vi "Telemetry.vi"() -> ()   [LabVIEW 2017]
uses:
  <vilib>/Platform/TimedLoop/XDataNode/timing_clust.ctl
  <vilib>/Platform/TimedLoop/XDataNode/nitl_modes.ctl
  <vilib>/Platform/TimedLoop/XDataNode/wakeup.ctl
  <vilib>/nican/nican.llb/ncNetAttr.ctl
  <vilib>/Utility/file.llb/Read From Spreadsheet File (string).vi
  <vilib>/xnet/xnet.llb/XNET Create Session (Frame Input Stream).vi
  <vilib>/xnet/xnet.llb/XNET Read (Frame CAN).vi
  <vilib>/Utility/file.llb/Write To Spreadsheet File (string).vi
  <vilib>/Platform/TimedLoop/XDataNode/XDataNode.xnode
  <resource>/objmgr/xnet.rc
  <vilib>/Platform/TimedLoop/XDataNode/XDNodeRunTimeDep.lvlib
panel:
  out "Traction Control ON":bool
  out "Torque Demand [Nm]":dbl
  out "BP_rear":i16
  out "BP_front":i16
  out "Front / Rear Brake Pressure":cluster{u16, u16}
  out "Regbrake Front Sum [Nm]":dbl
  out "Regbrake Rear Sum [Nm]":dbl
  out "BrakeForce":u16
  out "Cones3 2":T1(array[cluster])
  out "Cones2 2":T1(array[cluster])
  out "Cones1 2":T1(array[cluster])
  out "(hi.lo) 3":u64 format="%064b"
  out "Cones3":T1(array[cluster])
  out "(hi.lo) 2":u64 format="%064b"
  out "Cones2":T1(array[cluster])
  in  "ConeType":cluster{"Col":dbl, "X":dbl, "Y":dbl}
  out "(hi.lo)":u64 format="%064b"
  out "Cones1":T1(array[cluster])
  out "IGBT Temperature":T2(graph)
  out "Numeric 2":u8
  out "Slope":u16
  out "Damper Travel FR [mm]":dbl
  out "Damper Travel RR [mm]":dbl
  out "Damper Travel FL [mm]":dbl
  in  "Wheel Travel FR":dbl=1000.0
  in  "Wheel Travel FL Offset":dbl=1000.0
  in  "Wheel Travel RR Offset":dbl=1000.0
  out "Damper Travel RL [mm]":dbl
  in  "Wheel Travel RL Offset":dbl=1000.0
  out "HV Cell Voltage":u16(graph)
  out "accY 2":dbl
  out "accZ 2":dbl
  out "TorqRaw 2":u16
  in  "Brake Min 3":dbl=426.0
  out "BPRV":bool
  out "BPFV":bool
  out "BPFV":bool
  out "BPFSV":bool
  out "STA2":bool
  out "STA1":bool
  out "TPS2V":bool
  out "TPS1V":bool
  out "Apps2":dbl
  out "Apps1":dbl
  out "APPS1":u8(slide) scale=0.0..100.0
  out "APPS2":u8(slide) scale=0.0..100.0
  out "Brake Pedal Fore Supply":dbl
  out "Status LEDs Red":bool[](array[boolean])
  out "Status LEDs Green":bool[](array[boolean])
  out "Numeric":dbl
  out "TCU speed":cluster{dbl, "AccelXRaw":dbl, dbl}(graph)
  out "AccelYRaw":dbl
  out "AccelXRaw":dbl
  in  "Acc Y offset":dbl
  in  "Acc X offset 2":dbl
  in  "OffsetFilter":dbl=0.01
  out "IsStopped":bool
  out "Acc Z 2":dbl
  out "Acc X 2":dbl
  out "Roll 2":dbl
  out "Acc Y 2":dbl
  out "Yaw 2":dbl
  in  "Acc Z offset":dbl
  out "Vel_acc":dbl=-0.0098098
  in  "New Lap":bool
  out "Energy":dbl[](array[numeric])
  out "Wheel Travel FL":u16
  out "Wheel Travel FR":u16
  out "Wheel Travel RL":u16
  out "Wheel Travel RR":u16
  out "Acc X":dbl
  out "Roll":dbl
  out "Yaw":dbl
  out "Acc Y":dbl
  out "Acc Z":dbl
  out "accY":dbl
  out "accZ":dbl
  out "Intensity Graph":dbl[][](graph)
  in  "Rollrate offset":dbl
  out "XY Graph 2":cluster{dbl[], dbl[]}(graph)
  out "Torq_sum":dbl
  in  "Play":bool
  in  "Timestep":u32
  in  "stop":bool
  in  "start":bool
  in  "pause":bool
  in  "Progress":i32(slide) min=0 step=60 scale=-1.0..61354011.0 scale format="%.0p"
  out "Time Stamp":string="2\r\n60"
  out "Charge Voltage":dbl
  out "Charge Curr":dbl
  in  "Tab Control":T3(tab)
  in  "Rows to read":i32=60
  in  "Data Path":path=path "D:/__BME-FRT/2016/2016-05-19/2016_05_19_tokol_endurance_00005_00001.csv"
  in  "CAN1 Enable":bool
  in  "CAN0 Enable":bool
  in  "Data Source":u16(ring) items=["Wi-Fi", "CAN-USB", "Log Analysis", "XCAN-USB"]
  in  "Port":u16=8998
  in  "Exit":bool
  in  "Log Path":path=path "D:/__BME-FRT/2016/test.txt"
  in  "Log Enable":bool
  out "WiFi Error":errorcluster
  in  "Length":u16=10
  out "CAN0 Error":errorcluster
  out "CAN1 Error":errorcluster
  out "Log Error":errorcluster
  out "CAN Message":u8[][](array[numeric])=[[2, 1, 128, 63, 0, 0, 129, 162, 129, 155], [2, 17, 23, 61, 0, 1, 0, 0, 0, 0], [3, 64, 252, 0, 0, 0, 27, 55, 27, 0], [2, 16, 115, 16, 37, 0, 203, 0, 0, 0], [4, 17, 23, 61, 0, 1, 0, 0, 0, 0], [2, 0, 128, 44, 0, 0, 136, 1, 7, 207], [2, 1, 128, 63, 0, 0, 129, 162, 129, 155], [2, 17, 23, 61, 0, 1, 0, 0, 0, 0], [4, 34, 0, 33, 0, 30, 0, 0, 0, 0], [4, 80, 148, 60, 128, 0, 0, 0, 0, 0], [1, 116, 84, 128, 0, 0, 190, 127, 8, 37], [2, 16, 116, 15, 111, 0, 203, 0, 0, 0], [1, 120, 211, 127, 0, 0, 193, 158, 8, 215], [1, 180, 84, 128, 0, 0, 223, 126, 2, 100], [1, 124, 0, 0, 0, 0, 189, 126, 8, 75], [1, 184, 62, 128, 2, 15, 59, 127, 2, 219], [4, 17, 23, 61, 0, 1, 0, 0, 0, 0], [1, 188, 0, 0, 0, 0, 136, 158, 2, 110], [2, 0, 128, 44, 0, 0, 136, 1, 7, 207], [2, 1, 128, 63, 0, 0, 129, 162, 129, 155], [2, 17, 23, 61, 0, 1, 0, 0, 0, 0], [3, 64, 252, 0, 0, 0, 27, 55, 27, 0], [4, 48, 10, 15, 219, 0, 96, 0, 0, 0], [3, 49, 128, 255, 0, 0, 0, 0, 0, 0], [2, 16, 117, 0, 0, 0, 203, 0, 0, 0], [4, 17, 23, 61, 0, 1, 0, 0, 0, 0], [2, 0, 128, 44, 0, 0, 136, 1, 7, 207], [2, 1, 128, 63, 0, 0, 129, 162, 129, 155], [2, 17, 23, 61, 0, 1, 0, 0, 0, 0], [3, 32, 112, 255, 0, 0, 0, 0, 0, 0], [4, 34, 0, 30, 0, 31, 0, 0, 0, 0], [1, 116, 87, 128, 0, 0, 184, 127, 9, 218], [1, 120, 203, 127, 1, 37, 194, 158, 9, 222], [2, 16, 118, 0, 0, 0, 205, 0, 0, 0], [1, 124, 0, 0, 0, 0, 176, 126, 9, 211], [1, 180, 90, 128, 0, 0, 215, 126, 3, 116], [1, 184, 50, 128, 3, 19, 44, 127, 3, 114], [4, 17, 23, 61, 0, 1, 0, 0, 0, 0], [1, 188, 0, 0, 0, 0, 147, 158, 3, 235], [2, 0, 128, 43, 0, 0, 136, 1, 7, 207], [2, 1, 128, 63, 0, 0, 129, 162, 129, 155], [2, 17, 23, 61, 0, 1, 0, 0, 0, 0], [3, 64, 252, 0, 0, 0, 38, 55, 38, 0], [2, 16, 119, 0, 0, 0, 202, 0, 0, 0], [4, 17, 23, 61, 0, 1, 0, 0, 0, 0], [2, 0, 128, 43, 0, 0, 136, 2, 7, 207], [2, 1, 128, 63, 0, 0, 129, 162, 129, 155], [2, 17, 23, 61, 0, 1, 0, 0, 0, 0], [4, 34, 0, 20, 0, 26, 0, 0, 0, 0], [1, 116, 78, 128, 0, 0, 179, 127, 10, 75], [1, 120, 206, 127, 2, 57, 194, 158, 10, 132], [2, 16, 120, 16, 37, 0, 200, 0, 210, 0], [1, 180, 90, 128, 0, 0, 206, 126, 4, 188], [1, 124, 0, 0, 0, 0, 157, 126, 10, 65], [1, 184, 39, 128, 4, 3, 33, 127, 4, 7], [4, 17, 23, 61, 0, 1, 0, 0, 0, 0], [1, 188, 0, 0, 0, 0, 153, 158, 4, 183], [2, 0, 128, 43, 0, 0, 136, 2, 7, 207], [2, 1, 128, 63, 0, 0, 129, 162, 129, 155], [2, 17, 23, 61, 0, 1, 0, 0, 0, 0]] format="%02x"
  out "CAN ID":u16[](array[numeric])=[513, 529, 832, 528, 1041, 512, 513, 529, 1058, 1104, 372, 528, 376, 436, 380, 440, 1041, 444, 512, 513, 529, 832, 1072, 817, 528, 1041, 512, 513, 529, 800, 1058, 372, 376, 528, 380, 436, 440, 1041, 444, 512, 513, 529, 832, 528, 1041, 512, 513, 529, 1058, 372, 376, 528, 436, 380, 440, 1041, 444, 512, 513, 529] format="%x"
  out "CAN Message 2":u8[][](array[numeric])=[[2, 1, 128, 63, 0, 0, 129, 162, 129, 155], [2, 17, 23, 61, 0, 1, 0, 0, 0, 0], [3, 64, 252, 0, 0, 0, 27, 55, 27, 0], [2, 16, 115, 16, 37, 0, 203, 0, 0, 0], [4, 17, 23, 61, 0, 1, 0, 0, 0, 0], [2, 0, 128, 44, 0, 0, 136, 1, 7, 207], [2, 1, 128, 63, 0, 0, 129, 162, 129, 155], [2, 17, 23, 61, 0, 1, 0, 0, 0, 0], [4, 34, 0, 33, 0, 30, 0, 0, 0, 0], [4, 80, 148, 60, 128, 0, 0, 0, 0, 0], [1, 116, 84, 128, 0, 0, 190, 127, 8, 37], [2, 16, 116, 15, 111, 0, 203, 0, 0, 0], [1, 120, 211, 127, 0, 0, 193, 158, 8, 215], [1, 180, 84, 128, 0, 0, 223, 126, 2, 100], [1, 124, 0, 0, 0, 0, 189, 126, 8, 75], [1, 184, 62, 128, 2, 15, 59, 127, 2, 219], [4, 17, 23, 61, 0, 1, 0, 0, 0, 0], [1, 188, 0, 0, 0, 0, 136, 158, 2, 110], [2, 0, 128, 44, 0, 0, 136, 1, 7, 207], [2, 1, 128, 63, 0, 0, 129, 162, 129, 155], [2, 17, 23, 61, 0, 1, 0, 0, 0, 0], [3, 64, 252, 0, 0, 0, 27, 55, 27, 0], [4, 48, 10, 15, 219, 0, 96, 0, 0, 0], [3, 49, 128, 255, 0, 0, 0, 0, 0, 0], [2, 16, 117, 0, 0, 0, 203, 0, 0, 0], [4, 17, 23, 61, 0, 1, 0, 0, 0, 0], [2, 0, 128, 44, 0, 0, 136, 1, 7, 207], [2, 1, 128, 63, 0, 0, 129, 162, 129, 155], [2, 17, 23, 61, 0, 1, 0, 0, 0, 0], [3, 32, 112, 255, 0, 0, 0, 0, 0, 0], [4, 34, 0, 30, 0, 31, 0, 0, 0, 0], [1, 116, 87, 128, 0, 0, 184, 127, 9, 218], [1, 120, 203, 127, 1, 37, 194, 158, 9, 222], [2, 16, 118, 0, 0, 0, 205, 0, 0, 0], [1, 124, 0, 0, 0, 0, 176, 126, 9, 211], [1, 180, 90, 128, 0, 0, 215, 126, 3, 116], [1, 184, 50, 128, 3, 19, 44, 127, 3, 114], [4, 17, 23, 61, 0, 1, 0, 0, 0, 0], [1, 188, 0, 0, 0, 0, 147, 158, 3, 235], [2, 0, 128, 43, 0, 0, 136, 1, 7, 207], [2, 1, 128, 63, 0, 0, 129, 162, 129, 155], [2, 17, 23, 61, 0, 1, 0, 0, 0, 0], [3, 64, 252, 0, 0, 0, 38, 55, 38, 0], [2, 16, 119, 0, 0, 0, 202, 0, 0, 0], [4, 17, 23, 61, 0, 1, 0, 0, 0, 0], [2, 0, 128, 43, 0, 0, 136, 2, 7, 207], [2, 1, 128, 63, 0, 0, 129, 162, 129, 155], [2, 17, 23, 61, 0, 1, 0, 0, 0, 0], [4, 34, 0, 20, 0, 26, 0, 0, 0, 0], [1, 116, 78, 128, 0, 0, 179, 127, 10, 75], [1, 120, 206, 127, 2, 57, 194, 158, 10, 132], [2, 16, 120, 16, 37, 0, 200, 0, 210, 0], [1, 180, 90, 128, 0, 0, 206, 126, 4, 188], [1, 124, 0, 0, 0, 0, 157, 126, 10, 65], [1, 184, 39, 128, 4, 3, 33, 127, 4, 7], [4, 17, 23, 61, 0, 1, 0, 0, 0, 0], [1, 188, 0, 0, 0, 0, 153, 158, 4, 183], [2, 0, 128, 43, 0, 0, 136, 2, 7, 207], [2, 1, 128, 63, 0, 0, 129, 162, 129, 155], [2, 17, 23, 61, 0, 1, 0, 0, 0, 0]] format="%02x"
  out "CAN ID 2":u16[](array[numeric])=[513, 529, 832, 528, 1041, 512, 513, 529, 1058, 1104, 372, 528, 376, 436, 380, 440, 1041, 444, 512, 513, 529, 832, 1072, 817, 528, 1041, 512, 513, 529, 800, 1058, 372, 376, 528, 380, 436, 440, 1041, 444, 512, 513, 529, 832, 528, 1041, 512, 513, 529, 1058, 372, 376, 528, 436, 380, 440, 1041, 444, 512, 513, 529] format="%x"
  out "CAN Message 3":u8[][](array[numeric])=[[2, 1, 128, 63, 0, 0, 129, 162, 129, 155], [2, 17, 23, 61, 0, 1, 0, 0, 0, 0], [3, 64, 252, 0, 0, 0, 27, 55, 27, 0], [2, 16, 115, 16, 37, 0, 203, 0, 0, 0], [4, 17, 23, 61, 0, 1, 0, 0, 0, 0], [2, 0, 128, 44, 0, 0, 136, 1, 7, 207], [2, 1, 128, 63, 0, 0, 129, 162, 129, 155], [2, 17, 23, 61, 0, 1, 0, 0, 0, 0], [4, 34, 0, 33, 0, 30, 0, 0, 0, 0], [4, 80, 148, 60, 128, 0, 0, 0, 0, 0], [1, 116, 84, 128, 0, 0, 190, 127, 8, 37], [2, 16, 116, 15, 111, 0, 203, 0, 0, 0], [1, 120, 211, 127, 0, 0, 193, 158, 8, 215], [1, 180, 84, 128, 0, 0, 223, 126, 2, 100], [1, 124, 0, 0, 0, 0, 189, 126, 8, 75], [1, 184, 62, 128, 2, 15, 59, 127, 2, 219], [4, 17, 23, 61, 0, 1, 0, 0, 0, 0], [1, 188, 0, 0, 0, 0, 136, 158, 2, 110], [2, 0, 128, 44, 0, 0, 136, 1, 7, 207], [2, 1, 128, 63, 0, 0, 129, 162, 129, 155], [2, 17, 23, 61, 0, 1, 0, 0, 0, 0], [3, 64, 252, 0, 0, 0, 27, 55, 27, 0], [4, 48, 10, 15, 219, 0, 96, 0, 0, 0], [3, 49, 128, 255, 0, 0, 0, 0, 0, 0], [2, 16, 117, 0, 0, 0, 203, 0, 0, 0], [4, 17, 23, 61, 0, 1, 0, 0, 0, 0], [2, 0, 128, 44, 0, 0, 136, 1, 7, 207], [2, 1, 128, 63, 0, 0, 129, 162, 129, 155], [2, 17, 23, 61, 0, 1, 0, 0, 0, 0], [3, 32, 112, 255, 0, 0, 0, 0, 0, 0], [4, 34, 0, 30, 0, 31, 0, 0, 0, 0], [1, 116, 87, 128, 0, 0, 184, 127, 9, 218], [1, 120, 203, 127, 1, 37, 194, 158, 9, 222], [2, 16, 118, 0, 0, 0, 205, 0, 0, 0], [1, 124, 0, 0, 0, 0, 176, 126, 9, 211], [1, 180, 90, 128, 0, 0, 215, 126, 3, 116], [1, 184, 50, 128, 3, 19, 44, 127, 3, 114], [4, 17, 23, 61, 0, 1, 0, 0, 0, 0], [1, 188, 0, 0, 0, 0, 147, 158, 3, 235], [2, 0, 128, 43, 0, 0, 136, 1, 7, 207], [2, 1, 128, 63, 0, 0, 129, 162, 129, 155], [2, 17, 23, 61, 0, 1, 0, 0, 0, 0], [3, 64, 252, 0, 0, 0, 38, 55, 38, 0], [2, 16, 119, 0, 0, 0, 202, 0, 0, 0], [4, 17, 23, 61, 0, 1, 0, 0, 0, 0], [2, 0, 128, 43, 0, 0, 136, 2, 7, 207], [2, 1, 128, 63, 0, 0, 129, 162, 129, 155], [2, 17, 23, 61, 0, 1, 0, 0, 0, 0], [4, 34, 0, 20, 0, 26, 0, 0, 0, 0], [1, 116, 78, 128, 0, 0, 179, 127, 10, 75], [1, 120, 206, 127, 2, 57, 194, 158, 10, 132], [2, 16, 120, 16, 37, 0, 200, 0, 210, 0], [1, 180, 90, 128, 0, 0, 206, 126, 4, 188], [1, 124, 0, 0, 0, 0, 157, 126, 10, 65], [1, 184, 39, 128, 4, 3, 33, 127, 4, 7], [4, 17, 23, 61, 0, 1, 0, 0, 0, 0], [1, 188, 0, 0, 0, 0, 153, 158, 4, 183], [2, 0, 128, 43, 0, 0, 136, 2, 7, 207], [2, 1, 128, 63, 0, 0, 129, 162, 129, 155], [2, 17, 23, 61, 0, 1, 0, 0, 0, 0]] format="%02x"
  out "CAN ID 3":u16[](array[numeric])=[513, 529, 832, 528, 1041, 512, 513, 529, 1058, 1104, 372, 528, 376, 436, 380, 440, 1041, 444, 512, 513, 529, 832, 1072, 817, 528, 1041, 512, 513, 529, 800, 1058, 372, 376, 528, 380, 436, 440, 1041, 444, 512, 513, 529, 832, 528, 1041, 512, 513, 529, 1058, 372, 376, 528, 436, 380, 440, 1041, 444, 512, 513, 529] format="%x"
  out "Max RPM":u16
  out "Throttle Bias Front":dbl
  out "STA2":i16
  out "STA1":i16
  out "Max Power":u8
  out "TPS1_Raw":u16
  out "BPS1_Raw":u16
  out "Velocity [km/h]":dbl(knob) scale=0.0..120.0
  out "CAN Missing Message":u8[](array[numeric])
  out "TCU FR":dbl(graph)
  out "TCU RR":dbl(graph)
  out "TCU FL":dbl(graph)
  out "Throttle Bias Rear":dbl
  out "Torque":dbl(slide) scale=0.0..100.0
  out "FL":dbl(slide) scale=0.0..2330.0
  in  "Torque Min":dbl
  in  "Torque Max":dbl=1000.0
  in  "Brake Min":dbl
  in  "Brake Max":dbl=1000.0
  out "FL 2":dbl(slide)
  out "FR":dbl(slide) scale=0.0..2330.0
  out "FR 2":dbl(slide)
  out "RL":dbl(slide) scale=0.0..2330.0
  out "RL 2":dbl(slide)
  out "RR":dbl(slide) scale=0.0..2330.0
  out "RR 2":dbl(slide)
  out "Sensor Check":bool[](array[boolean])
  out "Brake Front":dbl(slide)=-0.5082592121982211 scale=0.0..100.0
  out "Brake Rear":dbl(slide)=-0.9529860228716646 scale=0.0..100.0
  in  "Brake Min 2":dbl=460.0
  in  "Brake Max 2":dbl=2000.0
  out "TorqRaw":u16
  out "BrakeRaw 2":u16
  out "Boolean":bool
  out "Boolean 2":bool
  out "Boolean 3":bool
  out "Boolean 4":bool
  out "Dial":dbl(knob)=3.0 scale=1.0..12.0
  out "Dial 2":dbl(knob)=11.0 scale=1.0..12.0
  out "Dial 3":dbl(knob)=9.0 scale=1.0..12.0
  out "Dial 4":dbl(knob)=1.0 scale=1.0..12.0
  out "Dial 5":dbl(knob)=1.0 scale=1.0..12.0
  out "Torque %":u8
  out "Speed [kmph]":dbl
  out "Regen %":u8
  out "BTC":bool
  out "TCU RR Status":bool[](array[boolean])
  out "TCU RL Status":bool[](array[boolean])
  out "TCU FR Status":bool[](array[boolean])
  out "TCU FL Status":bool[](array[boolean])
  out "Torque [Nm]":dbl(knob) scale=-500.0..1250.0
  out "XY Graph":cluster{dbl[], dbl[]}[](graph)
  out "TCU RL":dbl(graph)
  out "BPS2_Raw":u16
  out "BPF_Raw":u16
  out "BPR_Raw":u16
  out "TPS2_Raw":u16
  out "STA2_Raw":u16
  out "STA1_Raw":u16
  out "OFF":bool=TRUE
  out "START":bool
  out "ON":bool
  in  "Steering Null":dbl=1919.0
  in  "Steering Min":dbl=174.0
  in  "Steering Max":dbl=3565.0
  out "Steering Angle":dbl(slide)=-0.10285714285714287 scale=90.0..-90.0
  out "SteeringRaw":u16
  out "Safety Mode Enabled":bool
  out "PPS1":i16
  out "PPS2":i16
  out "Logging":bool
  out "Pressure based":bool
  out "Force based":bool
  out "Brake Force 2":u16
  out "Brake Force":u16(slide) scale=0.0..1500.0
  out "Slip_TCU":cluster{dbl, dbl, dbl, dbl}(graph)
  out "TCU_acc":cluster{dbl[], dbl[]}[](graph)
  out "Slip":cluster{dbl, dbl, dbl, dbl}(graph)
  out "TCU_ay":dbl
  out "TCU_v":dbl
  out "TCU_ax":dbl
  out "TCU_yaw":dbl
  out "TCU_slipFL":dbl
  out "TCU_slipFR":dbl
  out "TCU_slipRL":dbl
  out "TCU_slipRR":dbl
  out "FL Velocity":dbl
  out "FL Torque Pos":dbl
  out "FL Torque Neg":dbl
  out "FR Velocity":dbl
  out "FR Torque Pos":dbl
  out "FR Torque Neg":dbl
  out "RL Velocity":dbl
  out "RL Torque Pos":dbl
  out "RL Torque Neg":dbl
  out "RR Velocity":dbl
  out "RR Torque Pos":dbl
  out "RR Torque Neg":dbl
  out "MCU RR":cluster{dbl, dbl}(graph)={-0.487060546875, 0.57037353515625}
  out "MCU RL":cluster{dbl, dbl}(graph)={0.743408203125, -0.384521484375}
  out "MCU FR":cluster{dbl, dbl}(graph)={-0.25634765625, -0.205078125}
  out "MCU FL":cluster{dbl, dbl}(graph)={-0.16021728515625, 0.50628662109375}
  out "Actual Velocity\nFL [RPM]":i16
  out "Id FL [A]":dbl
  out "Iq FL [A]":dbl
  out "T Motor FL [°C]":dbl
  out "Error Info FL":u16
  out "Actual Velocity\nFR [RPM]":i16
  out "Id FR [A]":dbl
  out "Iq FR [A]":dbl
  out "Actual Velocity\nRL [RPM]":i16
  out "Id RL [A]":dbl
  out "Iq RL [A]":dbl
  out "Actual Velocity \nRR [RPM]":i16
  out "Id RR [A]":dbl
  out "Iq RR [A]":dbl
  out "Error Info FR":u16
  out "T Motor FR [°C]":dbl
  out "Error Info RL":u16
  out "T Motor RL [°C]":dbl
  out "Error Info RR":u16
  out "T Motor RR [°C]":dbl
  out "Status FL":bool[](array[boolean])
  out "Status FR":bool[](array[boolean])
  out "Status RL":bool[](array[boolean])
  out "Status RR":bool[](array[boolean])
  out "T Inv. FL [°C]":dbl
  out "T Inv. FR [°C]":dbl
  out "T Inv. RR [°C]":dbl
  out "T Inv. RL [°C]":dbl
  out "IGBT FL TEMP":i16
  out "IGBT FR TEMP":dbl
  out "IGBT RL TEMP":dbl
  out "IGBT RR TEMP":dbl
  out "MCU SC Endline":bool
  out "HVD Interlock":bool
  out "Motor4 Interlock":bool
  out "Motor3 Interlock":bool
  out "Motor2 Interlock":bool
  out "Motor1 Interlock":bool
  out "SC LKS":bool
  out "SC RKS":bool
  out "SC MCU":bool
  out "SC 12V":bool
  out "SC IMD":bool
  out "SC AMS":bool
  out "SC AIR-":bool
  out "SC AIR+":bool
  out "SC BOTS &\nINS & CKS":bool
  out "SC Motor 3":bool
  out "SC Motor 1":bool
  out "SC Motor 4":bool
  out "SC Motor 2":bool
  out "HVDet":bool
  out "AIR-":bool
  out "AIR+":bool
  out "MCU Interlocks":bool
  out "LKS & RKS":bool
  out "HV_ACC in menu":bool
  out "AMS Relay":bool
  out "IMD Relay":bool
  out "SC Endline":bool
  out "Radiator Cooling":bool
  out "Battery Low":bool
  out "BMS IC Wake":bool
  out "BMS IC Fault":bool
  out "48V Out 5":bool
  out "Battery Full":bool
  out "48V Out 3":bool
  out "48V Out 4":bool
  out "Undervoltage 3":bool
  out "Overtemp. 3":bool
  out "Logging Status":bool
  out "Radio CS":bool
  out "12V Out 2":bool
  out "12V Out 3":bool
  out "SC State":bool
  out "12V Out 1":bool
  out "Main Switch":bool
  out "MP Switch":bool
  out "12V Out 5":bool
  out "12V Out 4":bool
  out "48V Out 2":bool
  out "48V Out 1":bool
  out "Discharge":bool[](array[boolean])
  out "LV Temp":dbl[](array[numeric])
  out "LV Battery":cluster{"CellSlide":u16, "CellVoltage":u16}[](array[cluster])=[{"CellSlide"=0, "CellVoltage"=0}, {"CellSlide"=0, "CellVoltage"=0}, {"CellSlide"=0, "CellVoltage"=0}, {"CellSlide"=0, "CellVoltage"=0}, {"CellSlide"=0, "CellVoltage"=0}, {"CellSlide"=0, "CellVoltage"=0}, {"CellSlide"=0, "CellVoltage"=0}, {"CellSlide"=0, "CellVoltage"=0}, {"CellSlide"=0, "CellVoltage"=0}, {"CellSlide"=2800, "CellVoltage"=0}, {"CellSlide"=0, "CellVoltage"=0}, {"CellSlide"=0, "CellVoltage"=0}, {"CellSlide"=0, "CellVoltage"=0}, {"CellSlide"=0, "CellVoltage"=0}] {"CellSlide" scale=2800.0..4200.0}
  out "LV Temp":dbl
  out "LV Max":u16
  out "LV Min":u16
  out "LV Cell Voltages":T4(graph)
  out "Overtemp Errors":u16
  out "Undervoltage Errrors":u16
  out "LV Current":cluster{dbl, dbl}(graph)
  out "LV Voltage [V]":dbl format="%#.2g"
  out "12V Current [A]":dbl format="%#.1g"
  out "48V Current [A]":dbl format="%#.1g"
  out "Temp Max 2":dbl
  out "Cell Min 2":u16
  out "HVDet":bool
  out "Stack 1":cluster{"CellSlide":u16, "CellVoltage":u16}[](array[cluster]) {"CellSlide" scale=2800.0..4200.0}
  out "Temp 1":dbl[](array[numeric])
  out "Cell Min":u16
  out "Cell Max":u16
  out "Temp Max":dbl
  out "HV Before":dbl
  out "HV After":dbl
  out "HV Current":dbl
  out "SoC [mAh]":dbl
  out "Stack 2":cluster{"CellSlide":u16, "CellVoltage":u16}[](array[cluster]) {"CellSlide" scale=2800.0..4200.0}
  out "Stack 3":cluster{"CellSlide":u16, "CellVoltage":u16}[](array[cluster]) {"CellSlide" scale=2800.0..4200.0}
  out "Stack 4":cluster{"CellSlide":u16, "CellVoltage":u16}[](array[cluster])=[{"CellSlide"=0, "CellVoltage"=0}, {"CellSlide"=0, "CellVoltage"=0}, {"CellSlide"=0, "CellVoltage"=0}, {"CellSlide"=0, "CellVoltage"=0}, {"CellSlide"=0, "CellVoltage"=0}, {"CellSlide"=0, "CellVoltage"=0}, {"CellSlide"=0, "CellVoltage"=0}, {"CellSlide"=0, "CellVoltage"=0}, {"CellSlide"=0, "CellVoltage"=0}, {"CellSlide"=0, "CellVoltage"=0}, {"CellSlide"=0, "CellVoltage"=0}, {"CellSlide"=0, "CellVoltage"=0}, {"CellSlide"=0, "CellVoltage"=0}, {"CellSlide"=0, "CellVoltage"=0}, {"CellSlide"=0, "CellVoltage"=0}, {"CellSlide"=0, "CellVoltage"=0}, {"CellSlide"=0, "CellVoltage"=0}, {"CellSlide"=0, "CellVoltage"=0}, {"CellSlide"=0, "CellVoltage"=0}, {"CellSlide"=0, "CellVoltage"=0}, {"CellSlide"=0, "CellVoltage"=0}, {"CellSlide"=0, "CellVoltage"=0}, {"CellSlide"=2800, "CellVoltage"=0}, {"CellSlide"=2800, "CellVoltage"=0}] {"CellSlide" scale=2800.0..4200.0}
  out "Stack 5":cluster{"CellSlide":u16, "CellVoltage":u16}[](array[cluster])=[{"CellSlide"=2800, "CellVoltage"=0}, {"CellSlide"=0, "CellVoltage"=0}, {"CellSlide"=0, "CellVoltage"=0}, {"CellSlide"=0, "CellVoltage"=0}, {"CellSlide"=0, "CellVoltage"=0}, {"CellSlide"=0, "CellVoltage"=0}, {"CellSlide"=0, "CellVoltage"=0}, {"CellSlide"=0, "CellVoltage"=0}, {"CellSlide"=0, "CellVoltage"=0}, {"CellSlide"=0, "CellVoltage"=0}, {"CellSlide"=0, "CellVoltage"=0}, {"CellSlide"=0, "CellVoltage"=0}, {"CellSlide"=0, "CellVoltage"=0}, {"CellSlide"=0, "CellVoltage"=0}, {"CellSlide"=0, "CellVoltage"=0}, {"CellSlide"=0, "CellVoltage"=0}, {"CellSlide"=0, "CellVoltage"=0}, {"CellSlide"=0, "CellVoltage"=0}, {"CellSlide"=0, "CellVoltage"=0}, {"CellSlide"=0, "CellVoltage"=0}, {"CellSlide"=0, "CellVoltage"=0}, {"CellSlide"=0, "CellVoltage"=0}, {"CellSlide"=0, "CellVoltage"=0}, {"CellSlide"=0, "CellVoltage"=0}] {"CellSlide" scale=2800.0..4200.0}
  out "Stack 6":cluster{"CellSlide":u16, "CellVoltage":u16}[](array[cluster]) {"CellSlide" scale=2800.0..4200.0}
  out "Temp 2":dbl[](array[numeric])
  out "Temp 3":dbl[](array[numeric])
  out "Temp 4":dbl[](array[numeric])
  out "Temp 5":dbl[](array[numeric])
  out "Temp 6":dbl[](array[numeric])
  out "TSAL State":bool
  out "PC State":bool
  out "12V State":bool
  out "AMS error":bool
  out "IMD error":bool
  out "AMS Relay 2":bool
  out "IMD Relay":bool
  out "AIR+":bool
  out "AIR-":bool
  out "UV":bool
  out "OV":bool
  out "OT":bool
  out "TS-OV":bool
  out "Place of Error":u16
  out "Value":u16
  out "TSAL Green":bool
  out "TSAL Red":bool
  out "MCU HVDET":bool
  out "TSAL Error":bool
  out "TS-OC":bool
  out "PC":bool
  out "?":T5(graph)
  out "Angular Speed":T6(graph)
  out "Pedal Signals":cluster{u16, "BrakeRaw":u16}(graph)
  out "Brake Pressure":T7(graph)
  out "XY Graph 3":cluster{dbl[], dbl[]}[](graph)
  out "HV Cell":cluster{"Cell Max":u16, "Cell Min":u16}(graph)
  out "Current":dbl(graph)
  out "Electric Power":cluster{dbl, dbl}(graph)
  out "HV Voltage":cluster{"HV Before":dbl, "HV After":dbl}(graph)={"HV Before"=594.9, "HV After"=0.1}
  out "HV Cell Temperature":cluster{dbl, dbl}(graph)
  out "Motor Temperature":cluster{dbl, dbl, dbl, dbl}(graph)={1.3, 1.3, 1.6, 1.5}
  out "Inverter Temperature":cluster{dbl, dbl, dbl, dbl}(graph)={1.3, 1.3, 1.6, 1.5}
  out "Radiator Temperature":cluster{dbl, dbl, dbl, dbl}(graph)={1.3, 1.3, 1.6, 1.5}
  out "Dash Heartbeat":dbl
  out "Overvoltage":bool
  out "MODE":bool
  out "XLAT":bool
  out "BLANK":bool
  out "MCU S SC Endl":u16
  out "SD CS":bool
  out "Radio CS":bool
  out "XBee CS":bool
  out "TSAL":bool
  out "Logging":bool
  out "OFF":bool
  out "START":bool
  out "24V rear DC/DC":bool
  out "OFF Button":bool
  out "START Button":bool
  out "ON Button":bool
  out "Power B Current":u32
  out "Power A Current":u32
  out "CAN2 Term.":bool
  out "CAN1 Term.":bool
  out "MCU TSAL":bool
  out "MCU SC Endline 2":bool
  out "MCU FL 4":bool
  out "MCU FL 3":bool
  out "MCU FL 2":bool
  out "Brake Heartbeat":bool
  out "MCU RF 4":bool
  out "MCU RF 3":bool
  out "MCU RF 2":bool
  out "MCU RF 1":bool
  out "MCU EF2 B":bool
  out "MCU EF2 A":bool
  out "MCU EF B":bool
  out "MCU EF A":bool
  out "24V Power B":bool
  out "Braking":bool
  out "STA2 ADC Null":u16
  out "STA1 ADC Null":u16
  out "Battery Low 2":bool
  out "BMS IC Awake":bool
  out "BMS IC Error":bool
  out "48V Out 5 2":bool
  out "Battery Full 2":bool
  out "48V Out 3 2":bool
  out "48V Out 4 2":bool
  out "Undervoltage 4":bool
  out "Overtemp. 4":bool
  out "Logging Status":bool
  out "Radio CS":bool
  out "12V Out 2 2":bool
  out "12V Out 3 2":bool
  out "SC State 2":bool
  out "12V Out 1 2":bool
  out "Main Switch 2":bool
  out "MP Switch 2":bool
  out "12V Out 5 2":bool
  out "12V Out 4 2":bool
  out "48V Out 2 2":bool
  out "48V Out 1 2":bool
  out "ON":bool
  out "24V front DC/DC":bool
  out "MCU Interlock":bool
  out "TCU Power":bool
  out "RTDS":bool
  out "LKS & RKS":bool
  out "Brake Light":bool
  out "STA2 ADC 90":u16
  out "STA1 ADC 90":u16
  out "BSE2 ADC Max":u16
  out "BSE2 ADC Min":u16
  out "BSE1 ADC Max":u16
  out "BSE1 ADC Min":u16
  out "APPS2 ADC Max":u16
  out "APPS2 ADC Min":u16
  out "APPS1 ADC Max":u16
  out "APPS1 ADC Min":u16
  out "MCU EF":bool
  out "MCU RF":bool
  out "Radiator Left IN":dbl
  out "Radiator Right OUT":dbl
  out "Radiator Right IN":dbl
  out "Radiator Left OUT":dbl
  out "TSAL State 2":bool
  out "PC State 2":bool
  out "Driver Protection":bool
  out "12V Current [mA]":dbl
  out "48V Current [mA]":dbl
  out "Pedal Heartbeat":dbl
  out "Sensorbox Front Timeout Error":bool
  out "AccY Rear Validity Error":bool
  out "Yaw Rate Rear Validity Error":bool
  out "AccX Rear Validity Error":bool
  out "Sensorbox Front Timeout Error  2":bool
  out "Yaw Rate Front Validity Error":bool
  out "AccY Front Validity Error":bool
  out "AccX Front Validity Error":bool
  out "Steering Angle 1 Validity Error":bool
  out "Steering Angle Plausibility Error":bool
  out "APPS2 Validity Error":bool
  out "APPS1 Validity Error":bool
  out "APPS Plausibility Error":bool
  out "Yaw Rate Plausibility Error":bool
  out "AccY Plausibility Error":bool
  out "AccX Plausibility Error":bool
  out "SC Endline Validity Error":bool
  out "Brake Pressure Timeout Error":bool
  out "Brake Pressure Rear Validity Error":bool
  out "Brake Pressure Front Validity Error":bool
  out "Brake Force Timeout Error":bool
  out "Brake Force Validity Error":bool
  out "Steering APPS Timeout Error":bool
  out "Steering Angle 2 Validity Error":bool
  out "Button 2 Validity Error":bool
  out "Button 1 Validity Error":bool
  out "Rot Switch 5 Validity Error":bool
  out "Rot Switch 4 Validity Error":bool
  out "Rot Switch 3 Validity Error":bool
  out "Rot Switch 2 Validity Error":bool
  out "Rot Switch 1 Validity Error":bool
  out "SC Endline Timeout Error":bool
  out "HV Voltage Validity Error":bool
  out "HV Current Validity Error":bool
  out "HV Cell Values Timeout Error":bool
  out "HV Cell Voltage Validity Error":bool
  out "HV Cell Temperature Validity Error":bool
  out "Steering Control Timeout Error":bool
  out "Button 4 Validity Error":bool
  out "Button 3 Validity Error":bool
  out "LV Cell Values Timeout Error":bool
  out "LV Cell Voltage Validity Error":bool
  out "LV Cell Temperature Validity Error":bool
  out "HV Battery Status Timeout Error":bool
  out "Yaw Control":dbl
  out "New Drop":dbl
  out "PowerLimiter Approx":u16
  out "Hardcore Powlim":bool
  out "New Drop":bool
  out "Drop":dbl
  out "Torque Based Powlim":bool
  out "Throttle Based Powlim":bool
  out "Yaw Rear":dbl(graph)
  out "Yaw Front":dbl(graph)
  out "Slip":dbl(graph)
  out "Characteristics Approx":u8
  out "Tune":dbl
  out "Wheel Travel":cluster{"y_":dbl, "y_":dbl, "y_":dbl, "y_":dbl}(graph)
  out "Fz_FR":u16
  out "Fz_RL":u16
  out "Fz_FL":u16
  out "Fz_RR":u16
  out "YawControlSelector":u16
  out "P tag":u16
  out "Yaw_Control_ON":bool
  out "M_COG_Limit":u16
  out "M Yaw [Nm]":i16
  out "LaunchControl_Mu":dbl
  out "Brake Force Threshold":u16
  out "TC Threshold":u8
  out "Rear_Reduction":dbl format="%.2f"
  out "LaunchControl_Active":bool
  out "TC Normalizer":u16
  out "SlipControl_Enabled":bool
  out "Target pos [°]":ext
  out "ASSI":T8(ring)
  out "EBS":T9(ring)
  out "AMI":T10(ring)
  out "ASMS":u8
  out "RES EBS":bool
  out "RES GO":bool
  out "RES BUTTON":bool
  out "Steering Angle":T11(graph)
  out "Actual pos [°]":ext
  out "Voltage enabled":bool
  out "Fault present":bool
  out "Operation enable":bool
  out "Switched on":bool
  out "Ready to switch on":bool
  out "Warning present":bool
  out "Switch on disabled":bool
  out "In operational NMT state":bool
  out "Target reached":bool
  out "Following error":bool
  out "Setpoint ack":bool
  out "Position referenced to home position":bool
  out "Actual pos [°] Maxon":ext
  out "Voltage Limit":dbl
  out "Current Limit":dbl
  # "SlipControl"
  # "HV    LV BPSD IMD AMS  FL    FR    RL   RR"
  # "SystemReady : 1 ha van 24V és felállt a belsõ rendszer\nError : 1 ha valamilyen error van\nWarn : 1 ha warning van\nQuitDcOn : DcOn visszajelzõje, hogy ténylegesen engedélyezte-e a HV-t, és hogy van is HV\nDcOn : TCU küldi CAN-en, hogy engedélyezze a HV bemenetet, CAN-en beolvasott értéket írja itt ki\nQuitInverterOn : az inverterek tényleges állapota, 1 ha aktívak, azaz a fizikai engedélyezõ jelek is aktívak\nInverterOn : TCU küldi, inverter engedélyezõ jel, azt küldi amit CAN-rõl beolvasott\nDerating : valamilyen derating állapotban van"
  # "Wi-Fi"
  # "CAN-USB"
  # "Log Analysis"
  # "TPS1"
  # "STA1"
  # "TPS2"
  # "STA1"
  # "STA2"
  # "STA2"
  # "BPS1"
  # "STA1 raw"
  # "Throttle Bias"
  # "BPS2"
  # "BPF"
  # "STA2 raw"
  # "BPR"
  # "InverterOn"
  # "InverterOn"
  # "InverterOn"
  # "InverterOn"
  # "DcOn"
  # "DcOn"
  # "DcOn"
  # "DcOn"
  # "Enable"
  # "Enable"
  # "Enable"
  # "Enable"
  # "ErrorReset"
  # "ErrorReset"
  # "ErrorReset"
  # "ErrorReset"
  # "SysReady"
  # "SysReady"
  # "SysReady"
  # "SysReady"
  # "Error"
  # "Error"
  # "Error"
  # "Error"
  # "Warn"
  # "Warn"
  # "Warn"
  # "Warn"
  # "QuitDcOn"
  # "QuitDcOn"
  # "QuitDcOn"
  # "QuitDcOn"
  # "DcOn"
  # "DcOn"
  # "DcOn"
  # "DcOn"
  # "QuitInvOn"
  # "QuitInvOn"
  # "QuitInvOn"
  # "QuitInvOn"
  # "InverterOn"
  # "InverterOn"
  # "InverterOn"
  # "InverterOn"
  # "Derating"
  # "Derating"
  # "Derating"
  # "Derating"
  # "HV Accumulator ECU"
  # "Pedalbox"
  # "LV Sys ECU"
  # "MCU Power ECU"
  # "MCU Support ECU"
  # "Dashboard"
  # "Yaw Control"
  # "Powerlimiter"
  # "Characteristics Approx"
  # "Smooth Transition"
  # "ASSI State"
  # "EBS State"
  # "AMI State"
types:
  T1 = cluster{"Cluster":cluster{"Col":dbl, "X":dbl, "Y":dbl}}[]
  T2 = cluster{"IGBT FL TEMP":i16, "IGBT FR TEMP":dbl, "IGBT RL TEMP":dbl, "IGBT RR TEMP":dbl}
  T3 = enum32{"Config", "Raw Data", "Driver", "TCU", "MCUs", "SC", "LV Accu", "HV Accu", "Dynamics", "Tractive System", "Temperatures", "LV System", "Errors", "Test Settings", "AS"}
  T4 = cluster{"[0]":u16, "[1]":u16, "[2]":u16, "[3]":u16, "[4]":u16, "[5]":u16, "[6]":u16, "[7]":u16, "[8]":u16}
  T5 = cluster{"Velocity [km/h]":dbl, "Torque":dbl, dbl, dbl}
  T6 = cluster{"Actual Velocity (RPM)":i16, "Actual Velocity (RPM) 2":i16, "Actual Velocity (RPM) 3":i16, "Actual Velocity (RPM) 4":i16}
  T7 = cluster{"BP_front":i16, "BP_rear":i16, "Brake Force Threshold":u16, "TC Threshold":u8}
  T8 = enum16{"Invalid", "Off", "Ready", "Driving", "Emergency brake", "Finish", ""}
  T9 = enum16{"Invalid", "Unavailable", "Armed", "Triggered", ""}
  T10 = enum16{"Invalid", "Acceleration", "Skidpad", "Trackdrive", "Braketest", "Inspection", ""}
  T11 = cluster{ext, "Steering Angle":dbl, "Actual pos [°] Maxon":ext}
  T12 = typedef "ncNetAttr.ctl" = cluster{"Start On Open":enum32{"FALSE", "TRUE"}, "Baud Rate":u32, "Read Queue Length":u32, "Write Queue Length":u32, "Standard Comparator":u32, "Standard Mask":u32, "Extended Comparator":u32, "Extended Mask":u32}
  T13 = typedef "xobjhandle.ctl" = u32
  T14 = typedef "XNET Frame CAN.ctl" = cluster{"timestamp":timestamp, "payload":u8[], "identifier":u32, "type":T15, "extended?":bool, "echo?":bool}
  T15 = typedef "XNET Frame Type CAN.ctl" = u8
  T16 = cluster{"ConeType":cluster{"Col":dbl, "X":dbl, "Y":dbl}}[]
  T17 = cluster{"Actual Velocity\nFL [RPM]":i16, "Actual Velocity\nFR [RPM]":i16, "Actual Velocity\nRL [RPM]":i16, "Actual Velocity \nRR [RPM]":i16}
  T18 = cluster{"Regen %":u8, "Characteristics":u8, "Drop Parameter":dbl, "Yaw Control P":u16, "Max Power":u8, "Torque %":u8, "Max RPM":u16, "Regen press":bool, "Regen force":bool, "BTC":bool, "Safety Mode":bool, "Keylock Enable":bool, "Hardcore Powerlimiter On":bool, "Throttle Powerlimiter On":bool, "Torque Powerlimiter On":bool, "New Drop Enabled":bool, "Yaw Control On":bool, "Traction Control On":bool, "Slip Control On":bool, "Launch Control On":bool}
  T19 = cluster{"T Motor FL [°C]":dbl, "T Motor FR [°C]":dbl, "T Motor RL [°C]":dbl, "T Motor RR [°C]":dbl}
  T20 = cluster{"T Inv. FL [°C]":dbl, "T Inv. FR [°C]":dbl, "T Inv. RL [°C]":dbl, "T Inv. RR [°C]":dbl}
  T21 = cluster{"Brake_Force_Max":u16, "Yaw Control Balance":dbl, "M_Yaw_Limit [Nm]":u16, "M_Yaw [Nm]":i16, "Yaw Control Weight":u16, "Brake Force Threshold":u16, "Powlim Approx":u16, "Rear Reduction":dbl, "TC Normalizer":u16, "Drop New":dbl, "Throttle Bias":dbl}
  T22 = cluster{"Sensorbox Front Timeout Error ":bool, "Yaw Rate Rear Validity Error ":bool, "AccY Rear Validity Error":bool, "AccX Rear Validity Error ":bool, "Sensorbox Front Timeout Error  2":bool, "Yaw Rate Front Validity Error":bool, "AccY Front Validity Error":bool, "AccX Front Validity Error":bool, "Steering Angle 1 Validity Error":bool, "Steering Angle Plausibility Error":bool, "APPS2 Validity Error":bool, "APPS1 Validity Error":bool, "APPS Plausibility Error ":bool, "Yaw Rate Plausibility Error ":bool, "AccY Plausibility Error ":bool, "AccX Plausibility Error ":bool, "SC Endline Validity Error":bool, "Brake Pressure Timeout Error ":bool, "Brake Pressure Rear Validity Error":bool, "Brake Pressure Front Validity Error":bool, "Brake Force Timeout Error ":bool, "Brake Force Validity Error ":bool, "Steering APPS Timeout Error":bool, "Steering Angle 2 Validity Error":bool, "Button 2 Validity Error":bool, "Button 1 Validity Error":bool, "Rot Switch 5 Validity Error":bool, "Rot Switch 4 Validity Error":bool, "Rot Switch 3 Validity Error":bool, "Rot Switch 2 Validity Error":bool, "Rot Switch 1 Validity Error":bool, "SC Endline Timeout Error":bool, "HV Voltage Validity Error":bool, "HV Current Validity Error":bool, "HV Cell Values Timeout Error":bool, "HV Cell Voltage Validity Error":bool, "HV Cell Temperature Validity Error":bool, "Steering Control Timeout Error":bool, "Button 4 Validity Error":bool, "Button 3 Validity Error":bool, "LV Cell Values Timeout Error":bool, "LV Cell Voltage Validity Error":bool, "LV Cell Temperature Validity Error":bool, "HV Battery Status Timeout Error":bool}
  T23 = cluster{"Fz RR [N]":u16, "Speed [kmph]":dbl, "Fz FR [N]":u16, "Fz RL [N]":u16, "Torque Demand [Nm]":dbl, "Fz FL [N]":u16, "Regbrake Front Sum [Nm]":dbl, "Regbrake Rear Sum [Nm]":dbl}
  T24 = cluster{"Efficiency Tune":dbl, "TC Threshold":u8, "Launch Control Mu":dbl, "Brake Force Filtered":u16}
  T25 = typedef "XDNodeRunTimeDep.lvlib/timing_clust.ctl" = cluster{"Expected End [f-1]":u64, "Actual End [f-1]":u64, "Finished Late? [f-1]":bool, "Expected End [i-1]":u64, "Actual End [i-1]":u64, "Finished Late? [i-1]":bool, "Expected Start [i]":u64, "Actual Start [i]":u64, "Expected Start [f]":u64, "Actual Start [f]":u64, "Source Name":string, "Structure Name":string, "Period":i64, "Deadline":i64, "Offset":i64, "Start":i64, "Priority":i32, "Timeout":i32, "Mode":T26, "Wakeup Reason":T27, "Error":errorcluster, "Source Type":string, "Secondary Source Type":string, "Global End Time":u64, "Global Start Time":u64, "Frame Duration":u64, "Iteration Duration":u64, "Assigned CPU":i32, "I/O Scan Engine Mode":u32}
  T26 = typedef "XDNodeRunTimeDep.lvlib/nitl_modes.ctl" = enum32{"No Change", "Process missed periods, maintain original phase", "Discard missed periods, maintain original phase", "Process missed periods, ignore original phase", "Discard missed periods, ignore original phase"}
  T27 = typedef "XDNodeRunTimeDep.lvlib/wakeup.ctl" = enum32{"Normal", "Aborted", "Asynchronous wakeup", "Timing source error", "Timed loop error", "Timeout"}
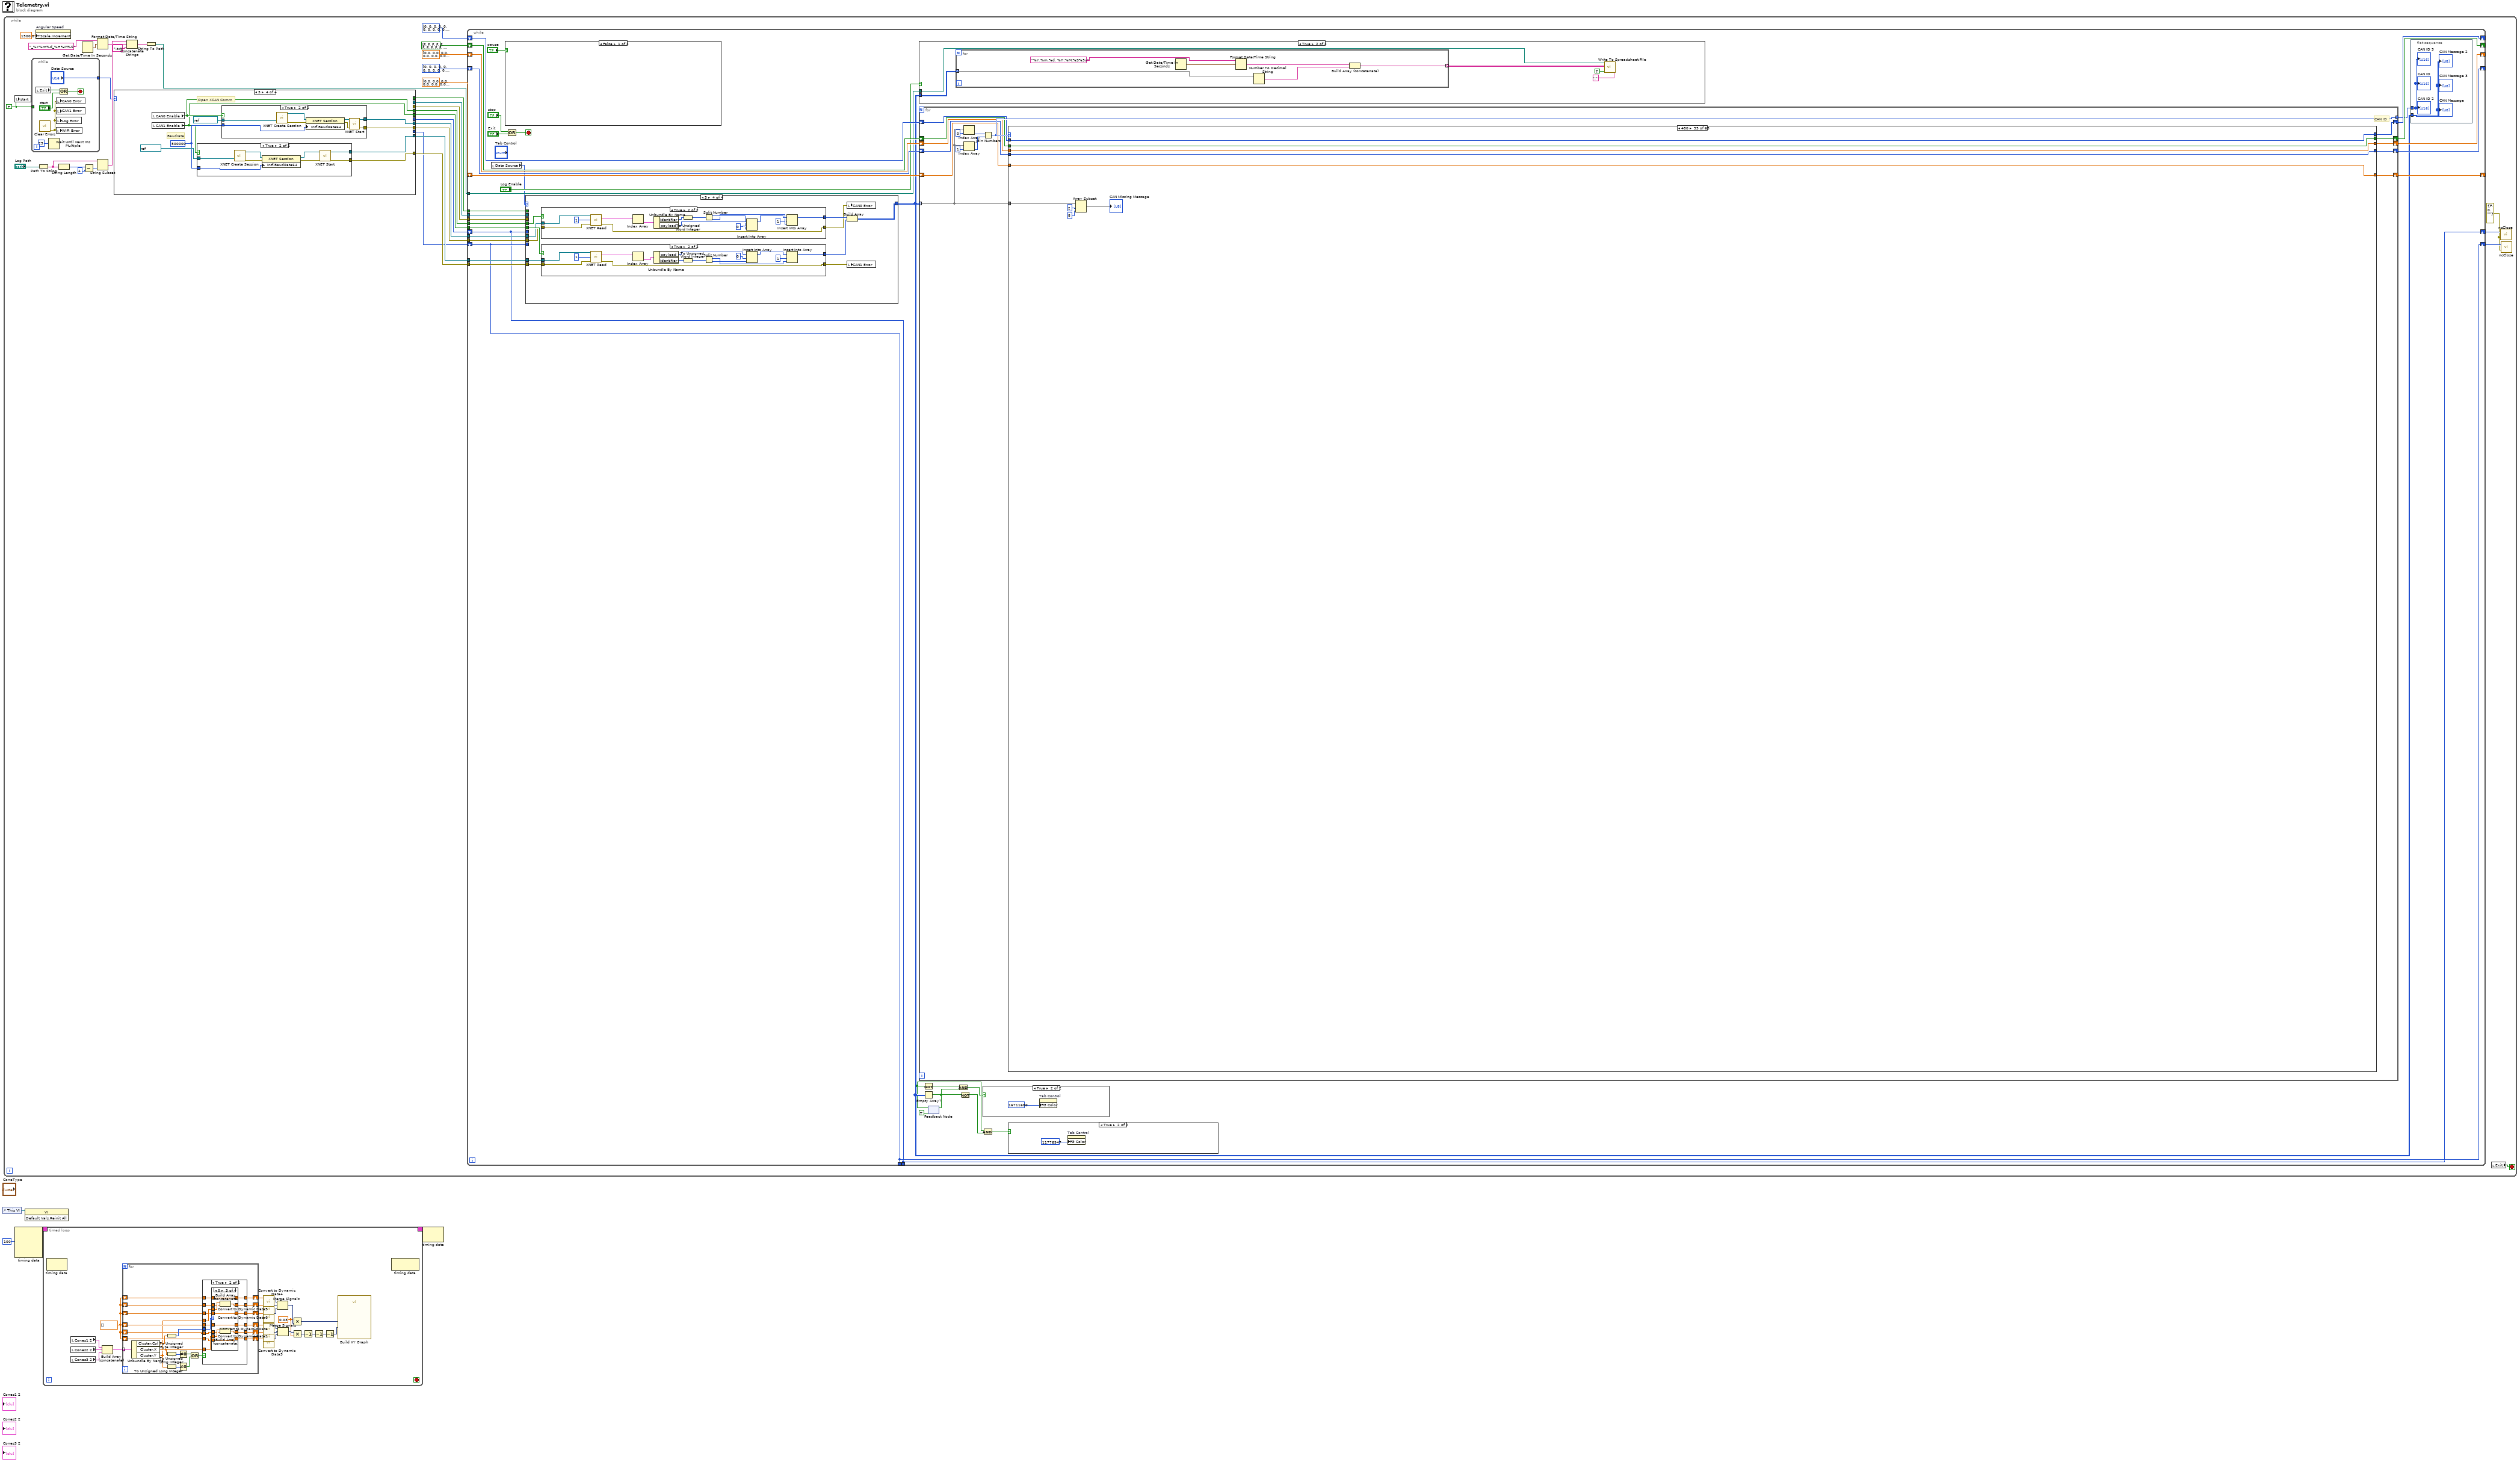
[diagram p0: block diagram]
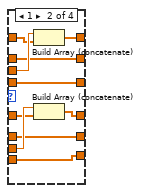
[diagram p4: hidden frame]
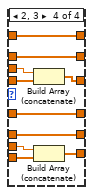
[diagram p5: hidden frame]
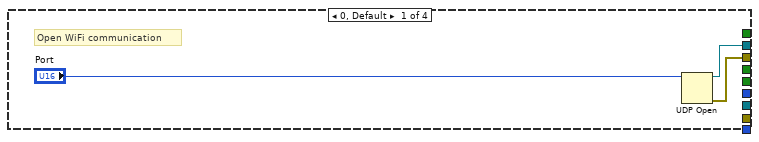
[diagram p6: hidden frame]
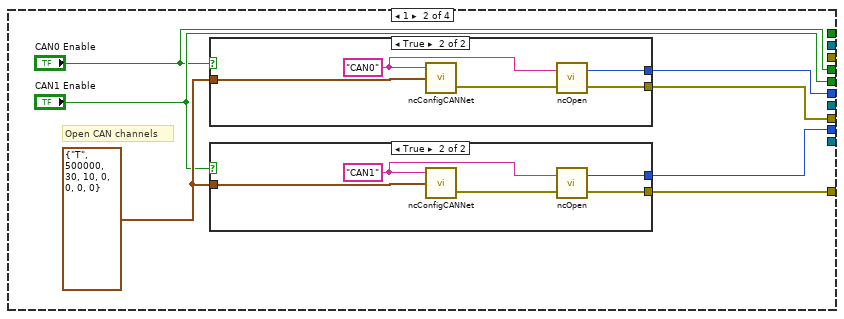
[diagram p7: hidden frame]
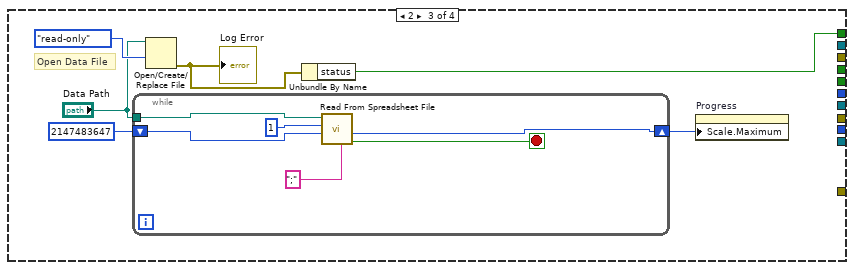
[diagram p10: hidden frame]
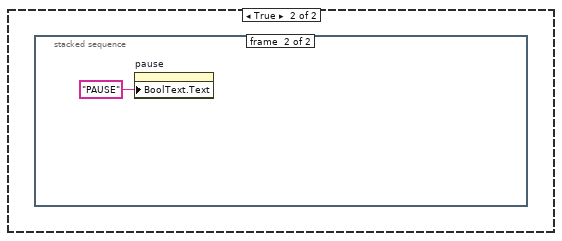
[diagram p13: hidden frame]
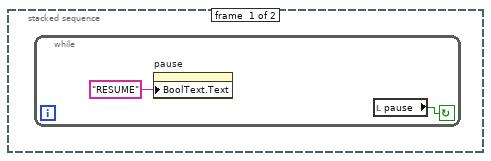
[diagram p14: hidden frame]
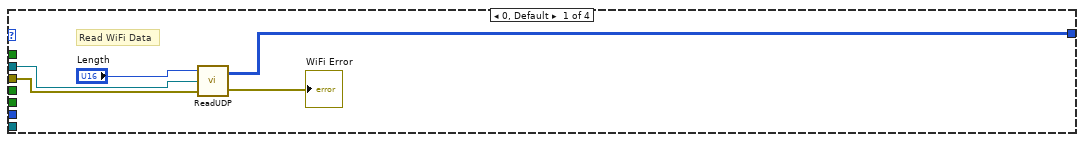
[diagram p17: hidden frame]
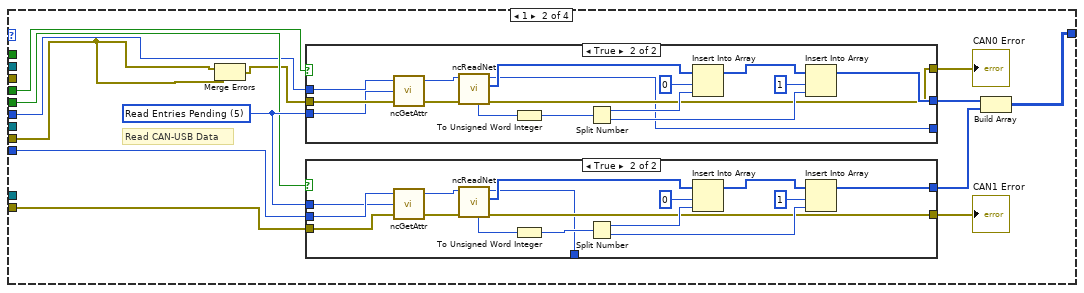
[diagram p18: hidden frame]
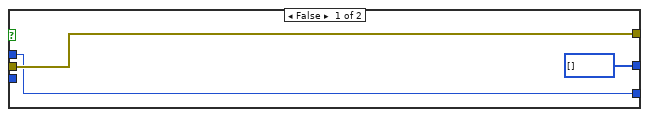
[diagram p19: hidden frame]
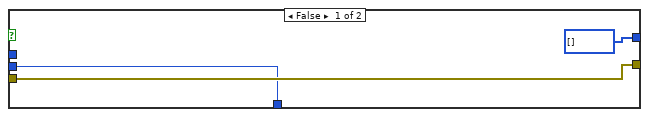
[diagram p20: hidden frame]
diagram:
  n1 = control-ref of="This VI"() -> (w4:refnum<vi>)
  n2 = while {
    stop <- w14 stop-if-true
    w7 = errorcluster {"status"=FALSE, "code"=0, "source"=""} ("Error in")
    w8 = FALSE ("start")
    n3 = local write "start"(w8) -> ()
    n4 = while {
      tunnel: ["Data Source"] -> w15
      tunnel: w8 -> [_]
      stop <- w41 stop-if-true
      n5 = local read "Exit"() -> (w42:bool)
      n6 = call <vilib>:"Clear Errors.vi"() -> ("error out"=w40:errorcluster)  [unwired: 6 in, 1 out]
      n7 = Wait Until Next ms Multiple(millisecond multiple=u32 25) -> ()  [unwired: 1 out]
      n8 = local write "CAN0 Error"(w40) -> ()
      n9 = local write "CAN1 Error"(w40) -> ()
      n10 = local write "Log Error"(w40) -> ()
      n11 = local write "WiFi Error"(w40) -> ()
      n12 = Compound Arithmetic op=OR(w42, "start") -> (w41:bool)
    }
    n13 = property on="Angular Speed" class="WFChart (strict)"("YScale.Increment"=1500.0 ("Y Scale.Range:Increment")) -> ()  [unwired: 2 in, 2 out]
    n14 = Path To String(path="Log Path") -> (string=w31:string)
    n15 = String Length(string=w31) -> (length=w30:i32)
    n16 = Get Date/Time In Seconds() -> (seconds since 1Jan1904=w33:timestamp)
    n17 = Subtract(x=w30, y=4) -> (x-y=w28:i32)
    n18 = Format Date/Time String(time format string (%c)="_%Y%m%d_%H%M%S", seconds (now)=w33) -> (date/time string=w24:string)  [unwired: 1 in]
    n19 = String Subset(string=w31, length (rest)=w28) -> (substring=w25:string)  [unwired: 1 in]
    n20 = case shown="3" w15 {
      tunnel: [_ w55 _ _] -> w6
      tunnel: [_ w54 _ w79] -> w19
      tunnel: [_ w53 _ _] -> w5
      tunnel: [_ w52 _ w78] -> w20
      tunnel: [w47 _ _ _] -> w22
      tunnel: [w46 _ _ _] -> w21
      tunnel: [_ "CAN0 Enable" _ w83] -> w18
      tunnel: [_ "CAN1 Enable" _ w82] -> w17
      tunnel: [_ _ w69 _] -> w16
      tunnel: [_ _ _ w81] -> w12
      tunnel: [_ _ _ w80] -> w11
      frame 0, Default {
        # "Open WiFi communication"
        n21 = UDP Open(11:"Port") -> (port=w47:refnum<k16>, 0:w46:errorcluster)  [unwired: 4 in, 1 out]
      }
      frame 1 {
        w51 = T12 {"Start On Open"=enum."TRUE", "Baud Rate"=500000, "Read Queue Length"=30, "Write Queue Length"=10, "Standard Comparator"=0, "Standard Mask"=0, "Extended Comparator"=0, "Extended Mask"=0} ("CAN Network Interface Config")
        # "Open CAN channels"
        n22 = case shown="True" "CAN0 Enable" {
          tunnel: w51 -> [_ w63]
          tunnel: [_ w62] -> w55
          tunnel: [_ w61] -> w54
          frame False {
          }
          frame True {
            w64 = "CAN0" ("ObjName")
            n23 = call <vilib>:"ncConfigCANNet.vi"("CAN Network Interface Config"=w63, "ObjName"=w64) -> ("Error out"=w65:errorcluster)  [unwired: 3 in]
            n24 = call <vilib>:"ncOpen.vi"("Error in"=w65, "ObjName"=w64) -> ("Error out"=w61:errorcluster, "ObjHandle out"=w62:T13)
          }
        }
        n25 = case shown="True" "CAN1 Enable" {
          tunnel: [_ w58] -> w53
          tunnel: [_ w57] -> w52
          tunnel: w51 -> [_ w56]
          frame False {
          }
          frame True {
            w60 = "CAN1" ("ObjName")
            n26 = call <vilib>:"ncConfigCANNet.vi"("CAN Network Interface Config"=w56, "ObjName"=w60) -> ("Error out"=w59:errorcluster)  [unwired: 3 in]
            n27 = call <vilib>:"ncOpen.vi"("Error in"=w59, "ObjName"=w60) -> ("Error out"=w57:errorcluster, "ObjHandle out"=w58:T13)
          }
        }
      }
      frame 2 {
        # "Open Data File"
        n28 = while {
          tunnel: "Data Path" -> [w77]
          shift-right: [w73] -> w67
          shift-left: 2147483647 ("mark after read (chars.)") -> [w74]
          stop <- w75 stop-if-true
          n29 = call-poly <vilib>:"Read From Spreadsheet File.vi"("delimiter (\\t)"=";" ("delimiter (\\t)"), "start of read offset (chars.:0)"=w74, "number of rows (all:-1)"=1, "file path (dialog if empty)"=w77) -> ("EOF?"=w75:bool, "mark after read (chars.)"=w73:i32)  [unwired: 3 in, 3 out]
        }
        n30 = Open/Create/Replace File(file path (use dialog)="Data Path", access (0:read/write)=enum16{"read/write", "read-only", "write-only"}."read-only") -> (error out=w70:errorcluster)  [unwired: 4 in, 2 out]
        "Log Error" <- w70
        n31 = Unbundle By Name(w70) -> ("status"=w69:bool)
        n32 = property on="Progress" class="Slide (strict)"("Scale.Maximum"=w67) -> ()  [unwired: 2 in, 2 out]
      }
      frame 3 {
        w84 = u64 500000
        # "Open XCAN Comm"
        # "Baudrate"
        n33 = local read "CAN0 Enable"() -> (w83:bool)
        n34 = local read "CAN1 Enable"() -> (w82:bool)
        n35 = case shown="True" w82 {
          tunnel: refnum<k21> "CAN3" ("XNET Interface") -> [_ w94]
          tunnel: w84 -> [_ w93]
          tunnel: [_ w88] -> w78
          tunnel: [_ w87] -> w80
          frame False {
          }
          frame True {
            n36 = call-poly <vilib>:"XNET Create Session.vi"("interface"=w94) -> ("session out"=w92:refnum<k21>, "error out"=w91:errorcluster)  [unwired: 13 in]
            n37 = property class="XNET Session"(reference=w92, error in=w91, "Intf.BaudRate64"=w93) -> (reference out=w90:refnum<k21>, error out=w89:errorcluster)
            n38 = call <vilib>:"XNET Start.vi"("session in"=w90, "error in (no error)"=w89) -> ("session out"=w87:refnum<k21>, "error out"=w88:errorcluster)  [unwired: 12 in]
          }
        }
        n39 = case shown="True" w83 {
          tunnel: w84 -> [_ w102]
          tunnel: refnum<k21> "CAN2" ("XNET Interface") -> [_ w101]
          tunnel: [_ w96] -> w79
          tunnel: [_ w95] -> w81
          frame False {
          }
          frame True {
            n40 = call-poly <vilib>:"XNET Create Session.vi"("interface"=w101) -> ("session out"=w99:refnum<k21>, "error out"=w100:errorcluster)  [unwired: 13 in]
            n41 = property class="XNET Session"(reference=w99, error in=w100, "Intf.BaudRate64"=w102) -> (reference out=w98:refnum<k21>, error out=w97:errorcluster)
            n42 = call <vilib>:"XNET Start.vi"("session in"=w98, "error in (no error)"=w97) -> ("session out"=w95:refnum<k21>, "error out"=w96:errorcluster)  [unwired: 12 in]
          }
        }
      }
    }
    n43 = Concatenate Strings(w25, w24, ".txt" ("string")) -> (w26:string)
    n44 = String To Path(string=w26) -> (path=w34:path)
    n45 = while {
      tunnel: w22 -> [w138]
      tunnel: w21 -> [w139]
      shift-right: [w136] -> _
      shift-left: u16[] [0, 0, 0, 0, 0, 0, 0, 0, 0, 0, 0, 0, 0, 0, 0, 0, 0, 0, 0, 0, 0, 0, 0, 0, 0, 0, 0, 0, 0, 0, 0, 0, 0, 0, 0, 0, 0, 0, 0, 0, 0, 0, 0, 0, 0, 0, 0, 0, 0, 0, 0, 0, 0, 0, 0, 0, 0, 0, 0, 0, 0, 0, 0, 0, 0, 0, 0, 0, 0, 0, 0, 0, 0, 0, 0, 0, 0, 0, 0, 0, 0, 0, 0, 0, 0, 0, 0, 0, 0, 0, 0, 0, 0, 0, 0, 0, 0, 0, 0, 0, 0, 0, 0, 0, 0, 0, 0, 0, 0, 0, 0, 0, 0, 0, 0, 0, 0, 0, 0, 0, 0, 0, 0, 0, 0, 0, 0, 0, 0, 0, 0, 0, 0, 0, 0, 0, 0, 0, 0, 0, 0, 0, 0, 0, 0, 0, 0, 0, 0, 0, 0, 0, 0, 0, 0, 0, 0, 0, 0, 0, 0, 0, 0, 0, 0, 0, 0, 0, 0, 0, 0, 0, 0, 0, 0, 0, 0, 0, 0, 0, 0] -> [w137]
      shift-right: [w135] -> _
      shift-left: dbl[] [0.0, 0.0, 0.0, 0.0, 0.0, 0.0, 0.0, 0.0, 0.0, 0.0, 0.0, 0.0, 0.0, 0.0, 0.0, 0.0, 0.0, 0.0, 0.0, 0.0, 0.0, 0.0, 0.0, 0.0, 0.0, 0.0, 0.0, 0.0, 0.0, 0.0, 0.0, 0.0, 0.0, 0.0, 0.0, 0.0, 0.0, 0.0, 0.0, 0.0, 0.0, 0.0, 0.0, 0.0, 0.0, 0.0, 0.0, 0.0, 0.0, 0.0, 0.0, 0.0, 0.0, 0.0, 0.0, 0.0, 0.0, 0.0, 0.0, 0.0, 0.0, 0.0, 0.0, 0.0, 0.0, 0.0, 0.0, 0.0, 0.0, 0.0, 0.0, 0.0, 0.0, 0.0, 0.0, 0.0, 0.0, 0.0, 0.0, 0.0, 0.0, 0.0, 0.0, 0.0, 0.0, 0.0, 0.0, 0.0, 0.0, 0.0, 0.0, 0.0, 0.0, 0.0, 0.0, 0.0, 0.0, 0.0, 0.0, 0.0, 0.0, 0.0, 0.0, 0.0, 0.0, 0.0, 0.0, 0.0, 0.0, 0.0, 0.0, 0.0, 0.0, 0.0, 0.0, 0.0, 0.0, 0.0, 0.0, 0.0, 0.0, 0.0, 0.0, 0.0, 0.0, 0.0, 0.0, 0.0, 0.0, 0.0, 0.0, 0.0, 0.0, 0.0, 0.0, 0.0, 0.0, 0.0, 0.0, 0.0, 0.0, 0.0, 0.0, 0.0, 0.0, 0.0, 0.0, 0.0, 0.0, 0.0, 0.0, 0.0, 0.0, 0.0, 0.0, 0.0, 0.0, 0.0, 0.0, 0.0, 0.0, 0.0, 0.0, 0.0, 0.0, 0.0, 0.0, 0.0, 0.0, 0.0, 0.0, 0.0, 0.0, 0.0, 0.0, 0.0, 0.0, 0.0, 0.0, 0.0, 0.0] -> [w134]
      shift-right: [w130] -> _
      shift-left: u16[] [0, 0, 0, 0, 0, 0, 0, 0, 0, 0, 0, 0, 0, 0] -> [w131]
      shift-right: [w129] -> _
      shift-left: bool[] [FALSE, FALSE, FALSE, FALSE, FALSE, FALSE, FALSE, FALSE, FALSE, FALSE, FALSE, FALSE, FALSE, FALSE] -> [w132]
      shift-right: [w128] -> _
      shift-left: dbl[] [0.0, 0.0, 0.0, 0.0, 0.0, 0.0, 0.0, 0.0, 0.0, 0.0, 0.0, 0.0, 0.0, 0.0] -> [w133]
      tunnel: w34 -> [w125]
      tunnel: w20 -> [w123]
      tunnel: w19 -> [w122]
      tunnel: w18 -> [w107]
      tunnel: w17 -> [w121]
      tunnel: w16 -> [w113]
      tunnel: w12 -> [w106]
      tunnel: w11 -> [w105]
      shift-right: [w104] -> w9
      shift-left: w5 -> [w104]
      tunnel: [w103] -> _
      tunnel: [w104] -> _
      shift-right: [w103] -> w10
      shift-left: w6 -> [w103]
      stop <- w109 stop-if-true
      n46 = local read "Data Source"() -> (w124:u16)
      n47 = case shown="False" "pause" {
        frame False {
        }
        frame True {
          n48 = stacked-sequence {
            frame #0 {
              n49 = while {
                stop <- w141 continue-if-true
                n50 = property on="pause" class="Bool (strict)"("BoolText.Text"="RESUME" ("Boolean Text.Text")) -> ()  [unwired: 2 in, 2 out]
                n51 = local read "pause"() -> (w141:bool)
              }
            }
            frame #1 {
              n52 = property on="pause" class="Bool (strict)"("BoolText.Text"="PAUSE" ("Boolean Text.Text")) -> ()  [unwired: 2 in, 2 out]
            }
          }
        }
      }
      n53 = Compound Arithmetic op=OR("stop", "Exit") -> (w109:bool)
      n54 = case shown="3" w124 {
        tunnel: w139 -> [w147 _ _ _]
        tunnel: w138 -> [w148 _ _ _]
        tunnel: [w146 w159 w202 w227] -> w120
        tunnel: w104 -> [_ w162 _ _]
        tunnel: w123 -> [_ w157 _ w231]
        tunnel: w122 -> [_ w150 _ w230]
        tunnel: w103 -> [_ w151 _ _]
        tunnel: w107 -> [_ w154 _ w233]
        tunnel: w121 -> [_ w153 _ w232]
        tunnel: w113 -> [_ _ w201 _]
        tunnel: w106 -> [_ _ _ w229]
        tunnel: w105 -> [_ _ _ w228]
        frame 0, Default {
          # "Read WiFi Data"
          n55 = call "ReadUDP.vi"("error in (no error)"=w147, "connection ID"=w148, "Message length"="Length") -> ("error out"=→"WiFi Error":errorcluster, "Array"=w146:u8[][])
        }
        frame 1 {
          w156 = u32 5 items=["(reserved)", "Protocol Version", "Software Version", "Object State", "(reserved)", "Read Entries Pending", "Write Entries Pending", "ReadMult Size for Notification", "Listen Only?", "Self Reception?", "Transmit Error Counter", "Receive Error Counter", "Single Shot Transmit?", "Series 2 Filter Mode", "Series 2 Mask", "Series 2 Comparator", "Serial Number", "Form Factor", "Series", "Transceiver Type", "Interface Number", "Series 2 Error/Arb Capture", "Transceiver Mode", "Transceiver External Outputs", "Transceiver External Inputs", "Start Trigger Behavior", "Log Comm Warnings", "User RTSI Frame", "Transmit Mode", "Log Start Trigger?", "Timestamp Format", "Master Timebase Rate", "Virtual Bus Timing", "Write Entries Free", "Timeline Recovery", "Log Bus Errors", "Log Transceiver Faults", "Termination", "LIN Sleep", "LIN Checksum Type", "LIN Response Timeout", "LIN Enable DLC Check", "LIN Log Wakeup", "Baud Rate"] ("AttrId")
          # "Read CAN-USB Data"
          n56 = Merge Errors(w150, w150) -> (w152:errorcluster)
          n57 = case shown="True" w154 {
            tunnel: w156 -> [_ w167]
            tunnel: w152 -> [w165 w180]
            tunnel: w151 -> [w163 w168]
            tunnel: [u8[] [] ("Data") w170] -> w161
            tunnel: [w165 w169] -> w155
            tunnel: [w163 w166] -> _
            frame False {
            }
            frame True {
              n58 = call <vilib>:"ncGetAttr.vi"("Error in"=w180, "AttrId"=w167, "ObjHandle in"=w168) -> ("Error out"=w179:errorcluster, "ObjHandle out"=w181:T13)  [unwired: 1 out]
              n59 = call <vilib>:"ncReadNet.vi"("ObjHandle in"=w181, "Error in"=w179) -> ("ArbitrationId"=w172:u32, "ObjHandle out"=w166:T13, "Data"=w178:u8[], "Error out"=w169:errorcluster)  [unwired: 2 in, 3 out]
              n60 = To Unsigned Word Integer(number=w172) -> (unsigned 16bit integer=w171:u16)
              n61 = Split Number(x=w171) -> (hi(x)=w174:u8, lo(x)=w173:u8)
              n62 = Insert Into Array(array=w178, index=0, new element=w174) -> (w176:u8[])
              n63 = Insert Into Array(array=w176, index=1, new element=w173) -> (w170:u8[])
            }
          }
          "CAN0 Error" <- w155
          n64 = case shown="True" w153 {
            tunnel: w162 -> [w182 w199]
            tunnel: w156 -> [_ w198]
            tunnel: [u8[] [] ("Data") w188] -> w160
            tunnel: [w184 w187] -> w158
            tunnel: w157 -> [w184 w186]
            tunnel: [w182 w185] -> _
            frame False {
            }
            frame True {
              n65 = call <vilib>:"ncGetAttr.vi"("Error in"=w186, "AttrId"=w198, "ObjHandle in"=w199) -> ("Error out"=w197:errorcluster, "ObjHandle out"=w200:T13)  [unwired: 1 out]
              n66 = call <vilib>:"ncReadNet.vi"("ObjHandle in"=w200, "Error in"=w197) -> ("ArbitrationId"=w196:u32, "ObjHandle out"=w185:T13, "Data"=w192:u8[], "Error out"=w187:errorcluster)  [unwired: 2 in, 3 out]
              n67 = To Unsigned Word Integer(number=w196) -> (unsigned 16bit integer=w195:u16)
              n68 = Split Number(x=w195) -> (hi(x)=w191:u8, lo(x)=w189:u8)
              n69 = Insert Into Array(array=w192, index=0, new element=w191) -> (w190:u8[])
              n70 = Insert Into Array(array=w190, index=1, new element=w189) -> (w188:u8[])
            }
          }
          "CAN1 Error" <- w158
          n71 = Build Array(w161, w160) -> (w159:u8[][])
        }
        frame 2 {
          n72 = case shown="False" w201 {
            tunnel: [w216 u8[][] []] -> w202
            frame False {
              n73 = Wait Until Next ms Multiple(millisecond multiple="Timestep") -> ()  [unwired: 1 out]
              n74 = local read "Data Path"() -> (w222:path)
              n75 = call-poly <vilib>:"Read From Spreadsheet File.vi"("delimiter (\\t)"=";" ("delimiter (\\t)"), "start of read offset (chars.:0)"="Progress", "number of rows (all:-1)"="Rows to read", "file path (dialog if empty)"=w222) -> ("mark after read (chars.)"=w213:i32, "all rows"=w220:string[][])  [unwired: 3 in, 3 out]
              n76 = Delete From Array(array=w220, index (col)=0 ("disabled index (col)")) -> (deleted portion=w207:string[], array with subset deleted=w218:string[][])  [unwired: 2 in]
              n77 = case shown="True" "Play" {
                tunnel: w213 -> [_ w223]
                frame False {
                }
                frame True {
                  n78 = local write "Progress"(w223) -> ()
                }
              }
              n79 = Array Size(array=w207) -> (size(s)=w209:i32)
              n80 = Decimal String To Number(string=w218, default (0L)=u8 0 ("default (0 I32)")) -> (number=w216:u8[][])  [unwired: 1 in, 1 out]
              n81 = Decrement(x=w209) -> (x-1=w208:i32)
              n82 = Index Array(array=w207, index=w208) -> (element=w204:string)
              n83 = Index Array(array=w207, index=1) -> (element=w206:string)
              n84 = Concatenate Strings(w206, "\r\n", w204) -> (→"Time Stamp":string)
            }
            frame True {
            }
          }
        }
        frame 3 {
          n85 = case shown="True" w233 {
            tunnel: w229 -> [_ w269]
            tunnel: w230 -> [w254 w268]
            tunnel: [u8[] [] ("Data") w256] -> w235
            tunnel: [w254 w255] -> w226
            frame False {
            }
            frame True {
              n86 = call-poly <vilib>:"XNET Read.vi"("session in"=w269, "number to read (-1)"=1, "error in (no error)"=w268) -> ("data"=w266:T14[], "error out"=w255:errorcluster)  [unwired: 9 in, 2 out]
              n87 = Index Array(array=w266) -> (element=w265:T14)  [unwired: 1 in]
              n88 = Unbundle By Name(w265) -> ("identifier"=w264:u32, "payload"=w262:u8[])
              n89 = To Unsigned Word Integer(number=w264) -> (unsigned 16bit integer=w263:u16)
              n90 = Split Number(x=w263) -> (hi(x)=w260:u8, lo(x)=w258:u8)
              n91 = Insert Into Array(array=w262, index=0, new element=w260) -> (w259:u8[])
              n92 = Insert Into Array(array=w259, index=1, new element=w258) -> (w256:u8[])
            }
          }
          n93 = case shown="True" w232 {
            tunnel: w231 -> [w237 w251]
            tunnel: w228 -> [_ w252]
            tunnel: [w237 w249] -> w225
            tunnel: [u8[] [] ("Data") w238] -> w234
            frame False {
            }
            frame True {
              n94 = call-poly <vilib>:"XNET Read.vi"("session in"=w252, "number to read (-1)"=1, "error in (no error)"=w251) -> ("data"=w248:T14[], "error out"=w249:errorcluster)  [unwired: 9 in, 2 out]
              n95 = Index Array(array=w248) -> (element=w247:T14)  [unwired: 1 in]
              n96 = Unbundle By Name(w247) -> ("payload"=w246:u8[], "identifier"=w244:u32)
              n97 = To Unsigned Word Integer(number=w244) -> (unsigned 16bit integer=w243:u16)
              n98 = Split Number(x=w243) -> (hi(x)=w242:u8, lo(x)=w241:u8)
              n99 = Insert Into Array(array=w246, index=0, new element=w242) -> (w245:u8[])
              n100 = Insert Into Array(array=w245, index=1, new element=w241) -> (w238:u8[])
            }
          }
          n101 = local write "CAN0 Error"(w226) -> ()
          n102 = Build Array(w235, w234) -> (w227:u8[][])
          n103 = local write "CAN1 Error"(w225) -> ()
        }
      }
      n104 = case shown="True" "Log Enable" {
        tunnel: w125 -> [_ w273]
        tunnel: w120 -> [_ w272]
        frame False {
        }
        frame True {
          n105 = for {
            tunnel: w272 -> [w280] mode=indexing
            tunnel: [w278] -> w271 mode=indexing
            n106 = Get Date/Time In Seconds() -> (seconds since 1Jan1904=w276:timestamp)
            n107 = Format Date/Time String(time format string (%c)="%Y.%m.%d. %H:%M:%S%3u", seconds (now)=w276) -> (date/time string=w279:string)  [unwired: 1 in]
            n108 = Number To Decimal String(number=w280) -> (decimal integer string=w277:string[])  [unwired: 1 in]
            n109 = Build Array (concatenate)(w279, w277) -> (w278:string[])
          }
          n110 = call-poly <vilib>:"Write To Spreadsheet File.vi"("delimiter (\\t)"=";" ("delimiter (\\t)"), "append to file? (new file:F)"=TRUE, "2D data"=w271, "file path (dialog if empty)"=w273) -> ()  [unwired: 4 in, 1 out]
        }
      }
      n111 = for {
        tunnel: w120 -> [w293] mode=indexing
        tunnel: [w294] -> w127 mode=indexing
        shift-right: [w284] -> w136
        shift-left: w137 -> [w292]
        shift-right: [w290] -> w135
        shift-left: w134 -> [w291]
        shift-right: [w288] -> w130
        shift-left: w131 -> [w289]
        shift-right: [w283] -> w129
        shift-left: w132 -> [w287]
        shift-right: [w285] -> w128
        shift-left: w133 -> [w286]
        # "CAN ID"
        n112 = Index Array(array=w293, index=0) -> (element=w296:u8)
        n113 = Index Array(array=w293, index=1) -> (element=w295:u8)
        n114 = Join Numbers(hi=w296, lo=w295) -> ((hi.lo)=w294:u16)
        n115 = case shown="480" w294 {
          tunnel: w293 -> [_ w309 w410 w510 w637 w691 w739 w760 w787 w818 w849 w894 w923 w1044 w1066 w1074 w1182 w1251 w1281 w1351 w1431 w1484 w1569 w1599 w1645 w1679 w1722 w1751 w1785 w1866 w1932 w1967 w2038 w2047 w2058 w2119 w2136 w2155 w2223 w2329 w2364 w2442 w2506 w2569 w2593 w2611 w2635 w2690 w2746 w2760 w2803 w2810 w2814 w2840 w2857 w2876 w2927 w2942 w2953 w2967 w2991 w3018 w3039]
          tunnel: w292 -> [w303 w304 w405 w505 w644 w698 w746 w775 w806 w837 w868 w901 w930 w1051 w1068 w1098 w1213 w1268 w1295 w1355 w1446 w1528 w1588 w1634 w1674 w1710 w1745 w1780 w1816 w1897 w1961 w1996 w2037 w2049 w2054 w2115 w2145 w2201 w2310 w2353 w2418 w2447 w2552 w2586 w2594 w2612 w2636 w2703 w2755 w2779 w2798 w2806 w2837 w2849 w2858 w2877 w2928 w2943 w2954 w2973 w3008 w3013 w3032]
          tunnel: [w303 w304 w405 w505 w644 w698 w746 w775 w806 w837 w868 w901 w930 w1051 w1068 w1098 w1213 w1268 w1295 w1325 w1446 w1528 w1588 w1634 w1674 w1710 w1745 w1780 w1816 w1897 w1961 w1996 w2037 w2049 w2054 w2115 w2145 w2201 w2310 w2353 w2418 w2447 w2552 w2586 w2594 w2612 w2636 w2703 w2755 w2779 w2798 w2806 w2837 w2849 w2858 w2877 w2928 w2943 w2954 w2973 w3008 w3013 w3032] -> w284
          tunnel: w291 -> [w302 w308 w404 w504 w643 w697 w745 w774 w805 w836 w867 w900 w929 w1050 w1067 w1097 w1212 w1267 w1294 w1348 w1445 w1527 w1592 w1638 w1673 w1709 w1744 w1779 w1815 w1896 w1960 w1995 w2036 w2048 w2053 w2114 w2149 w2200 w2314 w2357 w2421 w2446 w2551 w2590 w2606 w2616 w2640 w2707 w2759 w2772 w2797 w2805 w2836 w2853 w2862 w2881 w2932 w2947 w2958 w2972 w3007 w3017 w3031]
          tunnel: [w302 w308 w404 w504 w643 w697 w745 w774 w805 w836 w867 w900 w929 w1050 w1067 w1097 w1212 w1267 w1294 w1301 w1445 w1527 w1592 w1638 w1673 w1709 w1744 w1779 w1815 w1896 w1960 w1995 w2036 w2048 w2053 w2114 w2149 w2200 w2314 w2357 w2421 w2446 w2551 w2590 w2606 w2616 w2640 w2707 w2759 w2772 w2797 w2805 w2836 w2853 w2862 w2881 w2932 w2947 w2958 w2972 w3007 w3017 w3031] -> w290
          tunnel: w289 -> [w301 w307 w408 w508 w642 w696 w744 w773 w804 w835 w864 w899 w928 w1049 w1071 w1094 w1211 w1266 w1293 w1335 w1442 w1522 w1591 w1637 w1670 w1706 w1741 w1776 w1812 w1893 w1957 w1992 w2006 w2052 w2057 w2118 w2148 w2193 w2313 w2356 w2420 w2445 w2550 w2589 w2605 w2615 w2639 w2706 w2758 w2780 w2801 w2809 w2834 w2852 w2861 w2880 w2931 w2946 w2957 w2970 w3004 w3016 w3035]
          tunnel: [w301 w307 w408 w508 w642 w696 w744 w773 w804 w835 w864 w899 w928 w1049 w1071 w1094 w1211 w1266 w1293 w1335 w1442 w1522 w1591 w1637 w1670 w1706 w1741 w1776 w1812 w1893 w1957 w1992 w2006 w2052 w2057 w2118 w2148 w2193 w2313 w2356 w2420 w2445 w2550 w2589 w2605 w2615 w2639 w2706 w2758 w2762 w2801 w2809 w2834 w2852 w2861 w2880 w2931 w2946 w2957 w2970 w3004 w3016 w3035] -> w288
          tunnel: w287 -> [w300 w306 w407 w507 w641 w695 w743 w772 w803 w834 w863 w898 w927 w1048 w1070 w1095 w1210 w1265 w1292 w1333 w1443 w1521 w1590 w1636 w1671 w1707 w1742 w1777 w1813 w1894 w1958 w1993 w2005 w2051 w2056 w2117 w2147 w2192 w2312 w2355 w2419 w2444 w2549 w2588 w2604 w2614 w2638 w2705 w2757 w2776 w2800 w2808 w2833 w2851 w2860 w2879 w2930 w2945 w2956 w2969 w3005 w3015 w3034]
          tunnel: w286 -> [w299 w305 w406 w506 w640 w694 w742 w771 w802 w833 w862 w897 w926 w1047 w1069 w1096 w1209 w1264 w1291 w1334 w1444 w1526 w1589 w1635 w1672 w1708 w1743 w1778 w1814 w1895 w1959 w1994 w2035 w2050 w2055 w2116 w2146 w2199 w2311 w2354 w2417 w2443 w2548 w2587 w2603 w2613 w2637 w2704 w2756 w2773 w2799 w2807 w2835 w2850 w2859 w2878 w2929 w2944 w2955 w2971 w3006 w3014 w3033]
          tunnel: [w299 w305 w406 w506 w640 w694 w742 w771 w802 w833 w862 w897 w926 w1047 w1069 w1096 w1209 w1264 w1291 w1334 w1444 w1526 w1589 w1635 w1672 w1708 w1743 w1778 w1814 w1895 w1959 w1994 w2035 w2050 w2055 w2116 w2146 w2199 w2311 w2354 w2417 w2443 w2548 w2587 w2603 w2613 w2637 w2704 w2756 w2768 w2799 w2807 w2835 w2850 w2859 w2878 w2929 w2944 w2955 w2971 w3006 w3014 w3033] -> w285
          tunnel: [w300 w306 w407 w507 w641 w695 w743 w772 w803 w834 w863 w898 w927 w1048 w1070 w1095 w1210 w1265 w1292 w1333 w1443 w1521 w1590 w1636 w1671 w1707 w1742 w1777 w1813 w1894 w1958 w1993 w2005 w2051 w2056 w2117 w2147 w2192 w2312 w2355 w2419 w2444 w2549 w2588 w2604 w2614 w2638 w2705 w2757 w2774 w2800 w2808 w2833 w2851 w2860 w2879 w2930 w2945 w2956 w2969 w3005 w3015 w3034] -> w283
          frame 0, Default {
          }
          frame 272 {
            w397 = u64 511 ("y")
            w375 = -1.0 ("y")
            w362 = i16 -8 ("y")
            w361 = u64 511 ("y")
            w360 = u64 1023 ("y")
            w359 = u64 3 ("y")
            n116 = local read "ConeType"() -> (w336:cluster{"Col":dbl, "X":dbl, "Y":dbl})
            n117 = Array Subset(array=w309, index=2, length=8) -> (w339:u8[])
            n118 = Index Array(array=w339, index #1=7 ("index"), index #2=6 ("index"), index #3=5 ("index"), index #4=4 ("index"), index #5=3 ("index"), index #6=2 ("index"), index #7=1 ("index"), index #8=0 ("index")) -> (element #1=w318:u8, element #2=w319:u8, element #3=w320:u8, element #4=w321:u8, element #5=w322:u8, element #6=w323:u8, element #7=w324:u8, element #8=w325:u8)
            n119 = Join Numbers(hi=w318, lo=w319) -> ((hi.lo)=w326:u16)
            n120 = Join Numbers(hi=w320, lo=w321) -> ((hi.lo)=w327:u16)
            n121 = Join Numbers(hi=w322, lo=w323) -> ((hi.lo)=w328:u16)
            n122 = Join Numbers(hi=w324, lo=w325) -> ((hi.lo)=w329:u16)
            n123 = Join Numbers(hi=w326, lo=w327) -> ((hi.lo)=w330:u32)
            n124 = Join Numbers(hi=w328, lo=w329) -> ((hi.lo)=w331:u32)
            n125 = Join Numbers(hi=w330, lo=w331) -> ((hi.lo)=w340:u64)
            "(hi.lo)" <- w340
            n126 = Logical Shift(y=i16 0, x=w340) -> (x << y=w350:u64)
            n127 = Logical Shift(y=i16 -2, x=w340) -> (x << y=w351:u64)
            n128 = Logical Shift(y=i16 -12, x=w340) -> (x << y=w352:u64)
            n129 = Logical Shift(y=i16 -21, x=w340) -> (x << y=w353:u64)
            n130 = Logical Shift(y=i16 -23, x=w340) -> (x << y=w354:u64)
            n131 = Logical Shift(y=i16 -33, x=w340) -> (x << y=w355:u64)
            n132 = Logical Shift(y=i16 -42, x=w340) -> (x << y=w356:u64)
            n133 = Logical Shift(y=i16 -44, x=w340) -> (x << y=w357:u64)
            n134 = Logical Shift(y=i16 -54, x=w340) -> (x << y=w358:u64)
            n135 = And(x=w350, y=w359) -> (x .and. y?=w378:u64)
            n136 = And(x=w351, y=w360) -> (x .and. y?=w380:u64)
            n137 = And(x=w353, y=w359) -> (x .and. y?=w377:u64)
            n138 = And(x=w354, y=w360) -> (x .and. y?=w381:u64)
            n139 = And(x=w356, y=w359) -> (x .and. y?=w376:u64)
            n140 = And(x=w357, y=w360) -> (x .and. y?=w379:u64)
            n141 = And(x=w352, y=w361) -> (x .and. y?=w389:u64)
            n142 = And(x=w355, y=w361) -> (x .and. y?=w385:u64)
            n143 = And(x=w358, y=w361) -> (x .and. y?=w387:u64)
            n144 = Logical Shift(y=w362, x=w389) -> (x << y=w363:u64)
            n145 = Logical Shift(y=w362, x=w385) -> (x << y=w364:u64)
            n146 = Logical Shift(y=w362, x=w387) -> (x << y=w365:u64)
            n147 = To Unsigned Byte Integer(number=w378) -> (unsigned 8bit integer=w403:u8)
            n148 = To Unsigned Word Integer(number=w380) -> (unsigned 16bit integer=w402:u16)
            n149 = Decrement(x=w389) -> (x-1=w369:u64)
            n150 = To Unsigned Byte Integer(number=w377) -> (unsigned 8bit integer=w401:u8)
            n151 = To Unsigned Word Integer(number=w381) -> (unsigned 16bit integer=w400:u16)
            n152 = Decrement(x=w385) -> (x-1=w370:u64)
            n153 = To Unsigned Byte Integer(number=w376) -> (unsigned 8bit integer=w398:u8)
            n154 = To Unsigned Word Integer(number=w379) -> (unsigned 16bit integer=w399:u16)
            n155 = Decrement(x=w387) -> (x-1=w371:u64)
            n156 = Not(x=w369) -> (.not. x?=w392:u64)
            n157 = Not Equal To 0?(x=w363) -> (x != 0?=w367:bool)
            n158 = Not(x=w370) -> (.not. x?=w393:u64)
            n159 = Not Equal To 0?(x=w364) -> (x != 0?=w368:bool)
            n160 = Not(x=w371) -> (.not. x?=w395:u64)
            n161 = Not Equal To 0?(x=w365) -> (x != 0?=w366:bool)
            n162 = And(x=w397, y=w392) -> (x .and. y?=w391:u64)
            n163 = And(x=w397, y=w393) -> (x .and. y?=w394:u64)
            n164 = And(x=w397, y=w395) -> (x .and. y?=w396:u64)
            n165 = To Double Precision Float(number=w385) -> (double precision float=w386:dbl)
            n166 = Multiply(x=w375, y=w391) -> (x*y=w372:dbl)
            n167 = Multiply(x=w375, y=w394) -> (x*y=w374:dbl)
            n168 = Multiply(x=w375, y=w396) -> (x*y=w373:dbl)
            n169 = To Double Precision Float(number=w389) -> (double precision float=w390:dbl)
            n170 = To Double Precision Float(number=w387) -> (double precision float=w388:dbl)
            n171 = Select(t=w372, s=w367, f=w390) -> (s? t:f=w382:dbl)
            n172 = Select(t=w374, s=w368, f=w386) -> (s? t:f=w384:dbl)
            n173 = Select(t=w373, s=w366, f=w388) -> (s? t:f=w383:dbl)
            n174 = Bundle By Name(cluster=w336, "Col"=w403, "X"=w402, "Y"=w382) -> (w332:cluster{"Col":dbl, "X":dbl, "Y":dbl})
            n175 = Bundle By Name(cluster=w336, "Col"=w401, "X"=w400, "Y"=w384) -> (w333:cluster{"Col":dbl, "X":dbl, "Y":dbl})
            n176 = Bundle By Name(cluster=w336, "Col"=w398, "X"=w399, "Y"=w383) -> (w334:cluster{"Col":dbl, "X":dbl, "Y":dbl})
            n177 = Build Cluster Array(w332, w333, w334) -> (→"Cones1":T16)
          }
          frame 273 {
            w497 = u64 511 ("y")
            w475 = -1.0 ("y")
            w462 = i16 -8 ("y")
            w461 = u64 511 ("y")
            w460 = u64 1023 ("y")
            w459 = u64 3 ("y")
            n178 = local read "ConeType"() -> (w409:cluster{"Col":dbl, "X":dbl, "Y":dbl})
            n179 = Array Subset(array=w410, index=2, length=8) -> (w439:u8[])
            n180 = Index Array(array=w439, index #1=7 ("index"), index #2=6 ("index"), index #3=5 ("index"), index #4=4 ("index"), index #5=3 ("index"), index #6=2 ("index"), index #7=1 ("index"), index #8=0 ("index")) -> (element #1=w419:u8, element #2=w420:u8, element #3=w421:u8, element #4=w422:u8, element #5=w423:u8, element #6=w424:u8, element #7=w425:u8, element #8=w426:u8)
            n181 = Join Numbers(hi=w419, lo=w420) -> ((hi.lo)=w427:u16)
            n182 = Join Numbers(hi=w421, lo=w422) -> ((hi.lo)=w428:u16)
            n183 = Join Numbers(hi=w423, lo=w424) -> ((hi.lo)=w429:u16)
            n184 = Join Numbers(hi=w425, lo=w426) -> ((hi.lo)=w430:u16)
            n185 = Join Numbers(hi=w427, lo=w428) -> ((hi.lo)=w431:u32)
            n186 = Join Numbers(hi=w429, lo=w430) -> ((hi.lo)=w432:u32)
            n187 = Join Numbers(hi=w431, lo=w432) -> ((hi.lo)=w440:u64)
            "(hi.lo) 2" <- w440
            n188 = Logical Shift(y=i16 0, x=w440) -> (x << y=w450:u64)
            n189 = Logical Shift(y=i16 -2, x=w440) -> (x << y=w451:u64)
            n190 = Logical Shift(y=i16 -12, x=w440) -> (x << y=w452:u64)
            n191 = Logical Shift(y=i16 -21, x=w440) -> (x << y=w453:u64)
            n192 = Logical Shift(y=i16 -23, x=w440) -> (x << y=w454:u64)
            n193 = Logical Shift(y=i16 -33, x=w440) -> (x << y=w455:u64)
            n194 = Logical Shift(y=i16 -42, x=w440) -> (x << y=w456:u64)
            n195 = Logical Shift(y=i16 -44, x=w440) -> (x << y=w457:u64)
            n196 = Logical Shift(y=i16 -54, x=w440) -> (x << y=w458:u64)
            n197 = And(x=w450, y=w459) -> (x .and. y?=w478:u64)
            n198 = And(x=w451, y=w460) -> (x .and. y?=w480:u64)
            n199 = And(x=w453, y=w459) -> (x .and. y?=w477:u64)
            n200 = And(x=w454, y=w460) -> (x .and. y?=w481:u64)
            n201 = And(x=w456, y=w459) -> (x .and. y?=w476:u64)
            n202 = And(x=w457, y=w460) -> (x .and. y?=w479:u64)
            n203 = And(x=w452, y=w461) -> (x .and. y?=w489:u64)
            n204 = And(x=w455, y=w461) -> (x .and. y?=w485:u64)
            n205 = And(x=w458, y=w461) -> (x .and. y?=w487:u64)
            n206 = Logical Shift(y=w462, x=w489) -> (x << y=w463:u64)
            n207 = Logical Shift(y=w462, x=w485) -> (x << y=w464:u64)
            n208 = Logical Shift(y=w462, x=w487) -> (x << y=w465:u64)
            n209 = To Unsigned Byte Integer(number=w478) -> (unsigned 8bit integer=w503:u8)
            n210 = To Unsigned Word Integer(number=w480) -> (unsigned 16bit integer=w502:u16)
            n211 = Decrement(x=w489) -> (x-1=w469:u64)
            n212 = To Unsigned Byte Integer(number=w477) -> (unsigned 8bit integer=w501:u8)
            n213 = To Unsigned Word Integer(number=w481) -> (unsigned 16bit integer=w500:u16)
            n214 = Decrement(x=w485) -> (x-1=w470:u64)
            n215 = To Unsigned Byte Integer(number=w476) -> (unsigned 8bit integer=w498:u8)
            n216 = To Unsigned Word Integer(number=w479) -> (unsigned 16bit integer=w499:u16)
            n217 = Decrement(x=w487) -> (x-1=w471:u64)
            n218 = Not(x=w469) -> (.not. x?=w492:u64)
            n219 = Not Equal To 0?(x=w463) -> (x != 0?=w467:bool)
            n220 = Not(x=w470) -> (.not. x?=w493:u64)
            n221 = Not Equal To 0?(x=w464) -> (x != 0?=w468:bool)
            n222 = Not(x=w471) -> (.not. x?=w495:u64)
            n223 = Not Equal To 0?(x=w465) -> (x != 0?=w466:bool)
            n224 = And(x=w497, y=w492) -> (x .and. y?=w491:u64)
            n225 = And(x=w497, y=w493) -> (x .and. y?=w494:u64)
            n226 = And(x=w497, y=w495) -> (x .and. y?=w496:u64)
            n227 = To Double Precision Float(number=w485) -> (double precision float=w486:dbl)
            n228 = Multiply(x=w475, y=w491) -> (x*y=w472:dbl)
            n229 = Multiply(x=w475, y=w494) -> (x*y=w474:dbl)
            n230 = Multiply(x=w475, y=w496) -> (x*y=w473:dbl)
            n231 = To Double Precision Float(number=w489) -> (double precision float=w490:dbl)
            n232 = To Double Precision Float(number=w487) -> (double precision float=w488:dbl)
            n233 = Select(t=w472, s=w467, f=w490) -> (s? t:f=w482:dbl)
            n234 = Select(t=w474, s=w468, f=w486) -> (s? t:f=w484:dbl)
            n235 = Select(t=w473, s=w466, f=w488) -> (s? t:f=w483:dbl)
            n236 = Bundle By Name(cluster=w409, "Col"=w503, "X"=w502, "Y"=w482) -> (w433:cluster{"Col":dbl, "X":dbl, "Y":dbl})
            n237 = Bundle By Name(cluster=w409, "Col"=w501, "X"=w500, "Y"=w484) -> (w434:cluster{"Col":dbl, "X":dbl, "Y":dbl})
            n238 = Bundle By Name(cluster=w409, "Col"=w498, "X"=w499, "Y"=w483) -> (w435:cluster{"Col":dbl, "X":dbl, "Y":dbl})
            n239 = Build Cluster Array(w433, w434, w435) -> (→"Cones2":T16)
          }
          frame 274 {
            w597 = u64 511 ("y")
            w575 = -1.0 ("y")
            w562 = i16 -8 ("y")
            w561 = u64 511 ("y")
            w560 = u64 1023 ("y")
            w559 = u64 3 ("y")
            n240 = local read "ConeType"() -> (w509:cluster{"Col":dbl, "X":dbl, "Y":dbl})
            n241 = Array Subset(array=w510, index=2, length=8) -> (w539:u8[])
            n242 = Index Array(array=w539, index #1=7 ("index"), index #2=6 ("index"), index #3=5 ("index"), index #4=4 ("index"), index #5=3 ("index"), index #6=2 ("index"), index #7=1 ("index"), index #8=0 ("index")) -> (element #1=w519:u8, element #2=w520:u8, element #3=w521:u8, element #4=w522:u8, element #5=w523:u8, element #6=w524:u8, element #7=w525:u8, element #8=w526:u8)
            n243 = Join Numbers(hi=w519, lo=w520) -> ((hi.lo)=w527:u16)
            n244 = Join Numbers(hi=w521, lo=w522) -> ((hi.lo)=w528:u16)
            n245 = Join Numbers(hi=w523, lo=w524) -> ((hi.lo)=w529:u16)
            n246 = Join Numbers(hi=w525, lo=w526) -> ((hi.lo)=w530:u16)
            n247 = Join Numbers(hi=w527, lo=w528) -> ((hi.lo)=w531:u32)
            n248 = Join Numbers(hi=w529, lo=w530) -> ((hi.lo)=w532:u32)
            n249 = Join Numbers(hi=w531, lo=w532) -> ((hi.lo)=w540:u64)
            "(hi.lo) 3" <- w540
            n250 = Logical Shift(y=i16 0, x=w540) -> (x << y=w550:u64)
            n251 = Logical Shift(y=i16 -2, x=w540) -> (x << y=w551:u64)
            n252 = Logical Shift(y=i16 -12, x=w540) -> (x << y=w552:u64)
            n253 = Logical Shift(y=i16 -21, x=w540) -> (x << y=w553:u64)
            n254 = Logical Shift(y=i16 -23, x=w540) -> (x << y=w554:u64)
            n255 = Logical Shift(y=i16 -33, x=w540) -> (x << y=w555:u64)
            n256 = Logical Shift(y=i16 -42, x=w540) -> (x << y=w556:u64)
            n257 = Logical Shift(y=i16 -44, x=w540) -> (x << y=w557:u64)
            n258 = Logical Shift(y=i16 -54, x=w540) -> (x << y=w558:u64)
            n259 = And(x=w550, y=w559) -> (x .and. y?=w578:u64)
            n260 = And(x=w551, y=w560) -> (x .and. y?=w580:u64)
            n261 = And(x=w553, y=w559) -> (x .and. y?=w577:u64)
            n262 = And(x=w554, y=w560) -> (x .and. y?=w581:u64)
            n263 = And(x=w556, y=w559) -> (x .and. y?=w576:u64)
            n264 = And(x=w557, y=w560) -> (x .and. y?=w579:u64)
            n265 = And(x=w552, y=w561) -> (x .and. y?=w589:u64)
            n266 = And(x=w555, y=w561) -> (x .and. y?=w585:u64)
            n267 = And(x=w558, y=w561) -> (x .and. y?=w587:u64)
            n268 = Logical Shift(y=w562, x=w589) -> (x << y=w563:u64)
            n269 = Logical Shift(y=w562, x=w585) -> (x << y=w564:u64)
            n270 = Logical Shift(y=w562, x=w587) -> (x << y=w565:u64)
            n271 = To Unsigned Byte Integer(number=w578) -> (unsigned 8bit integer=w603:u8)
            n272 = To Unsigned Word Integer(number=w580) -> (unsigned 16bit integer=w602:u16)
            n273 = Decrement(x=w589) -> (x-1=w569:u64)
            n274 = To Unsigned Byte Integer(number=w577) -> (unsigned 8bit integer=w601:u8)
            n275 = To Unsigned Word Integer(number=w581) -> (unsigned 16bit integer=w600:u16)
            n276 = Decrement(x=w585) -> (x-1=w570:u64)
            n277 = To Unsigned Byte Integer(number=w576) -> (unsigned 8bit integer=w598:u8)
            n278 = To Unsigned Word Integer(number=w579) -> (unsigned 16bit integer=w599:u16)
            n279 = Decrement(x=w587) -> (x-1=w571:u64)
            n280 = Not(x=w569) -> (.not. x?=w592:u64)
            n281 = Not Equal To 0?(x=w563) -> (x != 0?=w567:bool)
            n282 = Not(x=w570) -> (.not. x?=w593:u64)
            n283 = Not Equal To 0?(x=w564) -> (x != 0?=w568:bool)
            n284 = Not(x=w571) -> (.not. x?=w595:u64)
            n285 = Not Equal To 0?(x=w565) -> (x != 0?=w566:bool)
            n286 = And(x=w597, y=w592) -> (x .and. y?=w591:u64)
            n287 = And(x=w597, y=w593) -> (x .and. y?=w594:u64)
            n288 = And(x=w597, y=w595) -> (x .and. y?=w596:u64)
            n289 = To Double Precision Float(number=w585) -> (double precision float=w586:dbl)
            n290 = Multiply(x=w575, y=w591) -> (x*y=w572:dbl)
            n291 = Multiply(x=w575, y=w594) -> (x*y=w574:dbl)
            n292 = Multiply(x=w575, y=w596) -> (x*y=w573:dbl)
            n293 = To Double Precision Float(number=w589) -> (double precision float=w590:dbl)
            n294 = To Double Precision Float(number=w587) -> (double precision float=w588:dbl)
            n295 = Select(t=w572, s=w567, f=w590) -> (s? t:f=w582:dbl)
            n296 = Select(t=w574, s=w568, f=w586) -> (s? t:f=w584:dbl)
            n297 = Select(t=w573, s=w566, f=w588) -> (s? t:f=w583:dbl)
            n298 = Bundle By Name(cluster=w509, "Col"=w603, "X"=w602, "Y"=w582) -> (w533:cluster{"Col":dbl, "X":dbl, "Y":dbl})
            n299 = Bundle By Name(cluster=w509, "Col"=w601, "X"=w600, "Y"=w584) -> (w534:cluster{"Col":dbl, "X":dbl, "Y":dbl})
            n300 = Bundle By Name(cluster=w509, "Col"=w598, "X"=w599, "Y"=w583) -> (w535:cluster{"Col":dbl, "X":dbl, "Y":dbl})
            n301 = Build Cluster Array(w533, w534, w535) -> (→"Cones3":T16)
          }
          frame 372 {
            w632 = i16 -32768
            # "Acceleration Y & Yaw"
            n302 = local read "IsStopped"() -> (w620:bool)
            n303 = Index Array(array=w637, index=7) -> (element=w636:u8)
            n304 = Index Array(array=w637, index=6) -> (element=w633:u8)
            n305 = Index Array(array=w637, index=3) -> (element=w635:u8)
            n306 = Index Array(array=w637, index=2) -> (element=w634:u8)
            n307 = case shown="True" w620 {
              frame False {
              }
              frame True {
                n308 = feedback #1() -> (w649:dbl)  [unwired: 1 in]
                n309 = local read "OffsetFilter"() -> (w647:dbl)
                n310 = local read "Acc Y"() -> (w650:dbl)
                n311 = formula code="y_=a*x+(1-a)*y;"("x"=w650, "y"=w649, "a"=w647) -> ("y_"=w648:dbl)
                n312 = feedback-in #1(w648) -> ()
                n313 = local write "Acc Y offset"(w648) -> ()
              }
            }
            n314 = Join Numbers(hi=w636, lo=w633) -> ((hi.lo)=w630:u16)
            n315 = Join Numbers(hi=w635, lo=w634) -> ((hi.lo)=w628:u16)
            n316 = local read "Actual Velocity \nRR [RPM]"() -> (w613:i16)
            n317 = local read "Actual Velocity\nFR [RPM]"() -> (w612:i16)
            n318 = local read "Actual Velocity\nRL [RPM]"() -> (w614:i16)
            n319 = local read "Actual Velocity\nFL [RPM]"() -> (w609:i16)
            n320 = To Word Integer(number=w630) -> (16bit integer=w631:i16)
            n321 = To Word Integer(number=w628) -> (16bit integer=w629:i16)
            n322 = Subtract(x=w631, y=w632) -> (x-y=w627:i16)
            n323 = Subtract(x=w629, y=w632) -> (x-y=w626:i16)
            n324 = Build Array(w609, w612, w613, w614) -> (w615:i16[])
            n325 = To Double Precision Float(number=w609) -> (double precision float=w610:dbl)
            n326 = Array Max & Min(array=w615) -> (min value=w611:i16)  [unwired: 3 out]
            n327 = To Double Precision Float(number=w627) -> (double precision float=w625:dbl)
            n328 = To Double Precision Float(number=w626) -> (double precision float=w624:dbl)
            n329 = Divide(x=w610, y=148.96908) -> (x/y=w605:dbl)
            n330 = To Double Precision Float(number=w611) -> (double precision float=w607:dbl)
            n331 = Multiply(x=w624, y=0.005) -> (x*y=→"Yaw" →"Yaw Rear":dbl)
            n332 = Multiply(x=w625, y=0.0001274) -> (x*y=→"Acc Y":dbl)
            n333 = Multiply(x=w605, y=0.227) -> (x*y=w604:dbl)
            n334 = Divide(x=w607, y=677.4732) -> ()  [unwired: 1 out]
            n335 = Subtract(x=w604, y=w607) -> (x-y=w606:dbl)
            n336 = Divide(x=w606, y=w604) -> (x/y=→"Slip":dbl)
          }
          frame 376 {
            w686 = i16 -32768
            # "Acceleration X & Roll"
            n337 = local read "IsStopped"() -> (w652:bool)
            n338 = Index Array(array=w691, index=7) -> (element=w690:u8)
            n339 = Index Array(array=w691, index=6) -> (element=w687:u8)
            n340 = Index Array(array=w691, index=3) -> (element=w689:u8)
            n341 = Index Array(array=w691, index=2) -> (element=w688:u8)
            n342 = case shown="True" w652 {
              frame False {
              }
              frame True {
                n343 = feedback #2() -> (w703:dbl)  [unwired: 1 in]
                n344 = local read "OffsetFilter"() -> (w701:dbl)
                n345 = local read "Roll"() -> (w704:dbl)
                n346 = formula code="y_=a*x+(1-a)*y;"("x"=w704, "y"=w703, "a"=w701) -> ("y_"=w702:dbl)
                n347 = feedback-in #2(w702) -> ()
                n348 = local write "Rollrate offset"(w702) -> ()
              }
            }
            n349 = Join Numbers(hi=w690, lo=w687) -> ((hi.lo)=w684:u16)
            n350 = Join Numbers(hi=w689, lo=w688) -> ((hi.lo)=w682:u16)
            n351 = feedback #3() -> (w657:dbl)  [unwired: 1 in]
            n352 = feedback #4() -> (w674:dbl[])  [unwired: 1 in]
            n353 = feedback #5() -> (w660:dbl)  [unwired: 1 in]
            n354 = feedback #6() -> (w667:dbl[])  [unwired: 1 in]
            n355 = local read "Acc Y"() -> (w655:dbl)
            n356 = local read "Acc Z"() -> (w659:dbl)
            n357 = formula code="y_=a*x+(1-a)*y;"("x"=w655, "y"=w657, "a"=0.02 ("input variable")) -> ("y_"=w654:dbl)
            "accY" <- w654
            n358 = feedback-in #3(w654) -> ()
            n359 = formula code="y_=a*x+(1-a)*y;"("x"=w659, "y"=w660, "a"=0.02 ("input variable")) -> ("y_"=w653:dbl)
            "accZ" <- w653
            n360 = feedback-in #5(w653) -> ()
            n361 = To Word Integer(number=w684) -> (16bit integer=w685:i16)
            n362 = To Word Integer(number=w682) -> (16bit integer=w683:i16)
            n363 = Subtract(x=w685, y=w686) -> (x-y=w681:i16)
            n364 = Subtract(x=w683, y=w686) -> (x-y=w680:i16)
            n365 = To Double Precision Float(number=w681) -> (double precision float=w679:dbl)
            n366 = To Double Precision Float(number=w680) -> (double precision float=w678:dbl)
            n367 = Build Array (concatenate)(w667, w653) -> (w668:dbl[])
            n368 = Build Array (concatenate)(w674, w654) -> (w672:dbl[])
            n369 = Build Array(w654) -> (w665:dbl[])
            n370 = Build Array(w653) -> (w664:dbl[])
            n371 = Multiply(x=w678, y=0.005) -> (x*y=→"Roll":dbl)
            n372 = Multiply(x=w679, y=0.0001274) -> (x*y=→"Acc X":dbl)
            n373 = Array Size(array=w672) -> (size(s)=w671:i32)
            n374 = Bundle(w665, w664) -> (w661:cluster{dbl[], dbl[]})  [unwired: 1 in]
            n375 = Less?(x=w671, y=1000) -> (x < y?=w669:bool)
            n376 = case shown="False" w669 {
              tunnel: [w705 w714] -> w666
              tunnel: w668 -> [w706 w714]
              tunnel: [w709 w713] -> w673
              tunnel: w672 -> [w712 w713]
              frame False {
                n377 = Delete From Array(array=w712, length=1, index=0) -> (array with subset deleted=w709:dbl[])  [unwired: 1 out]
                n378 = Delete From Array(array=w706, length=1, index=0) -> (array with subset deleted=w705:dbl[])  [unwired: 1 out]
              }
              frame True {
              }
            }
            n379 = feedback-in #4(w673) -> ()
            n380 = feedback-in #6(w666) -> ()
            n381 = Bundle(w673, w666) -> (w662:cluster{dbl[], dbl[]})  [unwired: 1 in]
            n382 = Build Array(w661, w662) -> (→"XY Graph":cluster{dbl[], dbl[]}[])
          }
          frame 380 {
            # "Acceleration Z"
            n383 = local read "AccelXRaw"() -> (w723:dbl)
            n384 = local read "IsStopped"() -> (w724:bool)
            n385 = local read "TorqRaw"() -> (w720:u16)
            n386 = Index Array(array=w739, index=7) -> (element=w738:u8)
            n387 = Index Array(array=w739, index=6) -> (element=w737:u8)
            n388 = case shown="True" w724 {
              frame False {
              }
              frame True {
                n389 = feedback #7() -> (w751:dbl)  [unwired: 1 in]
                n390 = local read "OffsetFilter"() -> (w749:dbl)
                n391 = local read "Acc Z"() -> (w752:dbl)
                n392 = formula code="y_=a*x+(1-a)*y;"("x"=w752, "y"=w751, "a"=w749) -> ("y_"=w750:dbl)
                n393 = feedback-in #7(w750) -> ()
                n394 = local write "Acc Z offset"(w750) -> ()
              }
            }
            n395 = Less?(x=w720, y=u16 200) -> (x < y?=w718:bool)
            n396 = Join Numbers(hi=w738, lo=w737) -> ((hi.lo)=w734:u16)
            n397 = Multiply(x=0.01, y=w723) -> (x*y=w729:dbl)
            n398 = local read "Velocity [km/h]"() -> (w726:dbl)
            n399 = And(x=w718, y=TRUE) -> (x .and. y?=w717:bool)
            n400 = To Word Integer(number=w734) -> (16bit integer=w735:i16)
            n401 = Divide(x=w726, y=3.6) -> (x/y=w716:dbl)
            n402 = Subtract(x=w735, y=i16 -32768) -> (x-y=w733:i16)
            n403 = feedback #8(w716) -> (w730:dbl)
            n404 = Add(x=w730, y=w729) -> (x+y=w722:dbl)
            n405 = case shown="True" w717 {
              tunnel: w722 -> [w747 _]
              tunnel: [w747 w748] -> w721
              tunnel: w716 -> [_ w748]
              frame False {
              }
              frame True {
              }
            }
            "Vel_acc" <- w721
            n406 = feedback-in #8(w721) -> ()
            n407 = To Double Precision Float(number=w733) -> (double precision float=w732:dbl)
            n408 = Multiply(x=w732, y=0.0001274) -> (x*y=→"Acc Z":dbl)
          }
          frame 389 {
            # "TCU FL"
            n409 = Index Array(array=w760, index=7) -> (element=w781:u8)
            n410 = Index Array(array=w760, index=6) -> (element=w780:u8)
            n411 = Index Array(array=w760, index=9) -> (element=w777:u8)
            n412 = Index Array(array=w760, index=8) -> (element=w776:u8)
            n413 = Index Array(array=w760, index=5) -> (element=w759:u8)
            n414 = Index Array(array=w760, index=4) -> (element=w758:u8)
            n415 = Index Array(array=w760, index=3) -> (element=w765:u8)
            n416 = Join Numbers(hi=w781, lo=w780) -> ((hi.lo)=w767:u16)
            n417 = Join Numbers(hi=w777, lo=w776) -> ((hi.lo)=w769:u16)
            n418 = Join Numbers(hi=w759, lo=w758) -> ((hi.lo)=w757:u16)
            n419 = Number To Boolean Array(number=w765) -> (Boolean array=→"TCU FL Status":bool[])
            n420 = To Word Integer(number=w767) -> (16bit integer=w770:i16)
            n421 = To Word Integer(number=w769) -> (16bit integer=w768:i16)
            n422 = To Word Integer(number=w757) -> (16bit integer=w756:i16)
            n423 = To Double Precision Float(number=w756) -> (double precision float=→"FL Velocity":dbl)
            n424 = To Double Precision Float(number=w770) -> (double precision float=w754:dbl)
            "FL" <- w754
            "FL Torque Pos" <- w754
            n425 = To Double Precision Float(number=w768) -> (double precision float=w753:dbl)
            "FL 2" <- w753
            "FL Torque Neg" <- w753
            n426 = Add(x=w754, y=w753) -> (x+y=→"TCU FL":dbl)
          }
          frame 390 {
            # "TCU FR"
            n427 = Index Array(array=w787, index=7) -> (element=w812:u8)
            n428 = Index Array(array=w787, index=6) -> (element=w811:u8)
            n429 = Index Array(array=w787, index=9) -> (element=w808:u8)
            n430 = Index Array(array=w787, index=8) -> (element=w807:u8)
            n431 = Index Array(array=w787, index=5) -> (element=w791:u8)
            n432 = Index Array(array=w787, index=4) -> (element=w790:u8)
            n433 = Index Array(array=w787, index=3) -> (element=w796:u8)
            n434 = Join Numbers(hi=w812, lo=w811) -> ((hi.lo)=w800:u16)
            n435 = Join Numbers(hi=w808, lo=w807) -> ((hi.lo)=w798:u16)
            n436 = Join Numbers(hi=w791, lo=w790) -> ((hi.lo)=w789:u16)
            n437 = Number To Boolean Array(number=w796) -> (Boolean array=→"TCU FR Status":bool[])
            n438 = To Word Integer(number=w800) -> (16bit integer=w801:i16)
            n439 = To Word Integer(number=w798) -> (16bit integer=w799:i16)
            n440 = To Word Integer(number=w789) -> (16bit integer=w788:i16)
            n441 = To Double Precision Float(number=w788) -> (double precision float=→"FR Velocity":dbl)
            n442 = To Double Precision Float(number=w801) -> (double precision float=w785:dbl)
            "FR" <- w785
            "FR Torque Pos" <- w785
            n443 = To Double Precision Float(number=w799) -> (double precision float=w784:dbl)
            "FR 2" <- w784
            "FR Torque Neg" <- w784
            n444 = Add(x=w785, y=w784) -> (x+y=→"TCU FR":dbl)
          }
          frame 393 {
            # "TCU RL"
            n445 = Index Array(array=w818, index=7) -> (element=w843:u8)
            n446 = Index Array(array=w818, index=6) -> (element=w842:u8)
            n447 = Index Array(array=w818, index=9) -> (element=w839:u8)
            n448 = Index Array(array=w818, index=8) -> (element=w838:u8)
            n449 = Index Array(array=w818, index=5) -> (element=w822:u8)
            n450 = Index Array(array=w818, index=4) -> (element=w821:u8)
            n451 = Index Array(array=w818, index=3) -> (element=w827:u8)
            n452 = Join Numbers(hi=w843, lo=w842) -> ((hi.lo)=w830:u16)
            n453 = Join Numbers(hi=w839, lo=w838) -> ((hi.lo)=w829:u16)
            n454 = Join Numbers(hi=w822, lo=w821) -> ((hi.lo)=w820:u16)
            n455 = Number To Boolean Array(number=w827) -> (Boolean array=→"TCU RL Status":bool[])
            n456 = To Word Integer(number=w830) -> (16bit integer=w832:i16)
            n457 = To Word Integer(number=w829) -> (16bit integer=w831:i16)
            n458 = To Word Integer(number=w820) -> (16bit integer=w819:i16)
            n459 = To Double Precision Float(number=w819) -> (double precision float=→"RL Velocity":dbl)
            n460 = To Double Precision Float(number=w832) -> (double precision float=w816:dbl)
            "RL" <- w816
            "RL Torque Pos" <- w816
            n461 = To Double Precision Float(number=w831) -> (double precision float=w815:dbl)
            "RL 2" <- w815
            "RL Torque Neg" <- w815
            n462 = Add(x=w816, y=w815) -> (x+y=→"TCU RL":dbl)
          }
          frame 394 {
            # "TCU RR"
            n463 = Index Array(array=w849, index=7) -> (element=w874:u8)
            n464 = Index Array(array=w849, index=6) -> (element=w873:u8)
            n465 = Index Array(array=w849, index=9) -> (element=w870:u8)
            n466 = Index Array(array=w849, index=8) -> (element=w869:u8)
            n467 = Index Array(array=w849, index=5) -> (element=w853:u8)
            n468 = Index Array(array=w849, index=4) -> (element=w852:u8)
            n469 = Index Array(array=w849, index=3) -> (element=w858:u8)
            n470 = Join Numbers(hi=w874, lo=w873) -> ((hi.lo)=w860:u16)
            n471 = Join Numbers(hi=w870, lo=w869) -> ((hi.lo)=w866:u16)
            n472 = Join Numbers(hi=w853, lo=w852) -> ((hi.lo)=w851:u16)
            n473 = Number To Boolean Array(number=w858) -> (Boolean array=→"TCU RR Status":bool[])
            n474 = To Word Integer(number=w860) -> (16bit integer=w861:i16)
            n475 = To Word Integer(number=w866) -> (16bit integer=w865:i16)
            n476 = To Word Integer(number=w851) -> (16bit integer=w850:i16)
            n477 = To Double Precision Float(number=w850) -> (double precision float=→"RR Velocity":dbl)
            n478 = To Double Precision Float(number=w861) -> (double precision float=w847:dbl)
            "RR" <- w847
            "RR Torque Pos" <- w847
            n479 = To Double Precision Float(number=w865) -> (double precision float=w846:dbl)
            "RR 2" <- w846
            "RR Torque Neg" <- w846
            n480 = Add(x=w847, y=w846) -> (x+y=→"TCU RR":dbl)
          }
          frame 436 {
            w889 = i16 -32768
            # "Acceleration Y & Yaw"
            n481 = Index Array(array=w894, index=7) -> (element=w893:u8)
            n482 = Index Array(array=w894, index=6) -> (element=w890:u8)
            n483 = Index Array(array=w894, index=3) -> (element=w892:u8)
            n484 = Index Array(array=w894, index=2) -> (element=w891:u8)
            n485 = Join Numbers(hi=w893, lo=w890) -> ((hi.lo)=w887:u16)
            n486 = Join Numbers(hi=w892, lo=w891) -> ((hi.lo)=w885:u16)
            n487 = To Word Integer(number=w887) -> (16bit integer=w888:i16)
            n488 = To Word Integer(number=w885) -> (16bit integer=w886:i16)
            n489 = Subtract(x=w888, y=w889) -> (x-y=w884:i16)
            n490 = Subtract(x=w886, y=w889) -> (x-y=w883:i16)
            n491 = To Double Precision Float(number=w884) -> (double precision float=w882:dbl)
            n492 = To Double Precision Float(number=w883) -> (double precision float=w881:dbl)
            n493 = Multiply(x=w881, y=0.005) -> (x*y=→"Yaw 2" →"Yaw Front":dbl)
            n494 = Multiply(x=w882, y=0.0001274) -> (x*y=→"Acc Y 2":dbl)
          }
          frame 440 {
            w918 = i16 -32768
            # "Acceleration X & Roll"
            n495 = local read "Data Source"() -> (w905:u16)
            n496 = local read "IsStopped"() -> (w906:bool)
            n497 = Index Array(array=w923, index=7) -> (element=w922:u8)
            n498 = Index Array(array=w923, index=6) -> (element=w919:u8)
            n499 = Index Array(array=w923, index=3) -> (element=w921:u8)
            n500 = Index Array(array=w923, index=2) -> (element=w920:u8)
            n501 = case shown="True" w906 {
              frame False {
              }
              frame True {
                n502 = feedback #9() -> (w1033:dbl)  [unwired: 1 in]
                n503 = local read "OffsetFilter"() -> (w1031:dbl)
                n504 = local read "Acc X 2"() -> (w1034:dbl)
                n505 = formula code="y_=a*x+(1-a)*y;"("x"=w1034, "y"=w1033, "a"=w1031) -> ("y_"=w1032:dbl)
                n506 = feedback-in #9(w1032) -> ()
                n507 = local write "Acc X offset 2"(w1032) -> ()
              }
            }
            n508 = case shown="2" w905 {
              frame 0, Default {
              }
              frame 2 {
                (unwired) cluster{dbl, u32}[] [{-1.5, 255}, {0.0, 61192}, {1.5, 16711680}] ("Z Scale.Marker Values[]")
                w936 = 500 ("dimension size")
                n509 = feedback #10() -> (w966:dbl)  [unwired: 1 in]
                n510 = feedback #11(0.0) -> (w958:dbl)
                n511 = Greater?(x=w958, y=200.0) -> (0:w962:bool)
                n512 = local read "Acc Z 2"() -> (w940:dbl)
                n513 = local read "Roll 2"() -> (w964:dbl)
                n514 = Initialize Array(-100.0 ("element"), w936, w936) -> (w935:dbl[][])
                n515 = formula code="y_=a*x+(1-a)*y;"("x"=w964, "y"=w966, "a"=0.5 ("input variable")) -> ("y_"=w963:dbl)
                n516 = feedback-in #10(w963) -> ()
                n517 = feedback #12(dbl[] []) -> (w980:dbl[])
                n518 = feedback #13(dbl[] []) -> (w979:dbl[])
                n519 = feedback #14(dbl[] []) -> (w941:dbl[])
                n520 = local read "Velocity [km/h]"() -> (w972:dbl)
                n521 = Build Array (concatenate)(w941, w940) -> (w933:dbl[])
                n522 = feedback-in #14(w933) -> ()
                n523 = Divide(x=w972, y=3.6) -> (x/y=w974:dbl)
                n524 = Subtract(x=w963, y="Rollrate offset") -> (x-y=w965:dbl)
                n525 = feedback #15() -> (w985:dbl)  [unwired: 1 in]
                n526 = feedback #16() -> (w983:dbl)  [unwired: 1 in]
                n527 = Divide(x=w965, y=180.0 ("Yaw")) -> (x/y=w971:dbl)
                n528 = feedback #17() -> (w986:dbl)  [unwired: 1 in]
                n529 = Multiply(x=3.141592653589793, y=w971) -> (x*y=w969:dbl)
                n530 = formula code="ve=v*cos(phi);\nvn=v*sin(phi);\nse=sx+ve*ts;\nsn=sy+vn*ts;\nphi_=phi+yaw*ts;"("phi"=w983, "yaw"=w969, "ts"=0.01 ("input variable"), "sx"=w986, "sy"=w985, "v"=w974) -> ("se"=w981:dbl, "sn"=w978:dbl, "phi_"=w984:dbl)  [unwired: 4 out]
                n531 = feedback-in #15(w978) -> ()
                n532 = feedback-in #16(w984) -> ()
                n533 = feedback-in #17(w981) -> ()
                n534 = Build Array (concatenate)(w980, w981) -> (w956:dbl[])
                n535 = feedback-in #12(w956) -> ()
                n536 = Build Array (concatenate)(w979, w978) -> (w955:dbl[])
                n537 = feedback-in #13(w955) -> ()
                n538 = Bundle(w956, w955) -> (→"XY Graph 2":cluster{dbl[], dbl[]})  [unwired: 1 in]
                n539 = feedback #18() -> (w949:dbl)  [unwired: 1 in]
                n540 = feedback #19() -> (w945:dbl)  [unwired: 1 in]
                n541 = feedback #20() -> (w947:dbl)  [unwired: 1 in]
                n542 = case shown="True" w962 {
                  tunnel: w956 -> [_ w1030]
                  tunnel: w955 -> [_ w1029]
                  tunnel: [w995 0.0] -> w960
                  tunnel: w958 -> [w996 _]
                  tunnel: [w994 w1010] -> w950
                  tunnel: [w992 w1009] -> w946
                  tunnel: [w993 w1008] -> w948
                  tunnel: w949 -> [w994 _]
                  tunnel: w947 -> [w993 _]
                  tunnel: w945 -> [w992 _]
                  tunnel: w933 -> [_ w997]
                  frame False {
                    n543 = Increment(x=w996) -> (x+1=w995:dbl)
                  }
                  frame True {
                    n544 = Array Max & Min(array=w997) -> (max value=w1007:dbl, min value=w1006:dbl)  [unwired: 2 out]
                    n545 = Array Max & Min(array=w1030) -> (max value=w1024:dbl, min value=w1025:dbl)  [unwired: 2 out]
                    n546 = Array Max & Min(array=w1029) -> (max value=w1016:dbl, min value=w1015:dbl)  [unwired: 2 out]
                    n547 = Add(x=w1024, y=w1025) -> (x+y=w1023:dbl)
                    n548 = Subtract(x=w1024, y=w1025) -> (x-y=w1028:dbl)
                    n549 = Subtract(x=w1016, y=w1015) -> (x-y=w1027:dbl)
                    n550 = Add(x=w1016, y=w1015) -> (x+y=w1017:dbl)
                    n551 = Bundle(w1007, u32 16711680) -> (w1005:cluster{dbl, u32})  [unwired: 1 in]
                    n552 = Bundle(w1006, u32 255) -> (w1003:cluster{dbl, u32})  [unwired: 1 in]
                    n553 = Build Array(w1028, w1027) -> (w1026:dbl[])
                    n554 = Divide(x=w1023, y=2.0) -> (x/y=w1020:dbl)
                    n555 = Divide(x=w1017, y=2.0) -> (x/y=w1013:dbl)
                    n556 = Bundle("y"=0.0, u32 6618880) -> (w1004:cluster{"y":dbl, u32})  [unwired: 1 in]
                    n557 = Build Array(w1003, w1004, w1005) -> (w998:cluster{"y":dbl, u32}[])
                    n558 = Array Max & Min(array=w1026) -> (max value=w1008:dbl)  [unwired: 3 out]
                    n559 = property on="Intensity Graph" class="IntGraph (strict)"("ZScale.MarkerVals[]"=w998) -> ()  [unwired: 2 in, 2 out]
                    n560 = Divide(x=w1008, y=2.0) -> (x/y=w1012:dbl)
                    n561 = Add(x=w1020, y=w1012) -> (x+y=w1019:dbl)
                    n562 = Add(x=w1013, y=w1012) -> (x+y=w1014:dbl)
                    n563 = Subtract(x=w1020, y=w1012) -> (x-y=w1010:dbl)
                    n564 = Subtract(x=w1013, y=w1012) -> (x-y=w1009:dbl)
                    n565 = property on="XY Graph 2" class="XYGraph (strict)"("XScale.Maximum"=w1019) -> ()  [unwired: 2 in, 2 out]
                    n566 = property on="XY Graph 2" class="XYGraph (strict)"("XScale.Minimum"=w1010) -> ()  [unwired: 2 in, 2 out]
                    n567 = property on="XY Graph 2" class="XYGraph (strict)"("YScale.Maximum"=w1014) -> ()  [unwired: 2 in, 2 out]
                    n568 = property on="XY Graph 2" class="XYGraph (strict)"("YScale.Minimum"=w1009) -> ()  [unwired: 2 in, 2 out]
                  }
                }
                n569 = feedback-in #11(w960) -> ()
                n570 = feedback-in #18(w950) -> ()
                n571 = feedback-in #19(w946) -> ()
                n572 = feedback-in #20(w948) -> ()
                n573 = Subtract(x=w956, y=w950) -> (x-y=w954:dbl[])
                n574 = Subtract(x=w955, y=w946) -> (x-y=w953:dbl[])
                n575 = Divide(x=w948, y=500.0) -> (x/y=w951:dbl)
                n576 = Divide(x=w954, y=w951) -> (x/y=w944:dbl[])
                n577 = Divide(x=w953, y=w951) -> (x/y=w943:dbl[])
                n578 = Round To Nearest(number=w944) -> (nearest integer value=w939:dbl[])
                n579 = Round To Nearest(number=w943) -> (nearest integer value=w938:dbl[])
                n580 = for {
                  tunnel: w939 -> [w991] mode=indexing
                  tunnel: w938 -> [w990] mode=indexing
                  tunnel: w933 -> [w989] mode=indexing
                  shift-right: [w987] -> w934
                  shift-left: w935 -> [w988]
                  n581 = Replace Array Subset(array=w988, new element=w989, index (row)=w991, index (col)=w990) -> (w987:dbl[][])
                }
                "Intensity Graph" <- w934
              }
            }
            n582 = Join Numbers(hi=w922, lo=w919) -> ((hi.lo)=w916:u16)
            n583 = Join Numbers(hi=w921, lo=w920) -> ((hi.lo)=w914:u16)
            n584 = To Word Integer(number=w916) -> (16bit integer=w917:i16)
            n585 = To Word Integer(number=w914) -> (16bit integer=w915:i16)
            n586 = Subtract(x=w917, y=w918) -> (x-y=w913:i16)
            n587 = Subtract(x=w915, y=w918) -> (x-y=w912:i16)
            n588 = To Double Precision Float(number=w913) -> (double precision float=w911:dbl)
            n589 = To Double Precision Float(number=w912) -> (double precision float=w910:dbl)
            n590 = Multiply(x=w910, y=0.005) -> (x*y=→"Roll 2":dbl)
            n591 = Multiply(x=w911, y=0.0001274) -> (x*y=→"Acc X 2":dbl)
          }
          frame 444 {
            # "Acceleration Z"
            n592 = Index Array(array=w1044, index=7) -> (element=w1043:u8)
            n593 = Index Array(array=w1044, index=6) -> (element=w1042:u8)
            n594 = Join Numbers(hi=w1043, lo=w1042) -> ((hi.lo)=w1039:u16)
            n595 = To Word Integer(number=w1039) -> (16bit integer=w1040:i16)
            n596 = Subtract(x=w1040, y=i16 -32768) -> (x-y=w1038:i16)
            n597 = To Double Precision Float(number=w1038) -> (double precision float=w1037:dbl)
            n598 = Multiply(x=w1037, y=0.0001274) -> (x*y=→"Acc Z 2":dbl)
          }
          frame 402 {
            n599 = Index Array(array=w1066, index=2) -> (element=w1055:u8)
            n600 = Number To Boolean Array(number=w1055) -> (Boolean array=w1064:bool[])
            n601 = Index Array(array=w1064, index #1=7 ("index"), index #2=6 ("index"), index #3=5 ("index"), index #4=4 ("index"), index #5=3 ("index"), index #6=2 ("index"), index #7=1 ("index"), index #8=0 ("index")) -> (element #6=→"RES BUTTON":bool, element #7=→"RES GO":bool, element #8=→"RES EBS":bool)  [unwired: 5 out]
          }
          frame 512 {
            # "Torque signal"
            # "Pedalbox Throttle Steering"
            n602 = Index Array(array=w1074, index=6) -> (element=w1081:u8)
            n603 = Index Array(array=w1074, index=7) -> (element=w1080:u8)
            n604 = Index Array(array=w1074, index=4) -> (element=w1092:u8)
            n605 = Index Array(array=w1074, index=5) -> (element=w1091:u8)
            n606 = Index Array(array=w1074, index=2) -> (element=w1087:u8)
            n607 = Index Array(array=w1074, index=3) -> (element=w1086:u8)
            n608 = formula code="out = (in1 << 8) | in2;"("in1"=w1081, "in2"=w1080) -> ("out"=→"STA1":dbl)
            n609 = formula code="out = (in1 << 8) | in2;"("in1"=w1092, "in2"=w1091) -> ("out"=→"TPS2_Raw":dbl)
            n610 = formula code="out = (in1 << 8) | in2;"("in1"=w1087, "in2"=w1086) -> ("out"=→"TorqRaw 2" →"TPS1_Raw":dbl)
            n611 = Subtract(x="Torque Max", y="Torque Min") -> (x-y=w1103:dbl)
            n612 = Join Numbers(hi=w1092, lo=w1091) -> ((hi.lo)=w1093:u16)
            n613 = Subtract(x=w1093, y="Torque Min") -> (x-y=w1104:dbl)
            n614 = Index Array(array=w1074, index=8) -> (element=w1076:u8)
            n615 = Index Array(array=w1074, index=9) -> (element=w1075:u8)
            n616 = case shown="1" u16 1 ("y") {
              tunnel: w1074 -> [w1111 w1134]
              tunnel: [i16 0 ("STA1") w1129] -> _
              tunnel: [i16 0 ("STA1") w1124] -> _
              tunnel: [w1108 w1125] -> _
              tunnel: [w1107 i16 0 ("STA1")] -> w1090
              frame 0, Default {
                # "TCU 2016"
                n617 = Index Array(array=w1111, index=8) -> (element=w1114:u8)
                n618 = Index Array(array=w1111, index=9) -> (element=w1115:u8)
                n619 = Join Numbers(hi=w1114, lo=w1115) -> ((hi.lo)=w1107:u16)
                n620 = Subtract(x="Steering Max", y="Steering Min") -> (x-y=w1121:dbl)
                n621 = Subtract(x=w1107, y="Steering Null") -> (x-y=w1116:dbl)
                n622 = Divide(x=w1116, y=w1121) -> (x/y=w1117:dbl)
                n623 = Multiply(x=360.0, y=w1117) -> (x*y=w1108:dbl)
              }
              frame 1 {
                # "TCU 2017"
                n624 = Index Array(array=w1134, index=6) -> (element=w1140:u8)
                n625 = Index Array(array=w1134, index=7) -> (element=w1137:u8)
                n626 = Index Array(array=w1134, index=8) -> (element=w1133:u8)
                n627 = Index Array(array=w1134, index=9) -> (element=w1132:u8)
                n628 = Join Numbers(hi=w1133, lo=w1132) -> ((hi.lo)=w1130:u16)
                n629 = And(x=w1140, y=u8 127) -> (x .and. y?=w1139:u8)
                n630 = Subtract(x=w1130, y=i16 3600) -> (x-y=w1124:u16)
                n631 = Join Numbers(hi=w1139, lo=w1137) -> ((hi.lo)=w1138:u16)
                n632 = Subtract(x=w1138, y=i16 3600) -> (x-y=w1129:u16)
                n633 = To Word Integer(number=w1124) -> (16bit integer=w1127:i16)
                n634 = To Double Precision Float(number=w1127) -> (double precision float=w1126:dbl)
                n635 = Divide(x=w1126, y=10.0) -> (x/y=w1125:dbl)
              }
            }
            "SteeringRaw" <- w1090
            n636 = formula code="out = (in1 << 8) | in2;"("in1"=w1076, "in2"=w1075) -> ("out"=→"STA2":dbl)
            n637 = Divide(x=w1104, y=w1103) -> (x/y=w1100:dbl)
            n638 = Multiply(x=100.0, y=w1100) -> ()  [unwired: 1 out]
          }
          frame 513 {
            w1186 = 16.375 ("y")
            # "Pedalbox Brake"
            n639 = local read "Brake Force Threshold"() -> (w1150:u16)
            n640 = local read "TC Threshold"() -> (w1149:u8)
            n641 = Subtract(x="Brake Max", y="Brake Min") -> (x-y=w1216:dbl)
            n642 = Index Array(array=w1182, index=2) -> (element=w1177:u8)
            n643 = Index Array(array=w1182, index=4) -> (element=w1181:u8)
            n644 = Index Array(array=w1182, index=6) -> (element=w1207:u8)
            n645 = Index Array(array=w1182, index=8) -> (element=w1197:u8)
            n646 = Subtract(x="Brake Max 2", y="Brake Min 2") -> (x-y=w1205:dbl)
            n647 = Subtract(x="Brake Max 2", y="Brake Min 2") -> (x-y=w1195:dbl)
            n648 = Index Array(array=w1182, index=3) -> (element=w1175:u8)
            n649 = Index Array(array=w1182, index=5) -> (element=w1220:u8)
            n650 = Index Array(array=w1182, index=7) -> (element=w1200:u8)
            n651 = Index Array(array=w1182, index=9) -> (element=w1190:u8)
            n652 = feedback #21() -> (w1169:dbl[])  [unwired: 1 in]
            n653 = feedback #22() -> (w1162:dbl[])  [unwired: 1 in]
            n654 = And(x=w1177, y=u8 15) -> (x .and. y?=w1176:u8)
            n655 = And(x=w1181, y=u8 15) -> (x .and. y?=w1180:u8)
            n656 = And(x=w1207, y=u8 15) -> (x .and. y?=w1201:u8)
            n657 = And(x=w1197, y=u8 15) -> (x .and. y?=w1191:u8)
            n658 = Join Numbers(hi=w1176, lo=w1175) -> ((hi.lo)=→"BPS1_Raw":u16)
            n659 = feedback #23() -> (w1155:dbl)  [unwired: 1 in]
            n660 = Join Numbers(hi=w1180, lo=w1220) -> ((hi.lo)=w1173:u16)
            "BPS2_Raw" <- w1173
            n661 = Join Numbers(hi=w1201, lo=w1200) -> ((hi.lo)=w1171:u16)
            "BPR_Raw" <- w1171
            n662 = Join Numbers(hi=w1191, lo=w1190) -> ((hi.lo)=w1170:u16)
            "BrakeRaw 2" <- w1170
            "BPF_Raw" <- w1170
            n663 = feedback #24() -> (w1157:dbl)  [unwired: 1 in]
            n664 = Subtract(x=w1173, y="Brake Min") -> (x-y=w1217:dbl)
            n665 = Subtract(x=w1171, y="Brake Min 2") -> (x-y=w1185:dbl)
            n666 = Subtract(x=w1170, y="Brake Min 2") -> (x-y=w1172:dbl)
            n667 = local read "BP_front"() -> (w1146:i16)
            n668 = local read "BP_rear"() -> (w1145:i16)
            n669 = Divide(x=w1217, y=w1216) -> (x/y=w1215:dbl)
            n670 = Divide(x=w1185, y=w1205) -> (x/y=w1204:dbl)
            n671 = Divide(x=w1172, y=w1195) -> (x/y=w1194:dbl)
            n672 = Divide(x=w1185, y=w1186) -> ()  [unwired: 1 out]
            n673 = Divide(x=w1172, y=w1186) -> ()  [unwired: 1 out]
            n674 = Multiply(x=100.0, y=w1215) -> ()  [unwired: 1 out]
            n675 = formula code="y_=a*x+(1-a)*y;"("x"=w1146, "y"=w1155, "a"=0.02 ("input variable")) -> ("y_"=w1153:dbl)
            n676 = feedback-in #23(w1153) -> ()
            n677 = formula code="y_=a*x+(1-a)*y;"("x"=w1145, "y"=w1157, "a"=0.02 ("input variable")) -> ("y_"=w1152:dbl)
            "accZ 2" <- w1152
            n678 = feedback-in #24(w1152) -> ()
            n679 = Bundle("BP_front"=w1146, "BP_rear"=w1145, "Brake Force Threshold"=w1150, "TC Threshold"=w1149) -> (→"Brake Pressure":T7)  [unwired: 1 in]
            n680 = Multiply(x=100.0, y=w1204) -> (x*y=→"Brake Front":dbl)
            n681 = Multiply(x=100.0, y=w1194) -> (x*y=→"Brake Rear":dbl)
            n682 = Build Array (concatenate)(w1169, w1153) -> (w1167:dbl[])
            n683 = Build Array(w1153) -> (w1160:dbl[])
            n684 = Array Size(array=w1167) -> (size(s)=w1166:i32)
            n685 = Build Array (concatenate)(w1162, w1152) -> (w1163:dbl[])
            n686 = Build Array(w1152) -> (w1159:dbl[])
            n687 = Bundle(w1160, w1159) -> (w1147:cluster{dbl[], dbl[]})  [unwired: 1 in]
            n688 = Less?(x=w1166, y=1000) -> (x < y?=w1164:bool)
            n689 = case shown="False" w1164 {
              tunnel: [w1223 w1232] -> w1161
              tunnel: w1163 -> [w1224 w1232]
              tunnel: [w1227 w1231] -> w1168
              tunnel: w1167 -> [w1230 w1231]
              frame False {
                n690 = Delete From Array(array=w1230, length=1, index=0) -> (array with subset deleted=w1227:dbl[])  [unwired: 1 out]
                n691 = Delete From Array(array=w1224, length=1, index=0) -> (array with subset deleted=w1223:dbl[])  [unwired: 1 out]
              }
              frame True {
              }
            }
            n692 = feedback-in #21(w1168) -> ()
            n693 = feedback-in #22(w1161) -> ()
            n694 = Bundle(w1168, w1161) -> (w1158:cluster{dbl[], dbl[]})  [unwired: 1 in]
            n695 = Build Array(w1147, w1158) -> (→"XY Graph 3":cluster{dbl[], dbl[]}[])
          }
          frame 1026 {
            # "Pedalbox Brake"
            n696 = local read "BPS1_Raw"() -> (w1247:u16)
            n697 = local read "BPS2_Raw"() -> (w1246:u16)
            n698 = Index Array(array=w1251, index=2) -> (element=w1243:u8)
            n699 = Index Array(array=w1251, index=4) -> (element=w1237:u8)
            n700 = Index Array(array=w1251, index=6) -> (element=w1234:u8)
            n701 = Index Array(array=w1251, index=8) -> (element=w1240:u8)
            n702 = Index Array(array=w1251, index=3) -> (element=w1261:u8)
            n703 = Index Array(array=w1251, index=5) -> (element=w1254:u8)
            n704 = Index Array(array=w1251, index=7) -> (element=w1257:u8)
            n705 = Index Array(array=w1251, index=9) -> (element=w1260:u8)
            n706 = And(x=w1243, y=u8 15) -> (x .and. y?=w1242:u8)
            n707 = And(x=w1237, y=u8 15) -> (x .and. y?=w1236:u8)
            n708 = And(x=w1234, y=u8 15) -> (x .and. y?=w1233:u8)
            n709 = And(x=w1240, y=u8 15) -> (x .and. y?=w1239:u8)
            n710 = Join Numbers(hi=w1242, lo=w1261) -> ((hi.lo)=w1250:u16)
            n711 = Join Numbers(hi=w1236, lo=w1254) -> ((hi.lo)=w1249:u16)
            n712 = Join Numbers(hi=w1233, lo=w1257) -> ((hi.lo)=w1245:u16)
            n713 = Join Numbers(hi=w1239, lo=w1260) -> ((hi.lo)=w1248:u16)
            n714 = Bundle(w1250, w1249, "BPS1_Raw"=w1247, "BPS2_Raw"=w1246, w1245, w1248) -> ()  [unwired: 1 in, 1 out]
          }
          frame 1027 {
            # "Pedalbox Brake"
            n715 = Index Array(array=w1281, index=6) -> (element=w1279:u8)
            n716 = Index Array(array=w1281, index=7) -> (element=w1288:u8)
            n717 = Index Array(array=w1281, index=4) -> (element=w1276:u8)
            n718 = Index Array(array=w1281, index=5) -> (element=w1296:u8)
            n719 = Index Array(array=w1281, index=8) -> (element=w1273:u8)
            n720 = Index Array(array=w1281, index=9) -> (element=w1285:u8)
            n721 = Index Array(array=w1281, index=2) -> (element=w1270:u8)
            n722 = Index Array(array=w1281, index=3) -> (element=w1284:u8)
            n723 = And(x=w1279, y=u8 15) -> (x .and. y?=w1278:u8)
            n724 = And(x=w1276, y=u8 15) -> (x .and. y?=w1275:u8)
            n725 = And(x=w1273, y=u8 15) -> (x .and. y?=w1272:u8)
            n726 = And(x=w1270, y=u8 15) -> (x .and. y?=w1269:u8)
            n727 = Join Numbers(hi=w1278, lo=w1288) -> ()  [unwired: 1 out]
            n728 = Join Numbers(hi=w1275, lo=w1296) -> ()  [unwired: 1 out]
            n729 = Join Numbers(hi=w1272, lo=w1285) -> ()  [unwired: 1 out]
            n730 = Join Numbers(hi=w1269, lo=w1284) -> ()  [unwired: 1 out]
          }
          frame 528 {
            # "HV Cell Values"
            # "HV Accumulator"
            n731 = Index Array(array=w1351, index=5) -> (element=w1350:u8)
            n732 = Index Array(array=w1351, index=6) -> (element=w1349:u8)
            n733 = Index Array(array=w1351, index=3) -> (element=w1331:u8)
            n734 = Join Numbers(hi=w1350, lo=w1349) -> ((hi.lo)=w1327:u16)
            n735 = Index Array(array=w1351, index=4) -> (element=w1357:u8)
            n736 = And(x=w1331, y=u8 127) -> (x .and. y?=w1329:u8)
            n737 = Join Numbers(hi=w1329, lo=w1357) -> ((hi.lo)=w1356:u16)
            n738 = Index Array(array=w1351, index=2) -> (element=w1332:u8)
            n739 = Divide(x=w1327, y=10.0) -> (x/y=w1328:dbl)
            n740 = Replace Array Subset(array=w1355, new element=w1356, index=w1332) -> (w1325:u16[])
            n741 = Replace Array Subset(array=w1348, new element=w1328, index=w1332) -> (w1301:dbl[])
            n742 = Array Subset(array=w1301, index=0, length=28) -> (→"Temp 1":dbl[])
            n743 = Array Subset(array=w1301, index=84, length=28) -> (→"Temp 4":dbl[])
            n744 = Array Subset(array=w1301, index=56, length=28) -> (→"Temp 3":dbl[])
            n745 = Array Subset(array=w1301, index=28, length=28) -> (→"Temp 2":dbl[])
            n746 = Array Subset(array=w1301, index=0, length=180) -> (w1304:dbl[])
            n747 = Array Subset(array=w1301, index=140, length=28) -> (→"Temp 6":dbl[])
            n748 = Array Subset(array=w1301, index=112, length=28) -> (→"Temp 5":dbl[])
            n749 = call "Stack.vi"("Array"=w1325) -> ("Min"=→"Cell Min" →"HV Cell Voltage":u16, "Max"=→"Cell Max":u16, "appended array"=w1324:u16[], "appended array 2"=w1321:u16[], "appended array 3"=w1320:u16[], "appended array 4"=w1319:u16[], "appended array 5"=w1322:u16[], "appended array 6"=w1323:u16[])  [unwired: 11 in]
            n750 = for {
              tunnel: [w1372] -> w1354 mode=indexing
              tunnel: w1324 -> [w1371] mode=indexing
              tunnel: w1321 -> [w1369] mode=indexing
              tunnel: [w1370] -> w1317 mode=indexing
              tunnel: w1320 -> [w1368] mode=indexing
              tunnel: [w1367] -> w1316 mode=indexing
              tunnel: w1319 -> [w1366] mode=indexing
              tunnel: w1322 -> [w1365] mode=indexing
              tunnel: w1323 -> [w1364] mode=indexing
              tunnel: [w1363] -> w1315 mode=indexing
              tunnel: [w1362] -> w1314 mode=indexing
              tunnel: [w1361] -> w1313 mode=indexing
              n751 = Bundle(w1371, w1371) -> (w1372:cluster{u16, u16})  [unwired: 1 in]
              n752 = Bundle(w1369, w1369) -> (w1370:cluster{u16, u16})  [unwired: 1 in]
              n753 = Bundle(w1368, w1368) -> (w1367:cluster{u16, u16})  [unwired: 1 in]
              n754 = Bundle(w1366, w1366) -> (w1363:cluster{u16, u16})  [unwired: 1 in]
              n755 = Bundle(w1365, w1365) -> (w1362:cluster{u16, u16})  [unwired: 1 in]
              n756 = Bundle(w1364, w1364) -> (w1361:cluster{u16, u16})  [unwired: 1 in]
            }
            "Stack 1" <- w1354
            "Stack 2" <- w1317
            "Stack 3" <- w1316
            "Stack 4" <- w1315
            "Stack 5" <- w1314
            "Stack 6" <- w1313
            n757 = Array Max & Min(array=w1304) -> (max value=w1306:dbl, min value=w1307:dbl)  [unwired: 2 out]
            "Temp Max" <- w1306
            n758 = Bundle(w1306, w1307) -> (→"HV Cell Temperature":cluster{dbl, dbl})  [unwired: 1 in]
          }
          frame 532 {
            # "HV Battery Status"
            # "HV Battery Status"
            n759 = local read "HV Current"() -> (w1406:dbl)
            "Current" <- w1406
            n760 = local read "HV Before"() -> (w1407:dbl)
            n761 = local read "Cell Min"() -> (w1402:u16)
            n762 = local read "HV After"() -> (w1408:dbl)
            n763 = local read "TCU RR"() -> (w1390:dbl)
            n764 = local read "TCU FR"() -> (w1394:dbl)
            n765 = local read "TCU RL"() -> (w1392:dbl)
            n766 = local read "TCU FL"() -> (w1397:dbl)
            n767 = Index Array(array=w1431, index=6) -> (element=w1413:u8)
            n768 = Index Array(array=w1431, index=7) -> (element=w1412:u8)
            n769 = Index Array(array=w1431, index=4) -> (element=w1439:u8)
            n770 = Index Array(array=w1431, index=5) -> (element=w1438:u8)
            n771 = Index Array(array=w1431, index=8) -> (element=w1433:u8)
            n772 = Index Array(array=w1431, index=9) -> (element=w1432:u8)
            n773 = Index Array(array=w1431, index=2) -> (element=w1448:u8)
            n774 = Index Array(array=w1431, index=3) -> (element=w1447:u8)
            n775 = Join Numbers(hi=w1439, lo=w1438) -> ((hi.lo)=w1425:u16)
            n776 = Join Numbers(hi=w1433, lo=w1432) -> ((hi.lo)=w1420:u16)
            n777 = Join Numbers(hi=w1448, lo=w1447) -> ((hi.lo)=w1428:u16)
            n778 = To Unsigned Byte Integer(number=w1413) -> (unsigned 8bit integer=w1414:u8)
            n779 = To Unsigned Byte Integer(number=w1412) -> (unsigned 8bit integer=w1415:u8)
            n780 = Bundle("HV Before"=w1407, "HV After"=w1408) -> (→"HV Voltage":cluster{"HV Before":dbl, "HV After":dbl})  [unwired: 1 in]
            n781 = local read "Cell Max"() -> (w1403:u16)
            n782 = local read "Actual Velocity \nRR [RPM]"() -> (w1391:i16)
            n783 = Compound Arithmetic op=MULTIPLY(w1407, w1406, 0.001 ("value")) -> (w1383:dbl)
            n784 = local read "Actual Velocity\nFR [RPM]"() -> (w1395:i16)
            n785 = local read "Actual Velocity\nRL [RPM]"() -> (w1393:i16)
            n786 = local read "Actual Velocity\nFL [RPM]"() -> (w1396:i16)
            n787 = Join Numbers(hi=w1414, lo=w1415) -> ((hi.lo)=w1411:u16)
            n788 = To Double Precision Float(number=w1425) -> (double precision float=w1426:dbl)
            n789 = To Double Precision Float(number=w1420) -> (double precision float=w1421:dbl)
            n790 = To Double Precision Float(number=w1428) -> (double precision float=w1429:dbl)
            n791 = Bundle("Cell Max"=w1403, "Cell Min"=w1402) -> (→"HV Cell":cluster{"Cell Max":u16, "Cell Min":u16})  [unwired: 1 in]
            n792 = Multiply(x=w1396, y=w1397) -> (x*y=w1401:dbl)
            n793 = Multiply(x=w1395, y=w1394) -> (x*y=w1400:dbl)
            n794 = Multiply(x=w1393, y=w1392) -> (x*y=w1399:dbl)
            n795 = Multiply(x=w1391, y=w1390) -> (x*y=w1398:dbl)
            n796 = To Word Integer(number=w1411) -> (16bit integer=w1410:i16)
            n797 = Divide(x=w1421, y=1.0) -> (x/y=→"SoC [mAh]":dbl)
            n798 = Divide(x=w1426, y=10.0) -> (x/y=→"HV After":dbl)
            n799 = Divide(x=w1429, y=10.0) -> (x/y=→"HV Before":dbl)
            n800 = Compound Arithmetic op=ADD(w1401, w1400, w1399, w1398) -> (w1389:dbl)
            n801 = To Double Precision Float(number=w1410) -> (double precision float=w1423:dbl)
            n802 = Divide(x=w1383, y=3.6) -> (x/y=w1375:dbl)
            n803 = Divide(x=w1423, y=10.0) -> (x/y=→"HV Current":dbl)
            n804 = Multiply(x=0.005, y=w1375) -> (x*y=w1384:dbl)
            n805 = Compound Arithmetic op=MULTIPLY(w1389, 0.10472 ("x"), 0.0098 ("y"), 0.001 ("value")) -> (w1373:dbl)
            n806 = feedback #25() -> (w1379:dbl)  [unwired: 1 in]
            n807 = Add(x=w1379, y=w1384) -> (x+y=w1377:dbl)
            n808 = case shown="True" "New Lap" {
              tunnel: w1377 -> [w1451 _]
              tunnel: [w1451 0.0] -> w1376
              frame False {
              }
              frame True {
              }
            }
            n809 = feedback-in #25(w1376) -> ()
            n810 = Bundle(w1383, w1373) -> (→"Electric Power":cluster{dbl, dbl})  [unwired: 1 in]
            n811 = feedback #26() -> (w1380:dbl[])  [unwired: 1 in]
            n812 = case shown="False" "New Lap" {
              tunnel: w1377 -> [w1455 w1460]
              tunnel: [w1454 w1459] -> w1381
              tunnel: w1380 -> [w1453 w1458]
              frame False {
                n813 = Array Size(array=w1453) -> (size(s)=w1457:i32)
                n814 = Decrement(x=w1457) -> (x-1=w1456:i32)
                n815 = Replace Array Subset(array=w1453, new element=w1455, index=w1456) -> (w1454:dbl[])
              }
              frame True {
                n816 = Build Array (concatenate)(w1458, w1460) -> (w1459:dbl[])
              }
            }
            "Energy" <- w1381
            n817 = feedback-in #26(w1381) -> ()
          }
          frame 530 {
            # "ilyen nincs 18ban"
            # "ilyen nincs 18ban"
            # "ilyen nincs 18-ban"
            # "HV Accumulator Status"
            # "Accumulator Status"
            n818 = Index Array(array=w1484, index=3) -> (element=w1520:u8)
            n819 = Index Array(array=w1484, index=4) -> (element=w1510:u8)
            n820 = Index Array(array=w1484, index=5) -> (element=w1516:u8)
            n821 = Number To Boolean Array(number=w1520) -> (Boolean array=w1525:bool[])
            n822 = Number To Boolean Array(number=w1510) -> (Boolean array=w1509:bool[])
            n823 = Number To Boolean Array(number=w1516) -> (Boolean array=w1515:bool[])
            n824 = Index Array(array=w1525, index #1=7 ("index"), index #2=6 ("index"), index #3=5 ("index"), index #4=4 ("index"), index #5=3 ("index"), index #6=2 ("index"), index #7=1 ("index"), index #8=0 ("index")) -> (element #1=→"AMS error":bool, element #2=→"IMD error":bool, element #3=→"HVDet" →"HVDet":bool, element #4=→"AIR+" →"SC AIR+" →"AIR+":bool, element #5=→"AIR-" →"SC AIR-" →"AIR-":bool, element #6=→"SC Endline":bool, element #7=→"PC State" →"PC State 2":bool, element #8=→"TSAL State" →"TSAL State 2":bool)
            n825 = Index Array(array=w1509, index #1=7 ("index"), index #2=6 ("index"), index #3=5 ("index"), index #4=4 ("index"), index #5=3 ("index"), index #6=2 ("index"), index #7=1 ("index"), index #8=0 ("index")) -> (element #1=→"12V State" →"Driver Protection" →"SC 12V":bool, element #2=→"HV_ACC in menu":bool, element #3=→"TSAL Green":bool, element #4=→"AMS Relay" →"SC AMS" →"AMS Relay 2":bool, element #5=→"IMD Relay" →"SC IMD" →"IMD Relay":bool, element #6=→"TSAL Red":bool, element #7=w1465:bool, element #8=→"MCU HVDET":bool)
            n826 = Index Array(array=w1515, index #1=7 ("index"), index #2=6 ("index"), index #3=5 ("index"), index #4=4 ("index"), index #5=3 ("index"), index #6=2 ("index"), index #7=1 ("index"), index #8=0 ("index")) -> (element #1=→"TS-OC":bool, element #2=→"PC":bool, element #5=→"TS-OV":bool, element #6=→"OT":bool, element #7=→"OV":bool, element #8=→"UV":bool)  [unwired: 2 out]
            n827 = Not(x=w1465) -> (.not. x?=→"TSAL Error":bool)
            n828 = Index Array(array=w1484, index=7) -> (element=w1500:u8)
            n829 = Index Array(array=w1484, index=8) -> (element=w1499:u8)
            n830 = Index Array(array=w1484, index=6) -> (element=→"Place of Error":u8)
            n831 = Join Numbers(hi=w1500, lo=w1499) -> ((hi.lo)=→"Value":u16)
          }
          frame 560 {
            n832 = local read "Brake Force"() -> (w1551:u16)
            n833 = local read "BPFV"() -> (w1533:bool)
            n834 = local read "BPFSV"() -> (w1532:bool)
            n835 = Index Array(array=w1569, index=4) -> (element=w1539:u8)
            n836 = Index Array(array=w1569, index=2) -> (element=w1554:u8)
            n837 = Index Array(array=w1569, index=6) -> (element=w1560:u8)
            n838 = Index Array(array=w1569, index=8) -> (element=w1549:u8)
            n839 = Index Array(array=w1569, index=9) -> (element=w1568:u8)
            n840 = And(x=w1539, y=u8 15) -> (x .and. y?=w1540:u8)
            n841 = And(x=w1554, y=u8 15) -> (x .and. y?=w1557:u8)
            n842 = And(x=w1560, y=u8 15) -> (x .and. y?=w1559:u8)
            n843 = And(x=w1549, y=u8 15) -> (x .and. y?=w1548:u8)
            n844 = And(x=w1539, y=u8 240) -> (x .and. y?=w1542:u8)
            n845 = And(x=w1554, y=u8 240) -> (x .and. y?=w1555:u8)
            n846 = Join Numbers(hi=w1548, lo=w1568) -> ((hi.lo)=→"STA2_Raw":u16)
            n847 = Index Array(array=w1569, index=5) -> (element=w1578:u8)
            n848 = Index Array(array=w1569, index=7) -> (element=w1573:u8)
            n849 = Index Array(array=w1569, index=3) -> (element=w1585:u8)
            n850 = To Unsigned Byte Integer(number=w1540) -> (unsigned 8bit integer=w1579:u8)
            n851 = To Unsigned Byte Integer(number=w1557) -> (unsigned 8bit integer=w1584:u8)
            n852 = To Unsigned Byte Integer(number=w1559) -> (unsigned 8bit integer=w1574:u8)
            n853 = Number To Boolean Array(number=w1542) -> (Boolean array=w1562:bool[])
            n854 = Number To Boolean Array(number=w1555) -> (Boolean array=w1567:bool[])
            n855 = Join Numbers(hi=w1574, lo=w1573) -> ((hi.lo)=w1545:u16)
            n856 = Join Numbers(hi=w1579, lo=w1578) -> ((hi.lo)=→"APPS2" →"Apps2":u16)
            n857 = Join Numbers(hi=w1584, lo=w1585) -> ((hi.lo)=w1552:u16)
            "APPS1" <- w1552
            "Apps1" <- w1552
            "TorqRaw" <- w1552
            n858 = Index Array(array=w1562, index #1=7, index #2=6) -> (element #1=w1535:bool, element #2=w1534:bool)
            "STA1" <- w1535
            "STA2" <- w1534
            n859 = Index Array(array=w1567, index #1=6, index #2=7) -> (element #1=w1537:bool, element #2=w1536:bool)
            "TPS1V" <- w1537
            "TPS2V" <- w1536
            n860 = To Double Precision Float(number=w1545) -> (double precision float=w1544:dbl)
            "STA1_Raw" <- w1544
            n861 = local read "BPFV"() -> (w1531:bool)
            n862 = local read "BPRV"() -> (w1530:bool)
            n863 = Build Array(w1537, w1536, w1535, w1534, w1533, w1532, w1531, w1530) -> (→"Sensor Check":bool[])
            n864 = To Double Precision Float(number=w1552) -> (double precision float=w1582:dbl)
            n865 = Bundle(w1552, "Brake Force"=w1551) -> ()  [unwired: 1 in, 1 out]
            n866 = Subtract(x=w1544, y=u16 90) -> (x-y=→"Steering Angle":dbl)
            n867 = Multiply(x=0.1, y=w1582) -> (x*y=→"Torque":dbl)
          }
          frame 561 {
            w1627 = 0
            w1629 = 4
            w1618 = 5
            w1617 = 6
            w1614 = 7
            n868 = Index Array(array=w1599, index=w1629) -> (element=w1593:u8)
            n869 = Index Array(array=w1599, index=w1614) -> ()  [unwired: 1 out]
            n870 = Index Array(array=w1599, index=w1617) -> (element=w1620:u8)
            n871 = Index Array(array=w1599, index=2) -> (element=w1611:u8)
            n872 = Index Array(array=w1599, index=6) -> (element=w1594:u8)
            n873 = Index Array(array=w1599, index=8) -> (element=w1595:u8)
            n874 = Index Array(array=w1599, index=3) -> (element=w1632:u8)
            n875 = Index Array(array=w1599, index=7) -> (element=w1605:u8)
            n876 = Index Array(array=w1599, index=9) -> (element=w1600:u8)
            n877 = Split Number(x=w1611) -> (lo(x)=w1631:u8)  [unwired: 1 out]
            n878 = Split Number(x=w1593) -> (lo(x)=w1628:u8)  [unwired: 1 out]
            n879 = And(x=w1611, y=u8 15) -> (x .and. y?=w1610:u8)
            n880 = And(x=w1594, y=u8 15) -> (x .and. y?=w1606:u8)
            n881 = And(x=w1595, y=u8 15) -> (x .and. y?=w1601:u8)
            n882 = Number To Boolean Array(number=w1611) -> (Boolean array=w1641:bool[])
            n883 = Number To Boolean Array(number=w1595) -> (Boolean array=w1615:bool[])
            n884 = Number To Boolean Array(number=w1620) -> (Boolean array=w1619:bool[])
            n885 = Index Array(array=w1615, index=w1614) -> (element=→"BPRV":bool)
            n886 = Index Array(array=w1619, index=w1614) -> (element=→"BPFV":bool)
            n887 = Join Numbers(hi=w1627, lo=w1631) -> ((hi.lo)=w1630:u64)
            n888 = Join Numbers(hi=w1627, lo=w1628) -> ((hi.lo)=w1626:u64)
            n889 = Join Numbers(hi=w1606, lo=w1605) -> ((hi.lo)=w1598:u16)
            "BP_front" <- w1598
            n890 = Join Numbers(hi=w1601, lo=w1600) -> ((hi.lo)=w1597:u16)
            "BP_rear" <- w1597
            n891 = Index Array(array=w1641, index #1=w1614, index #2=w1617, index #3=w1618, index #4=w1629) -> (element #1=→"Brake Heartbeat":bool, element #2=→"BPFV":bool, element #3=→"BPFSV":bool, element #4=→"Braking":bool)
            n892 = Join Numbers(hi=w1610, lo=w1632) -> ()  [unwired: 1 out]
            n893 = To Unsigned Byte Integer(number=w1630) -> ()  [unwired: 1 out]
            n894 = Index Array(array=w1599, index=w1618) -> (element=w1624:u8)
            n895 = Bundle(w1598, w1597) -> (→"Front / Rear Brake Pressure":cluster{u16, u16})  [unwired: 1 in]
            n896 = To Unsigned Byte Integer(number=w1626) -> (unsigned 8bit integer=w1625:u8)
            n897 = Join Numbers(hi=w1625, lo=w1624) -> ((hi.lo)=→"Brake Pedal Fore Supply":u16)
          }
          frame 644 {
            # "MCU FL"
            n898 = Index Array(array=w1645, index=5) -> (element=w1676:u8)
            n899 = Index Array(array=w1645, index=4) -> (element=w1675:u8)
            n900 = Index Array(array=w1645, index=7) -> (element=w1661:u8)
            n901 = Index Array(array=w1645, index=6) -> (element=w1660:u8)
            n902 = Index Array(array=w1645, index=9) -> (element=w1667:u8)
            n903 = Index Array(array=w1645, index=8) -> (element=w1666:u8)
            n904 = Index Array(array=w1645, index=3) -> (element=w1644:u8)
            n905 = Join Numbers(hi=w1676, lo=w1675) -> ((hi.lo)=w1665:u16)
            n906 = Join Numbers(hi=w1661, lo=w1660) -> ((hi.lo)=w1653:u16)
            n907 = Join Numbers(hi=w1667, lo=w1666) -> ((hi.lo)=w1651:u16)
            n908 = Number To Boolean Array(number=w1644) -> (Boolean array=→"Status FL":bool[])
            n909 = To Word Integer(number=w1665) -> (16bit integer=→"Actual Velocity\nFL [RPM]":i16)
            n910 = To Word Integer(number=w1653) -> (16bit integer=w1652:i16)
            n911 = To Word Integer(number=w1651) -> (16bit integer=w1650:i16)
            n912 = Multiply(x=w1652, y=105.0) -> (x*y=w1659:dbl)
            n913 = Multiply(x=w1650, y=105.0) -> (x*y=w1654:dbl)
            n914 = Divide(x=w1659, y=16384.0) -> (x/y=w1649:dbl)
            "Id FL [A]" <- w1649
            n915 = Divide(x=w1654, y=16384.0) -> (x/y=w1648:dbl)
            "Iq FL [A]" <- w1648
            n916 = Bundle(w1649, w1648) -> (→"MCU FL":cluster{dbl, dbl})  [unwired: 1 in]
          }
          frame 645 {
            # "MCU FR"
            n917 = Index Array(array=w1679, index=5) -> (element=w1712:u8)
            n918 = Index Array(array=w1679, index=4) -> (element=w1711:u8)
            n919 = Index Array(array=w1679, index=7) -> (element=w1697:u8)
            n920 = Index Array(array=w1679, index=6) -> (element=w1696:u8)
            n921 = Index Array(array=w1679, index=3) -> (element=w1681:u8)
            n922 = Index Array(array=w1679, index=9) -> (element=w1703:u8)
            n923 = Index Array(array=w1679, index=8) -> (element=w1702:u8)
            n924 = Join Numbers(hi=w1712, lo=w1711) -> ((hi.lo)=w1701:u16)
            n925 = Join Numbers(hi=w1697, lo=w1696) -> ((hi.lo)=w1689:u16)
            n926 = Join Numbers(hi=w1703, lo=w1702) -> ((hi.lo)=w1687:u16)
            n927 = Number To Boolean Array(number=w1681) -> (Boolean array=→"Status FR":bool[])
            n928 = To Word Integer(number=w1701) -> (16bit integer=→"Actual Velocity\nFR [RPM]":i16)
            n929 = To Word Integer(number=w1689) -> (16bit integer=w1688:i16)
            n930 = To Word Integer(number=w1687) -> (16bit integer=w1686:i16)
            n931 = Multiply(x=w1688, y=105.0) -> (x*y=w1695:dbl)
            n932 = Multiply(x=w1686, y=105.0) -> (x*y=w1690:dbl)
            n933 = Divide(x=w1695, y=16384.0) -> (x/y=w1685:dbl)
            "Id FR [A]" <- w1685
            n934 = Divide(x=w1690, y=16384.0) -> (x/y=w1684:dbl)
            "Iq FR [A]" <- w1684
            n935 = Bundle(w1685, w1684) -> (→"MCU FR":cluster{dbl, dbl})  [unwired: 1 in]
          }
          frame 646 {
            # "MCU FL"
            n936 = Index Array(array=w1722, index=5) -> (element=w1733:u8)
            n937 = Index Array(array=w1722, index=4) -> (element=w1732:u8)
            n938 = Index Array(array=w1722, index=7) -> (element=w1738:u8)
            n939 = Index Array(array=w1722, index=6) -> (element=w1737:u8)
            n940 = Index Array(array=w1722, index=9) -> (element=w1719:u8)
            n941 = Index Array(array=w1722, index=8) -> (element=w1718:u8)
            n942 = Index Array(array=w1722, index=3) -> (element=w1747:u8)
            n943 = Index Array(array=w1722, index=2) -> (element=w1746:u8)
            n944 = Join Numbers(hi=w1733, lo=w1732) -> ((hi.lo)=w1731:u16)
            n945 = Join Numbers(hi=w1738, lo=w1737) -> ((hi.lo)=w1724:u16)
            n946 = Join Numbers(hi=w1719, lo=w1718) -> ((hi.lo)=w1717:u16)
            n947 = Join Numbers(hi=w1747, lo=w1746) -> ((hi.lo)=w1736:u16)
            n948 = To Word Integer(number=w1731) -> (16bit integer=w1726:i16)
            n949 = To Unsigned Word Integer(number=w1724) -> (unsigned 16bit integer=→"Error Info FL":u16)
            n950 = To Word Integer(number=w1736) -> (16bit integer=w1729:i16)
            n951 = Divide(x=w1717, y=10.0) -> (x/y=→"IGBT FL TEMP":dbl)
            n952 = Divide(x=w1726, y=10.0) -> (x/y=→"T Inv. FL [°C]":dbl)
            n953 = Divide(x=w1729, y=10.0) -> (x/y=→"T Motor FL [°C]":dbl)
          }
          frame 647 {
            # "MCU FR"
            n954 = Index Array(array=w1751, index=5) -> (element=w1768:u8)
            n955 = Index Array(array=w1751, index=4) -> (element=w1767:u8)
            n956 = Index Array(array=w1751, index=7) -> (element=w1773:u8)
            n957 = Index Array(array=w1751, index=6) -> (element=w1772:u8)
            n958 = Index Array(array=w1751, index=9) -> (element=w1755:u8)
            n959 = Index Array(array=w1751, index=8) -> (element=w1754:u8)
            n960 = Index Array(array=w1751, index=3) -> (element=w1782:u8)
            n961 = Index Array(array=w1751, index=2) -> (element=w1781:u8)
            n962 = Join Numbers(hi=w1768, lo=w1767) -> ((hi.lo)=w1766:u16)
            n963 = Join Numbers(hi=w1773, lo=w1772) -> ((hi.lo)=w1759:u16)
            n964 = Join Numbers(hi=w1755, lo=w1754) -> ((hi.lo)=w1753:u16)
            n965 = Join Numbers(hi=w1782, lo=w1781) -> ((hi.lo)=w1771:u16)
            n966 = To Word Integer(number=w1766) -> (16bit integer=w1761:i16)
            n967 = To Unsigned Word Integer(number=w1759) -> (unsigned 16bit integer=→"Error Info FR":u16)
            n968 = To Word Integer(number=w1771) -> (16bit integer=w1764:i16)
            n969 = Divide(x=w1753, y=10.0) -> (x/y=→"IGBT FR TEMP":dbl)
            n970 = Divide(x=w1761, y=10.0) -> (x/y=→"T Inv. FR [°C]":dbl)
            n971 = Divide(x=w1764, y=10.0) -> (x/y=→"T Motor FR [°C]":dbl)
          }
          frame 648 {
            # "MCU RL"
            n972 = Index Array(array=w1785, index=5) -> (element=w1818:u8)
            n973 = Index Array(array=w1785, index=4) -> (element=w1817:u8)
            n974 = Index Array(array=w1785, index=7) -> (element=w1803:u8)
            n975 = Index Array(array=w1785, index=6) -> (element=w1802:u8)
            n976 = Index Array(array=w1785, index=3) -> (element=w1787:u8)
            n977 = Index Array(array=w1785, index=9) -> (element=w1809:u8)
            n978 = Index Array(array=w1785, index=8) -> (element=w1808:u8)
            n979 = Join Numbers(hi=w1818, lo=w1817) -> ((hi.lo)=w1807:u16)
            n980 = Join Numbers(hi=w1803, lo=w1802) -> ((hi.lo)=w1795:u16)
            n981 = Join Numbers(hi=w1809, lo=w1808) -> ((hi.lo)=w1793:u16)
            n982 = Number To Boolean Array(number=w1787) -> (Boolean array=→"Status RL":bool[])
            n983 = To Word Integer(number=w1807) -> (16bit integer=→"Actual Velocity\nRL [RPM]":i16)
            n984 = To Word Integer(number=w1795) -> (16bit integer=w1794:i16)
            n985 = To Word Integer(number=w1793) -> (16bit integer=w1792:i16)
            n986 = Multiply(x=w1794, y=105.0) -> (x*y=w1801:dbl)
            n987 = Multiply(x=w1792, y=105.0) -> (x*y=w1796:dbl)
            n988 = Divide(x=w1801, y=16384.0) -> (x/y=w1790:dbl)
            "Id RL [A]" <- w1790
            n989 = Divide(x=w1796, y=16384.0) -> (x/y=w1789:dbl)
            "Iq RL [A]" <- w1789
            n990 = Bundle(w1790, w1789) -> (→"MCU RL":cluster{dbl, dbl})  [unwired: 1 in]
          }
          frame 649 {
            w1822 = 3.6 ("y")
            # "MCU RR"
            n991 = local read "TCU_v"() -> (w1823:dbl)
            n992 = local read "Id RR [A]"() -> (w1857:dbl)
            n993 = local read "Id FL [A]"() -> (w1860:dbl)
            n994 = local read "Id FR [A]"() -> (w1859:dbl)
            n995 = local read "Id RL [A]"() -> (w1858:dbl)
            n996 = local read "Vel_acc"() -> (w1850:dbl)
            n997 = local read "Vel_acc"() -> (w1841:dbl)
            n998 = flat-sequence {
              frame #0 {
                w1904 = i16 10 ("y")
                w1926 = 15.6 ("y")
                n999 = local read "Torq_sum"() -> (w1924:dbl)
                n1000 = Multiply(x=w1924, y=w1926) -> (x*y=→"Torque [Nm]":dbl)
                n1001 = local read "Actual Velocity \nRR [RPM]"() -> (w1905:i16)
                n1002 = local read "Actual Velocity\nRL [RPM]"() -> (w1906:i16)
                n1003 = local read "Actual Velocity\nFR [RPM]"() -> (w1907:i16)
                n1004 = local read "Actual Velocity\nFL [RPM]"() -> (w1908:i16)
                n1005 = Less?(x=w1906, y=w1904) -> (x < y?=w1910:bool)
                n1006 = Less?(x=w1905, y=w1904) -> (x < y?=w1909:bool)
                n1007 = Less?(x=w1908, y=w1904) -> (x < y?=w1912:bool)
                n1008 = Less?(x=w1907, y=w1904) -> (x < y?=w1911:bool)
                n1009 = To Double Precision Float(number=w1906) -> (double precision float=w1919:dbl)
                n1010 = To Double Precision Float(number=w1905) -> (double precision float=w1918:dbl)
                n1011 = Add(x=w1919, y=w1918) -> (x+y=w1921:dbl)
                n1012 = feedback #27() -> (w1916:dbl)  [unwired: 1 in]
                n1013 = local read "START"() -> (w1902:bool)
                n1014 = Compound Arithmetic op=AND(w1902, w1912, w1911, w1910, w1909) -> (→"IsStopped":bool)
                n1015 = Divide(x=w1921, y=2.0) -> (x/y=w1915:dbl)
                n1016 = formula code="y_=a*x+(1-a)*y;"("x"=w1915, "y"=w1916, "a"=0.1 ("input variable")) -> ("y_"=w1914:dbl)
                n1017 = feedback-in #27(w1914) -> ()
                n1018 = Multiply(x=w1914, y=0.104719755) -> (x*y=w1929:dbl)
                n1019 = Multiply(x=w1929, y=0.227) -> (x*y=w1923:dbl)
                n1020 = Divide(x=w1923, y=w1926) -> (x/y=w1922:dbl)
                n1021 = Multiply(x=w1922, y=3.6) -> (x*y=→"Velocity [km/h]":dbl)
              }
            }
            n1022 = Multiply(x=w1822, y=w1823) -> (x*y=w1821:dbl)
            n1023 = Index Array(array=w1866, index=5) -> (element=w1899:u8)
            n1024 = Index Array(array=w1866, index=4) -> (element=w1898:u8)
            n1025 = Index Array(array=w1866, index=7) -> (element=w1884:u8)
            n1026 = Index Array(array=w1866, index=6) -> (element=w1883:u8)
            n1027 = Index Array(array=w1866, index=3) -> (element=w1868:u8)
            n1028 = Index Array(array=w1866, index=9) -> (element=w1890:u8)
            n1029 = Index Array(array=w1866, index=8) -> (element=w1889:u8)
            n1030 = Divide(x=w1841, y=0.227) -> (x/y=w1839:dbl)
            n1031 = Multiply(x=w1850, y=w1822) -> (x*y=w1851:dbl)
            n1032 = Join Numbers(hi=w1899, lo=w1898) -> ((hi.lo)=w1888:u16)
            n1033 = Join Numbers(hi=w1884, lo=w1883) -> ((hi.lo)=w1876:u16)
            n1034 = Join Numbers(hi=w1890, lo=w1889) -> ((hi.lo)=w1874:u16)
            n1035 = Build Array(w1860, w1859, w1858, w1857) -> (w1856:dbl[])
            n1036 = local read "Velocity [km/h]"() -> (w1853:dbl)
            n1037 = Number To Boolean Array(number=w1868) -> (Boolean array=→"Status RR":bool[])
            n1038 = local read "Actual Velocity \nRR [RPM]"() -> (w1862:i16)
            n1039 = local read "Actual Velocity \nRR [RPM]"() -> (w1849:i16)
            n1040 = local read "Actual Velocity\nFR [RPM]"() -> (w1864:i16)
            n1041 = local read "Actual Velocity\nRL [RPM]"() -> (w1863:i16)
            n1042 = local read "Actual Velocity\nFR [RPM]"() -> (w1847:i16)
            n1043 = local read "Actual Velocity\nRL [RPM]"() -> (w1848:i16)
            n1044 = local read "Actual Velocity\nFL [RPM]"() -> (w1865:i16)
            n1045 = local read "Actual Velocity\nFL [RPM]"() -> (w1846:i16)
            n1046 = To Word Integer(number=w1888) -> (16bit integer=→"Actual Velocity \nRR [RPM]":i16)
            n1047 = To Word Integer(number=w1876) -> (16bit integer=w1875:i16)
            n1048 = To Word Integer(number=w1874) -> (16bit integer=w1873:i16)
            n1049 = call "Curr2Torq.vi"("Current"=w1856) -> ("Torque"=w1855:dbl[])
            n1050 = Bundle("Actual Velocity\nFL [RPM]"=w1865, "Actual Velocity\nFR [RPM]"=w1864, "Actual Velocity\nRL [RPM]"=w1863, "Actual Velocity \nRR [RPM]"=w1862) -> (→"Angular Speed":T17)  [unwired: 1 in]
            n1051 = Add Array Elements(numeric array=w1855) -> (sum=w1854:dbl)
            "Torq_sum" <- w1854
            n1052 = To Double Precision Float(number=w1846) -> (double precision float=w1845:dbl)
            n1053 = To Double Precision Float(number=w1847) -> (double precision float=w1844:dbl)
            n1054 = To Double Precision Float(number=w1848) -> (double precision float=w1843:dbl)
            n1055 = To Double Precision Float(number=w1849) -> (double precision float=w1842:dbl)
            n1056 = Multiply(x=w1875, y=105.0) -> (x*y=w1882:dbl)
            n1057 = Multiply(x=w1873, y=105.0) -> (x*y=w1877:dbl)
            n1058 = Multiply(x=15.6, y=w1839) -> (x*y=w1825:dbl)
            n1059 = Divide(x=w1882, y=16384.0) -> (x/y=w1872:dbl)
            "Id RR [A]" <- w1872
            n1060 = Divide(x=w1877, y=16384.0) -> (x/y=w1871:dbl)
            "Iq RR [A]" <- w1871
            n1061 = Multiply(x=30.0, y=w1825) -> (x*y=w1837:dbl)
            n1062 = Bundle("Velocity [km/h]"=w1853, "Torque"=w1854, w1851, w1821) -> (→"?":T5)  [unwired: 1 in]
            n1063 = Divide(x=w1837, y=3.141592653589793) -> (x/y=w1831:dbl)
            n1064 = Subtract(x=w1845, y=w1831) -> (x-y=w1835:dbl)
            n1065 = Subtract(x=w1844, y=w1831) -> (x-y=w1834:dbl)
            n1066 = Subtract(x=w1843, y=w1831) -> (x-y=w1833:dbl)
            n1067 = Subtract(x=w1842, y=w1831) -> (x-y=w1832:dbl)
            n1068 = Divide(x=w1835, y=w1831) -> (x/y=w1830:dbl)
            n1069 = Divide(x=w1834, y=w1831) -> (x/y=w1829:dbl)
            n1070 = Divide(x=w1833, y=w1831) -> (x/y=w1828:dbl)
            n1071 = Divide(x=w1832, y=w1831) -> (x/y=w1827:dbl)
            n1072 = Bundle(w1872, w1871) -> (→"MCU RR":cluster{dbl, dbl})  [unwired: 1 in]
            n1073 = Bundle(w1830, w1829, w1828, w1827) -> (→"Slip":cluster{dbl, dbl, dbl, dbl})  [unwired: 1 in]
          }
          frame 650 {
            # "MCU RL"
            n1074 = Index Array(array=w1932, index=5) -> (element=w1949:u8)
            n1075 = Index Array(array=w1932, index=4) -> (element=w1948:u8)
            n1076 = Index Array(array=w1932, index=7) -> (element=w1954:u8)
            n1077 = Index Array(array=w1932, index=6) -> (element=w1953:u8)
            n1078 = Index Array(array=w1932, index=9) -> (element=w1936:u8)
            n1079 = Index Array(array=w1932, index=8) -> (element=w1935:u8)
            n1080 = Index Array(array=w1932, index=3) -> (element=w1963:u8)
            n1081 = Index Array(array=w1932, index=2) -> (element=w1962:u8)
            n1082 = Join Numbers(hi=w1949, lo=w1948) -> ((hi.lo)=w1947:u16)
            n1083 = Join Numbers(hi=w1954, lo=w1953) -> ((hi.lo)=w1940:u16)
            n1084 = Join Numbers(hi=w1936, lo=w1935) -> ((hi.lo)=w1934:u16)
            n1085 = Join Numbers(hi=w1963, lo=w1962) -> ((hi.lo)=w1952:u16)
            n1086 = To Word Integer(number=w1947) -> (16bit integer=w1942:i16)
            n1087 = To Unsigned Word Integer(number=w1940) -> (unsigned 16bit integer=→"Error Info RL":u16)
            n1088 = To Word Integer(number=w1952) -> (16bit integer=w1945:i16)
            n1089 = Divide(x=w1934, y=10.0) -> (x/y=→"IGBT RL TEMP":dbl)
            n1090 = Divide(x=w1942, y=10.0) -> (x/y=→"T Inv. RL [°C]":dbl)
            n1091 = Divide(x=w1945, y=10.0) -> (x/y=→"T Motor RL [°C]":dbl)
          }
          frame 651 {
            # "MCU RR"
            n1092 = Index Array(array=w1967, index=5) -> (element=w1984:u8)
            n1093 = Index Array(array=w1967, index=4) -> (element=w1983:u8)
            n1094 = Index Array(array=w1967, index=7) -> (element=w1989:u8)
            n1095 = Index Array(array=w1967, index=6) -> (element=w1988:u8)
            n1096 = Index Array(array=w1967, index=9) -> (element=w1971:u8)
            n1097 = Index Array(array=w1967, index=8) -> (element=w1970:u8)
            n1098 = Index Array(array=w1967, index=3) -> (element=w1998:u8)
            n1099 = Index Array(array=w1967, index=2) -> (element=w1997:u8)
            n1100 = Join Numbers(hi=w1984, lo=w1983) -> ((hi.lo)=w1982:u16)
            n1101 = Join Numbers(hi=w1989, lo=w1988) -> ((hi.lo)=w1975:u16)
            n1102 = Join Numbers(hi=w1971, lo=w1970) -> ((hi.lo)=w1969:u16)
            n1103 = Join Numbers(hi=w1998, lo=w1997) -> ((hi.lo)=w1987:u16)
            n1104 = To Word Integer(number=w1982) -> (16bit integer=w1977:i16)
            n1105 = To Unsigned Word Integer(number=w1975) -> (unsigned 16bit integer=→"Error Info RR":u16)
            n1106 = To Word Integer(number=w1987) -> (16bit integer=w1980:i16)
            n1107 = Divide(x=w1969, y=10.0) -> (x/y=→"IGBT RR TEMP":dbl)
            n1108 = Divide(x=w1977, y=10.0) -> (x/y=→"T Inv. RR [°C]":dbl)
            n1109 = Divide(x=w1980, y=10.0) -> (x/y=→"T Motor RR [°C]":dbl)
          }
          frame 656 {
            n1110 = Index Array(array=w2038, index=5) -> (element=w2031:u8)
            n1111 = Index Array(array=w2038, index=4) -> (element=w2029:u8)
            n1112 = Index Array(array=w2038, index=3) -> (element=w2022:u8)
            n1113 = And(x=w2031, y=u8 15) -> (x .and. y?=→"Dial 5":u8)
            n1114 = And(x=w2022, y=u8 15) -> (x .and. y?=→"Dial":u8)
            n1115 = And(x=w2031, y=u8 240) -> (x .and. y?=w2026:u8)
            n1116 = And(x=w2029, y=u8 240) -> (x .and. y?=w2028:u8)
            n1117 = And(x=w2022, y=u8 240) -> (x .and. y?=w2021:u8)
            n1118 = And(x=w2029, y=u8 15) -> (x .and. y?=w2004:u8)
            "Dial 3" <- w2004
            n1119 = Logical Shift(y=i16 -4, x=w2026) -> (x << y=→"Dial 4":u8)
            n1120 = Logical Shift(y=i16 -4, x=w2021) -> (x << y=w2016:u8)
            n1121 = Logical Shift(y=i16 -4, x=w2028) -> (x << y=w2001:u8)
            "Dial 2" <- w2001
            n1122 = Multiply(x=4.16666, y=w2004) -> (x*y=→"Slope":dbl)
            n1123 = Number To Boolean Array(number=w2016) -> (Boolean array=w2015:bool[])
            n1124 = formula code="if(in1==1) out1=1;\nif(in1==2) out1=0.95;\nif(in1==3) out1=0.9;\nif(in1==4) out1=0.85;\nif(in1==5) out1=0.8;\nif(in1==6) out1=0.75;\nif(in1==7) out1=0.7;\nif(in1==8) out1=0.65;\nif(in1==9) out1=0.6;\nif(in1==10) out1=0.55;\nif(in1==11) out1=0.5;\nif(in1==12) out1=0.4;"("in1"=w2001) -> ()  [unwired: 1 out]
            n1125 = Index Array(array=w2015, index #1=0 ("index"), index #2=1 ("index"), index #3=2 ("index"), index #4=3 ("index")) -> (element #1=→"Boolean":bool, element #2=→"Boolean 2":bool, element #3=→"Boolean 3":bool, element #4=→"Boolean 4":bool)
          }
          frame 657 {
            n1126 = Index Array(array=w2047, index=3) -> (element=w2043:u8)
            n1127 = Index Array(array=w2047, index=2) -> (element=w2044:u8)
            n1128 = Join Numbers(hi=w2044, lo=w2043) -> ((hi.lo)=→"Brake Force 2" →"Brake Force":u16)
          }
          frame 642 {
            n1129 = Index Array(array=w2058, index=3) -> (element=w2102:u8)
            n1130 = Index Array(array=w2058, index #1=4 ("index"), index #2=5 ("index"), index #3=6 ("index"), index #4=7 ("index")) -> (element #1=w2071:u8, element #2=w2067:u8, element #3=w2066:u8, element #4=w2065:u8)
            n1131 = Index Array(array=w2058, index=2) -> (element=w2103:u8)
            n1132 = Number To Boolean Array(number=w2103) -> (Boolean array=w2101:bool[])
            n1133 = Number To Boolean Array(number=w2102) -> (Boolean array=w2084:bool[])
            n1134 = Join Numbers(hi=w2067, lo=w2071) -> ((hi.lo)=w2064:u16)
            n1135 = Join Numbers(hi=w2065, lo=w2066) -> ((hi.lo)=w2063:u16)
            n1136 = Join Numbers(hi=w2063, lo=w2064) -> ((hi.lo)=w2062:u32)
            n1137 = To Long Integer(number=w2062) -> (32bit integer=w2061:i32)
            n1138 = Divide(x=w2061, y=ext 1098.0) -> (x/y=→"Actual pos [°] Maxon":ext)
            n1139 = Index Array(array=w2101, index #1=0 ("index"), index #2=1 ("index"), index #3=2 ("index"), index #4=3 ("index"), index #5=4 ("index"), index #6=5 ("index"), index #7=6 ("index"), index #8=7 ("index")) -> (element #1=→"Ready to switch on":bool, element #2=→"Switched on":bool, element #3=→"Operation enable":bool, element #4=→"Fault present":bool, element #5=→"Voltage enabled":bool, element #7=→"Switch on disabled":bool, element #8=→"Warning present":bool)  [unwired: 1 out]
            n1140 = Index Array(array=w2084, index #1=0 ("index"), index #2=1 ("index"), index #3=2 ("index"), index #4=3 ("index"), index #5=4 ("index"), index #6=5 ("index"), index #7=6 ("index"), index #8=7 ("index")) -> (element #2=→"In operational NMT state":bool, element #3=→"Target reached":bool, element #5=→"Setpoint ack":bool, element #6=→"Following error":bool, element #8=→"Position referenced to home position":bool)  [unwired: 3 out]
          }
          frame 770 {
            n1141 = Index Array(array=w2119, index #1=4 ("index"), index #2=5 ("index"), index #3=6 ("index"), index #4=7 ("index")) -> (element #1=w2131:u8, element #2=w2127:u8, element #3=w2126:u8, element #4=w2125:u8)
            n1142 = Join Numbers(hi=w2127, lo=w2131) -> ((hi.lo)=w2124:u16)
            n1143 = Join Numbers(hi=w2125, lo=w2126) -> ((hi.lo)=w2123:u16)
            n1144 = Join Numbers(hi=w2123, lo=w2124) -> ((hi.lo)=w2122:u32)
            n1145 = To Long Integer(number=w2122) -> (32bit integer=w2120:i32)
            n1146 = Divide(x=w2120, y=ext 1098.0) -> (x/y=w2108:ext)
            n1147 = Equal To 0?(x=w2108) -> (x = 0?=w2110:bool)
            n1148 = local read "Actual pos [°] Maxon"() -> (w2111:ext)
            n1149 = feedback-in #28(w2108) -> ()
            n1150 = feedback #28() -> (w2109:ext)  [unwired: 1 in]
            n1151 = Select(t=w2109, s=w2110, f=w2108) -> (s? t:f=w2107:ext)
            "Target pos [°]" <- w2107
            n1152 = local read "Steering Angle"() -> (w2112:dbl)
            "Actual pos [°]" <- w2112
            n1153 = Bundle(w2107, "Steering Angle"=w2112, "Actual pos [°] Maxon"=w2111) -> (→"Steering Angle":T11)  [unwired: 1 in]
          }
          frame 787 {
            # "HV Critical Cell Values"
            n1154 = Index Array(array=w2136, index=4) -> (element=w2140:u8)
            n1155 = Index Array(array=w2136, index=3) -> (element=w2139:u8)
            n1156 = Index Array(array=w2136, index=5) -> (element=w2135:u8)
            n1157 = Index Array(array=w2136, index=6) -> (element=w2134:u8)
            n1158 = Join Numbers(hi=w2140, lo=w2139) -> ((hi.lo)=w2141:u16)
            n1159 = Join Numbers(hi=w2135, lo=w2134) -> ((hi.lo)=→"Temp Max 2":u16)
            n1160 = To Unsigned Word Integer(number=w2141) -> (unsigned 16bit integer=→"Cell Min 2":u16)
          }
          frame 800 {
            # "MCU Support Status kesz"
            n1161 = Index Array(array=w2155, index=3) -> (element=w2189:u8)
            n1162 = Index Array(array=w2155, index=5) -> (element=w2174:u8)
            n1163 = Index Array(array=w2155, index=6) -> (element=w2153:u8)
            n1164 = Index Array(array=w2155, index=4) -> (element=w2176:u8)
            n1165 = Number To Boolean Array(number=w2189) -> (Boolean array=w2198:bool[])
            n1166 = Number To Boolean Array(number=w2174) -> (Boolean array=w2173:bool[])
            n1167 = To Unsigned Word Integer(number=w2153) -> (unsigned 16bit integer=w2152:u16)
            "MCU S SC Endl" <- w2152
            n1168 = Number To Boolean Array(number=w2176) -> (Boolean array=w2177:bool[])
            n1169 = Greater?(x=w2152, y=5) -> ()  [unwired: 1 out]
            n1170 = Index Array(array=w2198, index #1=7 ("index"), index #2=6 ("index"), index #3=5 ("index"), index #4=4 ("index"), index #5=3 ("index"), index #6=2 ("index"), index #7=1 ("index"), index #8=0 ("index")) -> (element #1=→"Brake Light":bool, element #2=→"MCU EF":bool, element #3=→"MCU RF":bool, element #4=→"RTDS":bool, element #5=→"TCU Power":bool, element #6=→"24V front DC/DC":bool, element #7=→"24V rear DC/DC":bool, element #8=→"LKS & RKS" →"LKS & RKS" →"SC RKS" →"SC LKS":bool)
            n1171 = Index Array(array=w2177, index #1=7 ("index"), index #2=6 ("index"), index #3=5 ("index"), index #4=4 ("index"), index #5=3 ("index"), index #6=2 ("index"), index #7=1 ("index"), index #8=0 ("index")) -> (element #1=→"MCU Interlocks" →"MCU Interlock" →"SC Motor 4" →"SC Motor 1" →"SC Motor 3" →"SC MCU" →"SC Motor 2" →"Motor1 Interlock" →"Motor2 Interlock" →"Motor3 Interlock" →"Motor4 Interlock" →"HVD Interlock":bool, element #2=→"ON" →"ON":bool, element #3=→"START" →"START":bool, element #4=→"OFF" →"OFF":bool, element #5=→"Logging":bool, element #6=→"XBee CS":bool, element #7=→"Radio CS":bool, element #8=→"SD CS":bool)
            n1172 = Index Array(array=w2173, index=7) -> (element=→"TSAL":bool)
          }
          frame 816 {
            # "5db 12V"
            # "3db 48V"
            # "LV Sys Status"
            n1173 = Index Array(array=w2223, index=7) -> (element=w2251:u8)
            n1174 = Index Array(array=w2223, index=6) -> (element=w2291:u8)
            n1175 = Index Array(array=w2223, index=3) -> (element=w2308:u8)
            n1176 = Index Array(array=w2223, index=8) -> (element=w2221:u8)
            n1177 = Index Array(array=w2223, index=4) -> (element=w2265:u8)
            n1178 = Index Array(array=w2223, index=5) -> (element=w2262:u8)
            n1179 = Logical Shift(y=i16 -4, x=w2262) -> (x << y=w2280:u8)
            n1180 = Number To Boolean Array(number=w2251) -> (Boolean array=w2250:bool[])
            n1181 = Number To Boolean Array(number=w2291) -> (Boolean array=w2290:bool[])
            n1182 = Number To Boolean Array(number=w2308) -> (Boolean array=w2307:bool[])
            n1183 = Number To Boolean Array(number=w2221) -> (Boolean array=w2220:bool[])
            n1184 = Number To Boolean Array(number=w2265) -> (Boolean array=w2298:bool[])
            n1185 = Number To Boolean Array(number=w2262) -> (Boolean array=w2261:bool[])
            n1186 = Index Array(array=w2261, index #1=3, index #2=2, index #3=1, index #4=0) -> (element #1=→"Battery Full" →"Battery Full 2":bool, element #2=→"Overtemp. 3" →"Overtemp. 4":bool, element #3=→"Undervoltage 3" →"Undervoltage 4":bool, element #4=→"Battery Low" →"Battery Low 2":bool)
            n1187 = Index Array(array=w2298, index #1=7 ("index"), index #2=6 ("index"), index #3=5 ("index"), index #4=4 ("index"), index #5=3 ("index")) -> (element #1=→"48V Out 1" →"48V Out 1 2":bool, element #2=→"48V Out 2" →"48V Out 2 2":bool, element #3=→"48V Out 3" →"48V Out 3 2":bool, element #4=→"48V Out 4" →"48V Out 4 2":bool)  [unwired: 3 in, 4 out]
            n1188 = Index Array(array=w2250, index #1=7 ("index"), index #2=6 ("index"), index #3=5 ("index"), index #4=4 ("index"), index #5=3 ("index"), index #6=2 ("index"), index #7=1 ("index"), index #8=0 ("index")) -> (element #1=w2231:bool, element #2=w2230:bool, element #3=w2229:bool, element #4=w2226:bool, element #5=w2228:bool, element #6=w2225:bool, element #7=w2227:bool, element #8=w2224:bool)
            n1189 = Index Array(array=w2290, index #1=7 ("index"), index #2=6 ("index"), index #3=5 ("index"), index #4=4 ("index"), index #5=3 ("index"), index #6=2 ("index"), index #7=1 ("index"), index #8=0 ("index")) -> (element #1=w2239:bool, element #2=w2235:bool, element #3=w2238:bool, element #4=w2234:bool, element #5=w2237:bool, element #6=w2233:bool, element #7=w2236:bool, element #8=w2232:bool)
            n1190 = Index Array(array=w2220, index #1=7 ("index"), index #2=6 ("index"), index #3=5 ("index"), index #4=4 ("index"), index #5=3 ("index"), index #6=2 ("index"), index #7=1 ("index"), index #8=0 ("index")) -> (element #1=w2211:bool, element #2=w2210:bool, element #3=→"BMS IC Wake" →"BMS IC Awake":bool, element #4=→"BMS IC Fault" →"BMS IC Error":bool, element #5=→"Radio CS" →"Radio CS":bool, element #6=→"Logging Status" →"Logging Status" →"Logging":bool, element #7=→"Overvoltage":bool)  [unwired: 1 out]
            n1191 = And(x=w2280, y=u8 15) -> (x .and. y?=→"Undervoltage Errrors":u8)
            n1192 = Index Array(array=w2307, index #1=7 ("index"), index #2=6 ("index"), index #3=5 ("index"), index #4=4 ("index"), index #5=3 ("index"), index #6=2 ("index"), index #7=1 ("index"), index #8=0 ("index")) -> (element #1=→"Main Switch" →"Main Switch 2":bool, element #2=→"MP Switch" →"MP Switch 2":bool, element #3=→"SC BOTS &\nINS & CKS" →"SC State" →"SC State 2":bool, element #4=→"12V Out 1" →"12V Out 1 2":bool, element #5=→"12V Out 2" →"12V Out 2 2" →"Radiator Cooling":bool, element #6=→"12V Out 3" →"12V Out 3 2":bool, element #7=→"12V Out 4" →"12V Out 4 2":bool, element #8=→"12V Out 5" →"12V Out 5 2":bool)
            n1193 = And(x=w2265, y=15) -> (x .and. y?=→"Overtemp Errors":i32)
            n1194 = Build Array(w2211, w2227, w2228, w2229, w2231, w2239, w2238, w2237, w2236) -> (→"Status LEDs Green":bool[])
            n1195 = Build Array(w2210, w2224, w2225, w2226, w2230, w2235, w2234, w2233, w2232) -> (→"Status LEDs Red":bool[])
          }
          frame 817 {
            # "Offset error"
            # "PDM Status"
            n1196 = Index Array(array=w2329, index=2) -> (element=w2341:u8)
            n1197 = Index Array(array=w2329, index=3) -> (element=w2342:u8)
            n1198 = Index Array(array=w2329, index=4) -> (element=w2349:u8)
            n1199 = Index Array(array=w2329, index=5) -> (element=w2350:u8)
            n1200 = Index Array(array=w2329, index=6) -> (element=w2345:u8)
            n1201 = Index Array(array=w2329, index=7) -> (element=w2346:u8)
            n1202 = Join Numbers(hi=w2341, lo=w2342) -> ((hi.lo)=w2319:u16)
            n1203 = Join Numbers(hi=w2349, lo=w2350) -> ((hi.lo)=w2326:u16)
            n1204 = Join Numbers(hi=w2345, lo=w2346) -> ((hi.lo)=w2318:u16)
            n1205 = To Unsigned Word Integer(number=w2319) -> (unsigned 16bit integer=w2320:u16)
            n1206 = To Word Integer(number=w2326) -> (16bit integer=w2325:i16)
            n1207 = To Unsigned Word Integer(number=w2318) -> (unsigned 16bit integer=w2317:u16)
            n1208 = feedback #29() -> (w2328:dbl)  [unwired: 1 in]
            n1209 = feedback #30() -> (w2338:dbl)  [unwired: 1 in]
            n1210 = To Double Precision Float(number=w2320) -> (double precision float=w2327:dbl)
            n1211 = feedback #31() -> (w2340:dbl)  [unwired: 1 in]
            n1212 = To Double Precision Float(number=w2325) -> (double precision float=w2324:dbl)
            n1213 = To Double Precision Float(number=w2317) -> (double precision float=w2336:dbl)
            n1214 = formula code="y_=a*x+(1-a)*y;"("x"=w2327, "y"=w2328, "a"=0.1 ("input variable")) -> ("y_"=w2321:dbl)
            n1215 = feedback-in #29(w2321) -> ()
            n1216 = formula code="y_=a*x+(1-a)*y;"("x"=w2324, "y"=w2340, "a"=0.1 ("input variable")) -> ("y_"=w2316:dbl)
            "48V Current [mA]" <- w2316
            n1217 = feedback-in #31(w2316) -> ()
            n1218 = formula code="y_=a*x+(1-a)*y;"("x"=w2336, "y"=w2338, "a"=0.1 ("input variable")) -> ("y_"=w2315:dbl)
            "12V Current [mA]" <- w2315
            n1219 = feedback-in #30(w2315) -> ()
            n1220 = Divide(x=w2321, y=1000.0) -> (x/y=→"LV Voltage [V]":dbl)
            n1221 = Divide(x=w2316, y=1000.0) -> (x/y=→"48V Current [A]":dbl)
            n1222 = Bundle("y_"=w2316, "y_"=w2315) -> (→"LV Current":cluster{"y_":dbl, "y_":dbl})  [unwired: 1 in]
            n1223 = Divide(x=w2315, y=1000.0) -> (x/y=→"12V Current [A]":dbl)
          }
          frame 832 {
            # "MCU Power ECU Status"
            n1224 = Index Array(array=w2364, index=3) -> (element=w2416:u8)
            n1225 = Index Array(array=w2364, index=5) -> (element=w2386:u8)
            n1226 = Index Array(array=w2364, index=6) -> (element=w2363:u8)
            n1227 = Index Array(array=w2364, index=7) -> (element=w2362:u8)
            n1228 = Index Array(array=w2364, index=4) -> (element=w2405:u8)
            n1229 = Index Array(array=w2364, index=8) -> (element=w2361:u8)
            n1230 = Index Array(array=w2364, index=9) -> (element=w2360:u8)
            n1231 = Join Numbers(hi=w2363, lo=w2362) -> ((hi.lo)=→"Power A Current":u16)
            n1232 = Join Numbers(hi=w2361, lo=w2360) -> ((hi.lo)=→"Power B Current":u16)
            n1233 = Number To Boolean Array(number=w2416) -> (Boolean array=w2415:bool[])
            n1234 = Number To Boolean Array(number=w2386) -> (Boolean array=w2385:bool[])
            n1235 = Number To Boolean Array(number=w2405) -> (Boolean array=w2404:bool[])
            n1236 = Index Array(array=w2415, index #1=7 ("index"), index #2=6 ("index"), index #3=5 ("index"), index #4=4 ("index"), index #5=3 ("index"), index #6=2 ("index"), index #7=1 ("index")) -> (element #7=→"24V Power B":bool)  [unwired: 6 out]
            n1237 = Index Array(array=w2385, index #1=7 ("index"), index #2=6 ("index"), index #3=5 ("index"), index #4=4 ("index"), index #5=3 ("index"), index #6=2 ("index"), index #7=1 ("index"), index #8=0 ("index")) -> (element #2=→"MCU FL 2":bool, element #3=→"MCU FL 3":bool, element #4=→"MCU FL 4":bool, element #5=→"MCU SC Endline" →"MCU SC Endline 2":bool, element #6=→"MCU TSAL":bool, element #7=→"CAN1 Term.":bool, element #8=→"CAN2 Term.":bool)  [unwired: 1 out]
            n1238 = Index Array(array=w2404, index #1=7 ("index"), index #2=6 ("index"), index #3=5 ("index"), index #4=4 ("index"), index #5=3 ("index"), index #6=2 ("index"), index #7=1 ("index"), index #8=0 ("index")) -> (element #1=→"MCU EF A":bool, element #2=→"MCU EF B":bool, element #3=→"MCU EF2 A":bool, element #4=→"MCU EF2 B":bool, element #5=→"MCU RF 1":bool, element #6=→"MCU RF 2":bool, element #7=→"MCU RF 3":bool, element #8=→"MCU RF 4":bool)
          }
          frame 896 {
            # "TCU Status"
            n1239 = call "read_TCUStatus1.vi"("Message"=w2442) -> ("Status1"=w2441:T18)  [unwired: 10 in]
            n1240 = Unbundle By Name(w2441) -> ("Regen %"=→"Regen %":u8, "Characteristics"=→"Characteristics Approx":u8, "Drop Parameter"=→"Drop":dbl, "Yaw Control P"=→"P tag":u16, "Max Power"=→"Max Power":u8, "Torque %"=→"Torque %":u8, "Max RPM"=→"Max RPM":u16, "Regen press"=→"Pressure based":bool, "Regen force"=→"Force based":bool, "BTC"=→"BTC":bool, "Safety Mode"=→"Safety Mode Enabled":bool, "Hardcore Powerlimiter On"=→"Hardcore Powlim":bool, "Throttle Powerlimiter On"=→"Throttle Based Powlim":bool, "Torque Powerlimiter On"=→"Torque Based Powlim":bool, "New Drop Enabled"=→"New Drop":bool, "Yaw Control On"=→"Yaw_Control_ON":bool, "Traction Control On"=→"Traction Control ON":bool, "Slip Control On"=→"SlipControl_Enabled":bool, "Launch Control On"=→"LaunchControl_Active":bool)  [unwired: 1 out]
          }
          frame 897 {
            w2460 = 0.6 ("x")
            w2461 = 0.6 ("y")
            # "Acceleration X & Roll"
            n1241 = local read "Acc Z offset"() -> (w2479:dbl)
            n1242 = local read "Acc Y offset"() -> (w2448:dbl)
            n1243 = local read "AccelYRaw"() -> (w2521:dbl)
            n1244 = local read "AccelXRaw"() -> (w2525:dbl)
            n1245 = local read "AccelXRaw"() -> (w2450:dbl)
            n1246 = local read "Acc X 2"() -> (w2477:dbl)
            n1247 = local read "Acc Y 2"() -> (w2467:dbl)
            n1248 = Add(x=w2461, y=w2460) -> (x+y=w2462:dbl)
            n1249 = Index Array(array=w2506, index=5) -> (element=w2515:u8)
            n1250 = Index Array(array=w2506, index=2) -> (element=w2518:u8)
            n1251 = Index Array(array=w2506, index=3) -> (element=w2517:u8)
            n1252 = Index Array(array=w2506, index=6) -> (element=w2513:u8)
            n1253 = Index Array(array=w2506, index=7) -> (element=w2511:u8)
            n1254 = Index Array(array=w2506, index=8) -> (element=w2509:u8)
            n1255 = Index Array(array=w2506, index=9) -> (element=w2507:u8)
            n1256 = Index Array(array=w2506, index=4) -> (element=w2516:u8)
            n1257 = Subtract(x=w2467, y=w2448) -> (x-y=w2469:dbl)
            n1258 = feedback #32() -> (w2523:dbl)  [unwired: 1 in]
            n1259 = formula code="y_=a*x+(1-a)*y;"("x"=w2521, "y"=w2523, "a"=0.1 ("input variable")) -> ("y_"=w2520:dbl)
            n1260 = feedback-in #32(w2520) -> ()
            n1261 = feedback #33() -> (w2540:dbl[])  [unwired: 1 in]
            n1262 = feedback #34() -> (w2526:dbl)  [unwired: 1 in]
            n1263 = formula code="y_=a*x+(1-a)*y;"("x"=w2525, "y"=w2526, "a"=0.1 ("input variable")) -> ("y_"=w2519:dbl)
            n1264 = feedback-in #34(w2519) -> ()
            n1265 = feedback #35() -> (w2533:dbl[])  [unwired: 1 in]
            n1266 = To Byte Integer(number=w2515) -> (8bit integer=w2498:i8)
            n1267 = To Double Precision Float(number=w2518) -> (double precision float=w2545:dbl)
            n1268 = To Byte Integer(number=w2517) -> (8bit integer=w2503:i8)
            n1269 = To Byte Integer(number=w2513) -> (8bit integer=w2489:i8)
            n1270 = To Byte Integer(number=w2511) -> (8bit integer=w2488:i8)
            n1271 = To Byte Integer(number=w2509) -> (8bit integer=w2487:i8)
            n1272 = To Byte Integer(number=w2507) -> (8bit integer=w2486:i8)
            n1273 = To Byte Integer(number=w2516) -> (8bit integer=w2502:i8)
            n1274 = local read "Acc X offset 2"() -> (w2478:dbl)
            n1275 = local read "Acc Z"() -> (w2480:dbl)
            n1276 = local read "Acc Y"() -> (w2466:dbl)
            n1277 = Subtract(x=w2480, y=w2479) -> (x-y=w2476:dbl)
            n1278 = Subtract(x=w2477, y=w2478) -> (x-y=w2475:dbl)
            n1279 = Subtract(x=w2466, y=w2448) -> (x-y=w2468:dbl)
            n1280 = Multiply(x=w2460, y=w2469) -> (x*y=w2464:dbl)
            n1281 = To Double Precision Float(number=w2498) -> (double precision float=w2499:dbl)
            n1282 = To Double Precision Float(number=w2503) -> (double precision float=w2504:dbl)
            n1283 = To Double Precision Float(number=w2489) -> (double precision float=w2497:dbl)
            n1284 = To Double Precision Float(number=w2488) -> (double precision float=w2494:dbl)
            n1285 = To Double Precision Float(number=w2487) -> (double precision float=w2493:dbl)
            n1286 = To Double Precision Float(number=w2486) -> (double precision float=w2490:dbl)
            n1287 = To Double Precision Float(number=w2502) -> (double precision float=w2544:dbl)
            n1288 = Divide(x=w2545, y=2.0) -> (x/y=→"TCU_v":dbl)
            n1289 = Multiply(x=w2468, y=w2461) -> (x*y=w2465:dbl)
            n1290 = Build Array (concatenate)(w2533, w2519) -> (w2534:dbl[])
            n1291 = Negate(x=w2476) -> (-x=w2454:dbl)
            n1292 = Build Array (concatenate)(w2540, w2520) -> (w2538:dbl[])
            n1293 = Divide(x=w2499, y=20.0) -> (x/y=→"TCU_yaw":dbl)
            n1294 = Divide(x=w2544, y=50.0) -> (x/y=→"TCU_ay":dbl)
            n1295 = Build Array(w2520) -> (w2531:dbl[])
            n1296 = Build Array(w2519) -> (w2530:dbl[])
            n1297 = Divide(x=w2504, y=50.0) -> (x/y=w2451:dbl)
            "TCU_ax" <- w2451
            n1298 = Divide(x=w2497, y=127.0) -> (x/y=w2485:dbl)
            "TCU_slipFL" <- w2485
            n1299 = Divide(x=w2494, y=127.0) -> (x/y=w2484:dbl)
            "TCU_slipFR" <- w2484
            n1300 = Divide(x=w2493, y=127.0) -> (x/y=w2483:dbl)
            "TCU_slipRL" <- w2483
            n1301 = Divide(x=w2490, y=127.0) -> (x/y=w2482:dbl)
            "TCU_slipRR" <- w2482
            n1302 = Add(x=w2454, y=w2475) -> (x+y=w2474:dbl)
            n1303 = Add(x=w2465, y=w2464) -> (x+y=w2463:dbl)
            n1304 = Array Size(array=w2538) -> (size(s)=w2537:i32)
            n1305 = Bundle(w2531, w2530) -> (w2527:cluster{dbl[], dbl[]})  [unwired: 1 in]
            n1306 = Bundle(w2485, w2484, w2483, w2482) -> (→"Slip_TCU":cluster{dbl, dbl, dbl, dbl})  [unwired: 1 in]
            n1307 = Negate(x=w2474) -> (-x=w2473:dbl)
            n1308 = Negate(x=w2463) -> (-x=w2470:dbl)
            n1309 = Subtract(x=w2451, y=w2450) -> (x-y=w2449:dbl)
            "Numeric" <- w2449
            n1310 = Less?(x=w2537, y=1000) -> (x < y?=w2535:bool)
            n1311 = Divide(x=w2470, y=w2462) -> (x/y=w2459:dbl)
            n1312 = Divide(x=w2473, y=2.0) -> (x/y=w2471:dbl)
            n1313 = case shown="True" w2535 {
              tunnel: [w2555 w2564] -> w2532
              tunnel: w2534 -> [w2556 w2564]
              tunnel: [w2559 w2563] -> w2539
              tunnel: w2538 -> [w2562 w2563]
              frame False {
                n1314 = Delete From Array(array=w2562, length=1, index=0) -> (array with subset deleted=w2559:dbl[])  [unwired: 1 out]
                n1315 = Delete From Array(array=w2556, length=1, index=0) -> (array with subset deleted=w2555:dbl[])  [unwired: 1 out]
              }
              frame True {
              }
            }
            n1316 = feedback-in #33(w2539) -> ()
            n1317 = feedback-in #35(w2532) -> ()
            n1318 = Bundle(w2451, "AccelXRaw"=w2450, w2449) -> (→"TCU speed":cluster{dbl, "AccelXRaw":dbl, dbl})  [unwired: 1 in]
            n1319 = Multiply(x=9.81, y=w2471) -> (x*y=→"AccelXRaw":dbl)
            n1320 = Multiply(x=w2459, y=9.81) -> (x*y=→"AccelYRaw":dbl)
            n1321 = Bundle(w2539, w2532) -> (w2528:cluster{dbl[], dbl[]})  [unwired: 1 in]
            n1322 = Build Array(w2527, w2528) -> (→"TCU_acc":cluster{dbl[], dbl[]}[])
          }
          frame 1029 {
            # "Throttle EEPROM"
            n1323 = Index Array(array=w2569, index=2) -> (element=w2581:u8)
            n1324 = Index Array(array=w2569, index=3) -> (element=w2580:u8)
            n1325 = Index Array(array=w2569, index=4) -> (element=w2579:u8)
            n1326 = Index Array(array=w2569, index=5) -> (element=w2578:u8)
            n1327 = Index Array(array=w2569, index=6) -> (element=w2573:u8)
            n1328 = Index Array(array=w2569, index=7) -> (element=w2572:u8)
            n1329 = Index Array(array=w2569, index=8) -> (element=w2571:u8)
            n1330 = Index Array(array=w2569, index=9) -> (element=w2570:u8)
            n1331 = Join Numbers(hi=w2581, lo=w2580) -> ((hi.lo)=→"APPS1 ADC Min":u16)
            n1332 = Join Numbers(hi=w2579, lo=w2578) -> ((hi.lo)=→"APPS1 ADC Max":u16)
            n1333 = Join Numbers(hi=w2573, lo=w2572) -> ((hi.lo)=→"APPS2 ADC Min":u16)
            n1334 = Join Numbers(hi=w2571, lo=w2570) -> ((hi.lo)=→"APPS2 ADC Max":u16)
          }
          frame 1030 {
            # "Steering EEPROM"
            n1335 = Index Array(array=w2593, index=2) -> (element=w2600:u8)
            n1336 = Index Array(array=w2593, index=3) -> (element=w2599:u8)
            n1337 = Index Array(array=w2593, index=6) -> (element=w2596:u8)
            n1338 = Index Array(array=w2593, index=7) -> (element=w2595:u8)
            n1339 = Join Numbers(hi=w2600, lo=w2599) -> ((hi.lo)=→"STA1 ADC 90":u16)
            n1340 = Join Numbers(hi=w2596, lo=w2595) -> ((hi.lo)=→"STA2 ADC 90":u16)
          }
          frame 1031 {
            # "Brake EEPROM"
            n1341 = Index Array(array=w2611, index=2) -> (element=w2628:u8)
            n1342 = Index Array(array=w2611, index=3) -> (element=w2627:u8)
            n1343 = Index Array(array=w2611, index=4) -> (element=w2626:u8)
            n1344 = Index Array(array=w2611, index=5) -> (element=w2625:u8)
            n1345 = Index Array(array=w2611, index=6) -> (element=w2620:u8)
            n1346 = Index Array(array=w2611, index=7) -> (element=w2619:u8)
            n1347 = Index Array(array=w2611, index=8) -> (element=w2618:u8)
            n1348 = Index Array(array=w2611, index=9) -> (element=w2617:u8)
            n1349 = Join Numbers(hi=w2628, lo=w2627) -> ((hi.lo)=→"BSE1 ADC Min":u16)
            n1350 = Join Numbers(hi=w2626, lo=w2625) -> ((hi.lo)=→"BSE1 ADC Max":u16)
            n1351 = Join Numbers(hi=w2620, lo=w2619) -> ((hi.lo)=→"BSE2 ADC Max":u16)
            n1352 = Join Numbers(hi=w2618, lo=w2617) -> ((hi.lo)=→"BSE2 ADC Min":u16)
          }
          frame 1032 {
            # "Steering Middle EEPROM"
            n1353 = Index Array(array=w2635, index=2) -> (element=w2644:u8)
            n1354 = Index Array(array=w2635, index=3) -> (element=w2643:u8)
            n1355 = Index Array(array=w2635, index=4) -> (element=w2642:u8)
            n1356 = Index Array(array=w2635, index=5) -> (element=w2641:u8)
            n1357 = Join Numbers(hi=w2644, lo=w2643) -> ((hi.lo)=→"STA1 ADC Null":u16)
            n1358 = Join Numbers(hi=w2642, lo=w2641) -> ((hi.lo)=→"STA2 ADC Null":u16)
          }
          frame 1057 {
            w2672 = 0.1 ("input variable")
            # "Right in and out are permuted"
            # "Left in and out are permuted"
            # "Left in and out are permuted"
            # "Right in and out are permuted"
            n1359 = Index Array(array=w2690, index=4) -> (element=w2697:u8)
            n1360 = Index Array(array=w2690, index=5) -> (element=w2698:u8)
            n1361 = Index Array(array=w2690, index=2) -> (element=w2700:u8)
            n1362 = Index Array(array=w2690, index=3) -> (element=w2699:u8)
            n1363 = Index Array(array=w2690, index=8) -> (element=w2687:u8)
            n1364 = Index Array(array=w2690, index=9) -> (element=w2686:u8)
            n1365 = Index Array(array=w2690, index=6) -> (element=w2692:u8)
            n1366 = Index Array(array=w2690, index=7) -> (element=w2691:u8)
            n1367 = Join Numbers(hi=w2697, lo=w2698) -> ((hi.lo)=w2682:u16)
            n1368 = Join Numbers(hi=w2700, lo=w2699) -> ((hi.lo)=w2685:u16)
            n1369 = Join Numbers(hi=w2687, lo=w2686) -> ((hi.lo)=w2679:u16)
            n1370 = Join Numbers(hi=w2692, lo=w2691) -> ((hi.lo)=w2678:u16)
            n1371 = feedback #36() -> (w2675:dbl)  [unwired: 1 in]
            n1372 = feedback #37() -> (w2676:dbl)  [unwired: 1 in]
            n1373 = feedback #38() -> (w2673:dbl)  [unwired: 1 in]
            n1374 = feedback #39() -> (w2674:dbl)  [unwired: 1 in]
            n1375 = local read "T Motor RR [°C]"() -> (w2667:dbl)
            n1376 = local read "T Motor FR [°C]"() -> (w2669:dbl)
            n1377 = local read "T Motor RL [°C]"() -> (w2668:dbl)
            n1378 = local read "T Motor FL [°C]"() -> (w2670:dbl)
            n1379 = local read "IGBT RR TEMP"() -> (w2650:dbl)
            n1380 = local read "IGBT FL TEMP"() -> (w2653:i16)
            n1381 = local read "IGBT FR TEMP"() -> (w2652:dbl)
            n1382 = local read "IGBT RL TEMP"() -> (w2651:dbl)
            n1383 = local read "T Inv. RR [°C]"() -> (w2666:dbl)
            n1384 = local read "T Inv. FR [°C]"() -> (w2664:dbl)
            n1385 = local read "T Inv. RL [°C]"() -> (w2665:dbl)
            n1386 = local read "T Inv. FL [°C]"() -> (w2663:dbl)
            n1387 = Bundle("IGBT FL TEMP"=w2653, "IGBT FR TEMP"=w2652, "IGBT RL TEMP"=w2651, "IGBT RR TEMP"=w2650) -> (→"IGBT Temperature":T2)  [unwired: 1 in]
            n1388 = Bundle("T Motor FL [°C]"=w2670, "T Motor FR [°C]"=w2669, "T Motor RL [°C]"=w2668, "T Motor RR [°C]"=w2667) -> (→"Motor Temperature":T19)  [unwired: 1 in]
            n1389 = Bundle("T Inv. FL [°C]"=w2663, "T Inv. FR [°C]"=w2664, "T Inv. RL [°C]"=w2665, "T Inv. RR [°C]"=w2666) -> (→"Inverter Temperature":T20)  [unwired: 1 in]
            n1390 = Divide(x=w2682, y=10.0) -> (x/y=w2656:dbl)
            "Radiator Left IN" <- w2656
            n1391 = Divide(x=w2685, y=10.0) -> (x/y=w2657:dbl)
            "Radiator Left OUT" <- w2657
            n1392 = Divide(x=w2679, y=10.0) -> (x/y=w2654:dbl)
            "Radiator Right IN" <- w2654
            n1393 = Divide(x=w2678, y=10.0) -> (x/y=w2655:dbl)
            "Radiator Right OUT" <- w2655
            n1394 = formula code="y_=a*x+(1-a)*y;"("x"=w2657, "y"=w2676, "a"=w2672) -> ("y_"=w2661:dbl)
            n1395 = feedback-in #37(w2661) -> ()
            n1396 = formula code="y_=a*x+(1-a)*y;"("x"=w2656, "y"=w2675, "a"=w2672) -> ("y_"=w2660:dbl)
            n1397 = feedback-in #36(w2660) -> ()
            n1398 = formula code="y_=a*x+(1-a)*y;"("x"=w2654, "y"=w2673, "a"=w2672) -> ("y_"=w2658:dbl)
            n1399 = feedback-in #38(w2658) -> ()
            n1400 = formula code="y_=a*x+(1-a)*y;"("x"=w2655, "y"=w2674, "a"=w2672) -> ("y_"=w2659:dbl)
            n1401 = feedback-in #39(w2659) -> ()
            n1402 = Bundle("y_"=w2660, "y_"=w2661, "y_"=w2658, "y_"=w2659) -> (→"Radiator Temperature":cluster{"y_":dbl, "y_":dbl, "y_":dbl, "y_":dbl})  [unwired: 1 in]
          }
          frame 1058 {
            w2741 = 0.1 ("input variable")
            n1403 = Index Array(array=w2746, index=2) -> (element=w2752:u8)
            n1404 = Index Array(array=w2746, index=3) -> (element=w2751:u8)
            n1405 = Index Array(array=w2746, index=4) -> (element=w2749:u8)
            n1406 = Index Array(array=w2746, index=5) -> (element=w2750:u8)
            n1407 = feedback #40() -> (w2742:dbl)  [unwired: 1 in]
            n1408 = feedback #41() -> (w2744:dbl)  [unwired: 1 in]
            n1409 = feedback #42() -> (w2745:dbl)  [unwired: 1 in]
            n1410 = feedback #43() -> (w2743:dbl)  [unwired: 1 in]
            n1411 = local read "Wheel Travel FR"() -> (w2713:u16)
            n1412 = local read "Wheel Travel FL"() -> (w2709:u16)
            n1413 = Join Numbers(hi=w2752, lo=w2751) -> ((hi.lo)=w2735:u16)
            "Wheel Travel RL" <- w2735
            n1414 = Join Numbers(hi=w2749, lo=w2750) -> ((hi.lo)=w2708:u16)
            "Wheel Travel RR" <- w2708
            n1415 = Subtract(x=w2709, y="Wheel Travel FL Offset") -> (x-y=w2722:dbl)
            n1416 = Subtract(x=w2735, y="Wheel Travel RL Offset") -> (x-y=w2733:dbl)
            n1417 = Subtract(x=w2708, y="Wheel Travel RR Offset") -> (x-y=w2727:dbl)
            n1418 = Subtract(x=w2713, y="Wheel Travel FR") -> (x-y=w2717:dbl)
            n1419 = formula code="y_=a*x+(1-a)*y;"("x"=w2713, "y"=w2742, "a"=w2741) -> ("y_"=w2739:dbl)
            n1420 = feedback-in #40(w2739) -> ()
            n1421 = formula code="y_=a*x+(1-a)*y;"("x"=w2735, "y"=w2745, "a"=w2741) -> ("y_"=w2738:dbl)
            n1422 = feedback-in #42(w2738) -> ()
            n1423 = formula code="y_=a*x+(1-a)*y;"("x"=w2709, "y"=w2743, "a"=w2741) -> ("y_"=w2740:dbl)
            n1424 = feedback-in #43(w2740) -> ()
            n1425 = formula code="y_=a*x+(1-a)*y;"("x"=w2708, "y"=w2744, "a"=w2741) -> ("y_"=w2737:dbl)
            n1426 = feedback-in #41(w2737) -> ()
            n1427 = Bundle("y_"=w2740, "y_"=w2739, "y_"=w2738, "y_"=w2737) -> (→"Wheel Travel":cluster{"y_":dbl, "y_":dbl, "y_":dbl, "y_":dbl})  [unwired: 1 in]
            n1428 = Multiply(x=w2722, y=75.0) -> (x*y=w2720:dbl)
            n1429 = Multiply(x=w2733, y=75.0) -> (x*y=w2731:dbl)
            n1430 = Multiply(x=w2727, y=75.0) -> (x*y=w2725:dbl)
            n1431 = Multiply(x=w2717, y=75.0) -> (x*y=w2715:dbl)
            n1432 = Divide(x=w2720, y=4095.0) -> (x/y=→"Damper Travel FL [mm]":dbl)
            n1433 = Divide(x=w2731, y=4095.0) -> (x/y=→"Damper Travel RL [mm]":dbl)
            n1434 = Divide(x=w2725, y=4095.0) -> (x/y=→"Damper Travel RR [mm]":dbl)
            n1435 = Divide(x=w2715, y=4095.0) -> (x/y=→"Damper Travel FR [mm]":dbl)
          }
          frame 1074 {
            w2781 = u8 127 ("y")
            # "PDM LV Cell Values"
            n1436 = Index Array(array=w2760, index=5) -> (element=w2786:u8)
            n1437 = Index Array(array=w2760, index=6) -> (element=w2785:u8)
            n1438 = Index Array(array=w2760, index=2) -> (element=w2790:u8)
            n1439 = Index Array(array=w2760, index=3) -> (element=w2782:u8)
            n1440 = Index Array(array=w2760, index=4) -> (element=w2791:u8)
            n1441 = Join Numbers(hi=w2786, lo=w2785) -> ((hi.lo)=w2784:u16)
            n1442 = Greater?(x=w2782, y=w2781) -> (0:w2778:bool)
            n1443 = And(x=w2782, y=w2781) -> (x .and. y?=w2783:u8)
            n1444 = Decrement(x=w2790) -> (x-1=w2777:u8)
            n1445 = Join Numbers(hi=w2783, lo=w2791) -> ((hi.lo)=w2789:u16)
            n1446 = Replace Array Subset(array=w2773, new element=w2784, index=w2777) -> (w2768:dbl[])
            n1447 = Replace Array Subset(array=w2776, new element=w2778, index=w2777) -> (w2774:bool[])
            "Discharge" <- w2774
            n1448 = Replace Array Subset(array=w2780, new element=w2789, index=w2777) -> (w2762:u16[])
            n1449 = Divide(x=w2768, y=10.0) -> (x/y=w2766:dbl[])
            "LV Temp" <- w2766
            n1450 = for {
              tunnel: [w2796] -> w2775 mode=indexing
              tunnel: w2762 -> [w2795] mode=indexing
              n1451 = Bundle(w2795, w2795) -> (w2796:cluster{u16, u16})  [unwired: 1 in]
            }
            "LV Battery" <- w2775
            n1452 = Array Subset(array=w2762, index=0, length=12) -> (w2765:u16[])
            n1453 = Array To Cluster(array=w2762) -> (cluster=→"LV Cell Voltages":T4)
            n1454 = Array Max & Min(array=w2766) -> (max value=→"LV Temp":dbl)  [unwired: 3 out]
            n1455 = Array Max & Min(array=w2765) -> (max value=→"LV Max":u16, min value=→"LV Min":u16)  [unwired: 2 out]
          }
          frame 1075 {
            n1456 = Index Array(array=w2803, index=2) -> (element=→"ASMS":u8)
          }
          frame 1377 {
            n1457 = Index Array(array=w2810, index=2) -> (element=→"Pedal Heartbeat":u8)
          }
          frame 1378 {
            # "Dashboard GPIO States"
            n1458 = Index Array(array=w2814, index=2) -> (element=→"Dash Heartbeat":u8)
            n1459 = Index Array(array=w2814, index=4) -> (element=w2831:u8)
            n1460 = Number To Boolean Array(number=w2831) -> (Boolean array=w2830:bool[])
            n1461 = Index Array(array=w2830, index #1=7 ("index"), index #2=6 ("index"), index #3=5 ("index"), index #4=4 ("index"), index #5=3 ("index"), index #6=2 ("index"), index #7=1 ("index"), index #8=0 ("index")) -> (element #3=→"OFF Button":bool, element #4=→"START Button":bool, element #5=→"ON Button":bool, element #6=→"BLANK":bool, element #7=→"XLAT":bool, element #8=→"MODE":bool)  [unwired: 2 out]
          }
          frame 1105 {
            n1462 = Index Array(array=w2840, index=2) -> (element=w2846:u8)
            n1463 = Index Array(array=w2840, index=3) -> (element=w2845:u8)
            n1464 = Index Array(array=w2840, index=4) -> (element=w2843:u8)
            n1465 = Index Array(array=w2840, index=5) -> (element=w2844:u8)
            n1466 = Join Numbers(hi=w2846, lo=w2845) -> ((hi.lo)=→"Wheel Travel FL":u16)
            n1467 = Join Numbers(hi=w2843, lo=w2844) -> ((hi.lo)=→"Wheel Travel FR":u16)
          }
          frame 1152 {
            n1468 = Array Subset(array=w2857, index=2, length=8) -> (→"CAN Missing Message":u8[])
          }
          frame 1153 {
            # "TCU Status 2"
            n1469 = call "read_TCUStatus2.vi"("Array"=w2876) -> ("output cluster"=w2875:T21)
            n1470 = Unbundle By Name(w2875) -> ("Yaw Control Balance"=→"Yaw Control":dbl, "M_Yaw_Limit [Nm]"=→"M_COG_Limit":u16, "M_Yaw [Nm]"=→"M Yaw [Nm]":i16, "Yaw Control Weight"=→"YawControlSelector":u16, "Brake Force Threshold"=→"Brake Force Threshold":u16, "Powlim Approx"=→"PowerLimiter Approx":u16, "Rear Reduction"=→"Rear_Reduction":dbl, "TC Normalizer"=→"TC Normalizer":u16, "Drop New"=→"New Drop":dbl, "Throttle Bias"=w2867:dbl)  [unwired: 1 out]
            "Throttle Bias Front" <- w2867
            n1471 = Subtract(x=1.0, y=w2867) -> (x-y=→"Throttle Bias Rear":dbl)
          }
          frame 1154 {
            n1472 = call "read_VDCInputErrors.vi"("Array"=w2927) -> ("output cluster"=w2926:T22)
            n1473 = Unbundle By Name(w2926) -> ("Sensorbox Front Timeout Error"=→"Sensorbox Front Timeout Error":bool, "Yaw Rate Rear Validity Error"=→"Yaw Rate Rear Validity Error":bool, "AccY Rear Validity Error"=→"AccY Rear Validity Error":bool, "AccX Rear Validity Error"=→"AccX Rear Validity Error":bool, "Sensorbox Front Timeout Error  2"=→"Sensorbox Front Timeout Error  2":bool, "Yaw Rate Front Validity Error"=→"Yaw Rate Front Validity Error":bool, "AccY Front Validity Error"=→"AccY Front Validity Error":bool, "AccX Front Validity Error"=→"AccX Front Validity Error":bool, "Steering Angle 1 Validity Error"=→"Steering Angle 1 Validity Error":bool, "Steering Angle Plausibility Error"=→"Steering Angle Plausibility Error":bool, "APPS2 Validity Error"=→"APPS2 Validity Error":bool, "APPS1 Validity Error"=→"APPS1 Validity Error":bool, "APPS Plausibility Error"=→"APPS Plausibility Error":bool, "Yaw Rate Plausibility Error"=→"Yaw Rate Plausibility Error":bool, "AccY Plausibility Error"=→"AccY Plausibility Error":bool, "AccX Plausibility Error"=→"AccX Plausibility Error":bool, "SC Endline Validity Error"=→"SC Endline Validity Error":bool, "Brake Pressure Timeout Error"=→"Brake Pressure Timeout Error":bool, "Brake Pressure Rear Validity Error"=→"Brake Pressure Rear Validity Error":bool, "Brake Pressure Front Validity Error"=→"Brake Pressure Front Validity Error":bool, "Brake Force Timeout Error"=→"Brake Force Timeout Error":bool, "Brake Force Validity Error"=→"Brake Force Validity Error":bool, "Steering APPS Timeout Error"=→"Steering APPS Timeout Error":bool, "Steering Angle 2 Validity Error"=→"Steering Angle 2 Validity Error":bool, "Button 2 Validity Error"=→"Button 2 Validity Error":bool, "Button 1 Validity Error"=→"Button 1 Validity Error":bool, "Rot Switch 5 Validity Error"=→"Rot Switch 5 Validity Error":bool, "Rot Switch 4 Validity Error"=→"Rot Switch 4 Validity Error":bool, "Rot Switch 3 Validity Error"=→"Rot Switch 3 Validity Error":bool, "Rot Switch 2 Validity Error"=→"Rot Switch 2 Validity Error":bool, "Rot Switch 1 Validity Error"=→"Rot Switch 1 Validity Error":bool, "SC Endline Timeout Error"=→"SC Endline Timeout Error":bool, "HV Voltage Validity Error"=→"HV Voltage Validity Error":bool, "HV Current Validity Error"=→"HV Current Validity Error":bool, "HV Cell Values Timeout Error"=→"HV Cell Values Timeout Error":bool, "HV Cell Voltage Validity Error"=→"HV Cell Voltage Validity Error":bool, "HV Cell Temperature Validity Error"=→"HV Cell Temperature Validity Error":bool, "Steering Control Timeout Error"=→"Steering Control Timeout Error":bool, "Button 4 Validity Error"=→"Button 4 Validity Error":bool, "Button 3 Validity Error"=→"Button 3 Validity Error":bool, "LV Cell Values Timeout Error"=→"LV Cell Values Timeout Error":bool, "LV Cell Voltage Validity Error"=→"LV Cell Voltage Validity Error":bool, "LV Cell Temperature Validity Error"=→"LV Cell Temperature Validity Error":bool, "HV Battery Status Timeout Error"=→"HV Battery Status Timeout Error":bool)
          }
          frame 1157 {
            n1474 = call "read_TCUStatus3.vi"("Array"=w2942) -> ("Message"=w2941:T23)
            n1475 = Unbundle By Name(w2941) -> ("Speed [kmph]"=→"Speed [kmph]":dbl, "Torque Demand [Nm]"=→"Torque Demand [Nm]":dbl, "Regbrake Front Sum [Nm]"=→"Regbrake Front Sum [Nm]":dbl, "Regbrake Rear Sum [Nm]"=→"Regbrake Rear Sum [Nm]":dbl, "Fz FL [N]"=→"Fz_FL":u16, "Fz FR [N]"=→"Fz_FR":u16, "Fz RL [N]"=→"Fz_RL":u16, "Fz RR [N]"=→"Fz_RR":u16)
          }
          frame 1158 {
            n1476 = call "read_TCUStatus4.vi"("Array"=w2953) -> ("Message"=w2952:T24)
            n1477 = Unbundle By Name(w2952) -> ("Efficiency Tune"=→"Tune":dbl, "TC Threshold"=→"TC Threshold":u8, "Launch Control Mu"=→"LaunchControl_Mu":dbl, "Brake Force Filtered"=→"BrakeForce":u16)
          }
          frame 1184 {
            # "Charger Status"
            n1478 = Index Array(array=w2967, index=3) -> (element=w2968:u8)
            n1479 = Number To Boolean Array(number=w2968) -> (Boolean array=w2966:bool[])
            n1480 = Index Array(array=w2966, index #1=7 ("index"), index #2=6 ("index"), index #3=5 ("index"), index #4=4 ("index"), index #5=3 ("index"), index #6=2 ("index"), index #7=1 ("index")) -> ()  [unwired: 7 out]
          }
          frame 1185 {
            # "Charger Status 2"
            n1481 = Index Array(array=w2991, index=8) -> (element=w2993:u8)
            n1482 = Index Array(array=w2991, index=9) -> (element=w2992:u8)
            n1483 = Index Array(array=w2991, index=2) -> (element=w3010:u8)
            n1484 = Index Array(array=w2991, index=3) -> (element=w3009:u8)
            n1485 = Index Array(array=w2991, index=6) -> (element=w2997:u8)
            n1486 = Index Array(array=w2991, index=7) -> (element=w2996:u8)
            n1487 = Index Array(array=w2991, index=4) -> (element=w3001:u8)
            n1488 = Index Array(array=w2991, index=5) -> (element=w3000:u8)
            n1489 = Join Numbers(hi=w2993, lo=w2992) -> ((hi.lo)=w2979:u16)
            n1490 = Join Numbers(hi=w3010, lo=w3009) -> ((hi.lo)=w2988:u16)
            n1491 = Join Numbers(hi=w2997, lo=w2996) -> ((hi.lo)=w2982:u16)
            n1492 = Join Numbers(hi=w3001, lo=w3000) -> ((hi.lo)=w2985:u16)
            n1493 = To Double Precision Float(number=w2979) -> (double precision float=w2980:dbl)
            n1494 = To Double Precision Float(number=w2988) -> (double precision float=w2989:dbl)
            n1495 = To Double Precision Float(number=w2982) -> (double precision float=w2983:dbl)
            n1496 = To Double Precision Float(number=w2985) -> (double precision float=w2986:dbl)
            n1497 = Divide(x=w2980, y=10.0) -> (x/y=→"Voltage Limit":dbl)
            n1498 = Divide(x=w2983, y=10.0) -> (x/y=→"Charge Voltage":dbl)
            n1499 = Divide(x=w2989, y=100.0) -> (x/y=→"Charge Curr":dbl)
            n1500 = Divide(x=w2986, y=100.0) -> (x/y=→"Current Limit":dbl)
          }
          frame 1638 {
            n1501 = Index Array(array=w3018, index=4) -> (element=w3024:u8)
            n1502 = Index Array(array=w3018, index=5) -> (element=w3023:u8)
            n1503 = Index Array(array=w3018, index=2) -> (element=w3028:u8)
            n1504 = Index Array(array=w3018, index=3) -> (element=w3027:u8)
            n1505 = Join Numbers(hi=w3024, lo=w3023) -> ((hi.lo)=w3021:u16)
            n1506 = Join Numbers(hi=w3028, lo=w3027) -> ((hi.lo)=w3022:u16)
            n1507 = To Word Integer(number=w3021) -> (16bit integer=→"PPS1":i16)
            n1508 = To Word Integer(number=w3022) -> (16bit integer=→"PPS2":i16)
          }
          frame 1639 {
            n1509 = Index Array(array=w3039, index=2) -> (element=w3051:u8)
            n1510 = Number To Boolean Array(number=w3051) -> (Boolean array=w3061:bool[])
            n1511 = Index Array(array=w3061, index #1=0 ("index"), index #2=1 ("index"), index #3=2 ("index"), index #4=3 ("index"), index #5=4 ("index"), index #6=5 ("index"), index #7=6 ("index"), index #8=7 ("index")) -> (element #1=w3050:bool, element #2=w3049:bool, element #3=w3048:bool, element #4=w3045:bool, element #5=w3044:bool, element #6=w3042:bool, element #7=w3041:bool, element #8=w3040:bool)
            n1512 = Build Array(w3050, w3049, w3048) -> (w3047:bool[])
            n1513 = Build Array(w3042, w3041, w3040) -> (w3043:bool[])
            n1514 = Build Array(w3045, w3044) -> (w3046:bool[])
            n1515 = Boolean Array To Number(Boolean array=w3047) -> (number=→"ASSI":u32)
            n1516 = Boolean Array To Number(Boolean array=w3046) -> (number=→"EBS":u32)
            n1517 = Boolean Array To Number(Boolean array=w3043) -> (number=→"AMI":u32)
          }
        }
      }
      n1518 = Empty Array?(array=w120) -> (empty?=w114:bool)
      n1519 = feedback-in #44(w114) -> ()
      n1520 = feedback #44(TRUE ("empty?")) -> (w116:bool)
      n1521 = Not(x=w116) -> (.not. x?=w118:bool)
      n1522 = And(x=w118, y=w114) -> (x .and. y?=w119:bool)
      n1523 = Not(x=w114) -> (.not. x?=w115:bool)
      n1524 = And(x=w116, y=w115) -> (x .and. y?=w117:bool)
      n1525 = case shown="True" w119 {
        frame False {
        }
        frame True {
          n1526 = property on="Tab Control" class="TabCtl (strict)"("FG Color"=u32 16711680 ("Colors:FG Color")) -> ()  [unwired: 2 in, 2 out]
        }
      }
      n1527 = case shown="True" w117 {
        frame False {
        }
        frame True {
          n1528 = property on="Tab Control" class="TabCtl (strict)"("FG Color"=u32 11776947 ("Colors:FG Color")) -> ()  [unwired: 2 in, 2 out]
        }
      }
      n1529 = flat-sequence {
        tunnel: w127 -> [w281]
        tunnel: w120 -> [w282]
        frame #0 {
          "CAN ID" <- w281
          "CAN Message" <- w282
          "CAN ID 2" <- w281
          "CAN Message 2" <- w282
          "CAN ID 3" <- w281
          "CAN Message 3" <- w282
        }
      }
    }
    n1530 = local read "Exit"() -> (w14:bool)
    n1531 = call <vilib>:"ncClose.vi"("Error in"=w7, "ObjHandle in"=w10) -> ()  [unwired: 1 in, 1 out]
    n1532 = call <vilib>:"ncClose.vi"("Error in"=w7, "ObjHandle in"=w9) -> ()  [unwired: 1 in, 1 out]
  }
  n1533 = node-c288(i64 100 ("Period")) -> (w3:T25)  [unwired: 3 in]
  n1534 = invoke class="VI" method="Default Vals.Reinit All"(reference=w4) -> ()  [unwired: 2 in, 3 out]
  n1535 = timed-loop {
    timing: w3 -> [_]
    timing-out: [_] -> w2
    stop <- _ stop-if-true
    w3070 = dbl[] []
    w3072 = 0.03
    n1536 = node-c288() -> ()  [unwired: 1 in, 1 out]
    n1537 = local read "Cones1 2"() -> (w3068:T1)
    n1538 = local read "Cones2 2"() -> (w3066:T1)
    n1539 = local read "Cones3 2"() -> (w3067:T1)
    n1540 = Build Array (concatenate)(w3068, w3066, w3067) -> (w3069:T1)
    n1541 = for {
      tunnel: w3069 -> [w3094] mode=indexing
      shift-right: [w3106] -> w3086
      shift-left: w3070 -> [w3100]
      shift-right: [w3105] -> w3084
      shift-left: w3070 -> [w3099]
      shift-right: [w3104] -> w3082
      shift-left: w3070 -> [w3098]
      shift-right: [w3102] -> w3080
      shift-left: w3070 -> [w3097]
      shift-right: [w3103] -> w3078
      shift-left: w3070 -> [w3096]
      shift-right: [w3101] -> w3076
      shift-left: w3070 -> [w3095]
      n1542 = Unbundle By Name(w3094) -> ("Cluster.Col"=w3107:dbl, "Cluster.X"=w3093:dbl, "Cluster.Y"=w3092:dbl)
      n1543 = To Unsigned Byte Integer(number=w3107) -> (unsigned 8bit integer=w3108:u8)
      n1544 = To Unsigned Long Integer(number=w3093) -> (unsigned 32bit integer=w3091:u32)
      n1545 = To Unsigned Long Integer(number=w3092) -> (unsigned 32bit integer=w3090:u32)
      n1546 = Not Equal To 0?(x=w3091) -> (x != 0?=w3088:bool)
      n1547 = Not Equal To 0?(x=w3090) -> (x != 0?=w3089:bool)
      n1548 = Or(x=w3088, y=w3089) -> (x .or. y?=w3087:bool)
      n1549 = case shown="True" w3087 {
        tunnel: w3108 -> [_ w3129]
        tunnel: w3093 -> [_ w3128]
        tunnel: w3092 -> [_ w3127]
        tunnel: [w3114 w3126] -> w3106
        tunnel: [w3113 w3125] -> w3105
        tunnel: [w3112 w3124] -> w3104
        tunnel: [w3110 w3123] -> w3103
        tunnel: [w3111 w3122] -> w3102
        tunnel: [w3109 w3121] -> w3101
        tunnel: w3100 -> [w3114 w3120]
        tunnel: w3099 -> [w3113 w3119]
        tunnel: w3098 -> [w3112 w3118]
        tunnel: w3097 -> [w3111 w3117]
        tunnel: w3096 -> [w3110 w3116]
        tunnel: w3095 -> [w3109 w3115]
        frame False {
        }
        frame True {
          n1550 = case shown="0" w3129 {
            tunnel: w3128 -> [_ w3143 w3153 w3163]
            tunnel: w3127 -> [_ w3142 w3152 w3162]
            tunnel: [w3135 w3145 w3149 w3159] -> w3126
            tunnel: [w3133 w3138 w3148 w3165] -> w3124
            tunnel: [w3134 w3139 w3155 w3158] -> w3125
            tunnel: [w3132 w3144 w3147 w3157] -> w3122
            tunnel: [w3130 w3136 w3146 w3164] -> w3121
            tunnel: [w3131 w3137 w3154 w3156] -> w3123
            tunnel: w3120 -> [w3135 w3141 w3149 w3159]
            tunnel: w3119 -> [w3134 w3139 w3151 w3158]
            tunnel: w3118 -> [w3133 w3138 w3148 w3161]
            tunnel: w3117 -> [w3132 w3140 w3147 w3157]
            tunnel: w3116 -> [w3131 w3137 w3150 w3156]
            tunnel: w3115 -> [w3130 w3136 w3146 w3160]
            frame 5, Default {
            }
            frame 1 {
              n1551 = Build Array (concatenate)(w3142, w3140) -> (w3144:dbl[])
              n1552 = Build Array (concatenate)(w3143, w3141) -> (w3145:dbl[])
            }
            frame 0 {
              n1553 = Build Array (concatenate)(w3152, w3150) -> (w3154:dbl[])
              n1554 = Build Array (concatenate)(w3153, w3151) -> (w3155:dbl[])
            }
            frame 2, 3 {
              n1555 = Build Array (concatenate)(w3162, w3160) -> (w3164:dbl[])
              n1556 = Build Array (concatenate)(w3163, w3161) -> (w3165:dbl[])
            }
          }
        }
      }
    }
    n1557 = call "Convert to Dynamic Data4"("Array"=w3080) -> ("Dynamic Data Type"=w3079:dynamicdata)  [unwired: 3 in]
    n1558 = call "Convert to Dynamic Data5"("Array"=w3078) -> ("Dynamic Data Type"=w3077:dynamicdata)  [unwired: 3 in]
    n1559 = call "Convert to Dynamic Data6"("Array"=w3076) -> ("Dynamic Data Type"=w3075:dynamicdata)  [unwired: 3 in]
    n1560 = call "Convert to Dynamic Data"("Array"=w3086) -> ("Dynamic Data Type"=w3085:dynamicdata)  [unwired: 3 in]
    n1561 = call "Convert to Dynamic Data2"("Array"=w3084) -> ("Dynamic Data Type"=w3083:dynamicdata)  [unwired: 3 in]
    n1562 = call "Convert to Dynamic Data3"("Array"=w3082) -> ("Dynamic Data Type"=w3081:dynamicdata)  [unwired: 3 in]
    n1563 = Merge Signals(w3079, w3077, w3075) -> (w3073:dynamicdata)
    n1564 = Merge Signals(w3085, w3083, w3081) -> (w3074:dynamicdata)
    n1565 = Multiply(x=w3072, y=w3073) -> (x*y=w3071:dynamicdata)
    n1566 = Multiply(x=w3074, y=w3072) -> (x*y=w3065:dynamicdata)
    n1567 = Decrement(x=w3065) -> (x-1=w3064:dynamicdata)
    n1568 = Decrement(x=w3064) -> (x-1=w3063:dynamicdata)
    n1569 = Decrement(x=w3063) -> (x-1=w3062:dynamicdata)
    n1570 = call "Build XY Graph"("Y Input"=w3062, "X Input"=w3071) -> ()  [unwired: 8 in, 2 out]
    n1571 = node-c288() -> ()  [unwired: 1 in, 1 out]
  }
  n1572 = node-c288(w2) -> ()  [unwired: 1 out]
